vi "EM9636M系列_主VI.vi"() -> ()   [LabVIEW 2016]
uses:
  <vilib>/Modbus/subvis/Modbus API/Modbus API.lvclass/Modbus API.ctl
  <vilib>/Modbus/subvis/Transmission Data Unit (ADU)/Transmission Data Unit/Transmission Data Unit.lvclass/Transmission Data Unit.ctl
  <vilib>/Modbus/master/Data Access/Unit ID/Set Unit ID Property.vi
  <vilib>/Modbus/subvis/Transmission Data Unit (ADU)/Transmission Data Unit/Data Access/Unit ID/Write Unit ID.vi
  <vilib>/Modbus/subvis/Modbus API/Read Transmission Data Unit.vi
  <vilib>/Modbus/subvis/Modbus API/Write Transmission Data Unit.vi
  <vilib>/Modbus/master/Modbus Master.lvclass
  <vilib>/Utility/NIReport.llb/Append Text Table to Report (wrap).vi
  <vilib>/Modbus/master/Create Master Instance (Serial).vi
  <vilib>/Modbus/subvis/Transmission Data Unit (ADU)/Transmission Data Unit/Transmission Data Unit.lvclass
  <vilib>/Utility/NIReport.llb/NI_report.lvclass
  <vilib>/ptbypt/NI_PtbyPt.lvlib
  <vilib>/Utility/miscctls.llb/LVRectTypeDef.ctl
panel:
  out "车型":string
  in  "簇 3":T1
  out "R3":dbl format="%#.2g"
  out "R2":dbl format="%#.2g"
  out "R1":dbl format="%#.2g"
  out "D6":dbl format="%#.2g"
  out "D5":dbl format="%#.2g"
  out "D4":dbl format="%#.2g"
  out "D3":dbl format="%#.2g"
  out "D2":dbl format="%#.2g"
  out "D1":dbl format="%#.2g"
  in  "簇":T1
  out "数据":T2(array[cluster])
  out "comcnt":u16
  out "对话框":bool
  out "到期了":bool
  out "变频6":bool
  out "变频5":bool
  out "变频4":bool
  out "变频3":bool
  out "变频2":bool
  out "变频1":bool
  in  "加载电机右下正反转":bool
  out "加载右下转矩监控":i16 format="%#.0f"
  in  "加载电机右下启动":bool caption="停止"
  out "加载电机右下母线电流":dbl
  out "加载电机右下母线电压":dbl
  out "加载转速右下监控":dbl
  in  "加载电机右下转速给定":i32
  in  "加载电机右下停机":bool caption="停止"
  out "加载电机右下运行？":bool
  in  "加载电机右下转矩给定":i16
  out "加载电机左下运行？":bool
  in  "加载电机左下转速给定":i32
  out "加载左下转速监控":dbl
  out "加载电机左下母线电压":dbl
  out "加载电机左下母线电流":dbl
  out "加载左下转矩监控":i16
  in  "加载电机左下停机":bool caption="停止"
  in  "加载电机左下启动":bool caption="停止"
  in  "加载电机左下正反转":bool
  in  "加载电机左下转矩给定":i16
  in  "加载电机右上正反转":bool
  out "加载转矩右上监控":i16 format="%#.0f"
  in  "加载电机右上启动":bool caption="停止"
  out "加载电机右上母线电流":dbl
  out "加载电机右上母线电压":dbl
  out "加载右上转速监控":dbl
  in  "加载电机右上转速给定":i32
  in  "加载电机右上停机":bool caption="停止"
  out "加载电机右上运行？":bool
  in  "加载电机右上转矩给定":i16
  out "加载电机左上运行？":bool
  in  "加载电机左上转速给定":i32
  out "加载左上转速监控":dbl
  out "加载电机左上母线电压":dbl
  out "加载电机左上母线电流":dbl
  out "加载左上转矩监控":i16
  in  "加载电机左上停机":bool caption="停止"
  in  "加载电机左上启动":bool caption="停止"
  in  "加载电机左上正反转":bool
  in  "加载电机左上转矩给定":i16
  in  "驱动电机上正反转":bool
  out "驱动转矩上监控":i16 format="%#.0f"
  in  "驱动电机上转矩给定":i16
  in  "驱动电机上启动":bool caption="停止"
  out "驱动电机上母线电流":dbl
  out "驱动电机上母线电压":dbl
  out "驱动上转速监控":dbl
  in  "驱动电机上转速给定":i16
  in  "驱动电机上停机":bool caption="停止"
  out "驱动电机上运行？":bool
  in  "驱动电机下正反转":bool
  out "驱动转矩下监控":i16 format="%#.0f"
  in  "驱动电机下转矩给定":i16
  in  "驱动电机下启动":bool caption="停止"
  out "驱动电机下母线电流":dbl
  out "驱动电机下母线电压":dbl
  out "驱动转速下监控":dbl
  in  "驱动电机转速下给定":i16
  in  "驱动电机下停机":bool caption="停止"
  out "驱动电机下运行？":bool
  out "轮询耗时":u32
  out "数值":i32
  out "对话框传递":bool
  out "超温报警":bool
  out "遥控器通讯":bool
  out "变频串口":bool
  in  "加载电机复位":bool caption="停止"
  out "变频器":bool
  out "前右":bool[](array[boolean])
  out "前左":bool[](array[boolean])
  out "中右":bool[](array[boolean])
  out "中左":bool[](array[boolean])
  out "后右":bool[](array[boolean])
  out "后左":bool[](array[boolean])
  in  "倒计时间S":dbl=600.0
  out "错误输出 7":errorcluster caption="错误输出"
  out "确认输入布尔":bool
  out "等待进车布尔":bool
  out "Config":T9={"DevType"=2, "DevIndex"=0, "CanIndex"=0, "VCI_INIT_CONFIG"={"AccCode"=0, "AccMask"=0, "InitFlag"=0, "Fliter"=0, "Timing0"=0, "Timing1"=0, "Mode"=0}} {"DevType" items=["USB-CAN"=3, "USB-CAN2"=4]; "CanIndex" items=["通道1", "通道2"]; "VCI_INIT_CONFIG"."Fliter" items=["接收所有类型"=3, "只接收标准帧"=4, "只接收扩展帧"=7]; "VCI_INIT_CONFIG"."Mode" items=["正常工作", "自测模式（环回）", "仅侦听模式"]; "VCI_INIT_CONFIG"."InitFlag" items=["使用Flash参数", "使用界面设置参数"]}
  in  "D1扭矩给定":i16=500
  in  "D2扭矩给定":i16=1000
  in  "D3扭矩给定":i16=1500
  in  "D4扭矩给定":i16=2000
  in  "D5扭矩给定":i16=3500
  in  "D6扭矩给定":i16=4000
  in  "R1扭矩给定":i16=500
  in  "R2扭矩给定":i16=1000
  in  "R3扭矩给定":i16=1500
  out "发送左侧字符":bool
  in  "Close":bool
  in  "Open 2":bool
  in  "AD开始采集 2":bool
  in  "AD开始采集":bool
  out "输出数组右":dbl[][](array[numeric])
  out "输出数组左":dbl[][](array[numeric])
  out "采集卡右":bool
  out "采集卡左":bool
  out "Open":bool
  out "close2":bool
  out "close":bool
  out "当前实验时间":string
  out "元素 2":bool
  out "元素":bool
  out "元素 4":bool
  out "元素 3":bool
  in  "速度温度":string[][](array[string]) caption="文本数据"
  out "实验基本信息":string[][](array[string])
  out "字符布尔":bool
  in  "Reset 9":bool caption="重置"
  in  "Reset 8":bool caption="重置"
  in  "Reset 7":bool caption="重置"
  in  "Reset 6":bool caption="重置"
  in  "Reset 5":bool caption="重置"
  in  "Reset 4":bool caption="重置"
  in  "Reset 3":bool caption="重置"
  in  "Reset 2":bool caption="重置"
  in  "Reset":bool caption="重置"
  out "R3平均速度":dbl
  out "R2平均速度":dbl
  out "R1平均速度":dbl
  out "D6平均速度":dbl
  out "D5平均速度":dbl
  out "D4平均速度":dbl
  out "D3平均速度":dbl
  out "D2平均速度":dbl
  out "平均速度数组":dbl[](array[numeric])
  out "D1平均速度":dbl
  out "停止布尔 2":bool
  out "停止布尔":bool
  out "启动布尔":bool
  out "485启动给遥控器布尔":bool
  in  "左5字符":u8=85 format="%x"
  in  "左4字符":u8=85 format="%x"
  in  "左3字符":u8=85 format="%x"
  in  "左2字符":u8=85 format="%x"
  in  "左1字符":u8=85 format="%x"
  out "布尔数组 2":bool[](array[boolean])
  out "布尔数组":bool[](array[boolean])
  in  "kBaudRate":u8(ring)=10 caption="波特率" items=["5k bps"=1, "10k bps"=2, "20k bps"=3, "40k bps"=4, "50k bps"=5, "80k bps"=6, "100k bps"=7, "125k bps"=8, "200k bps"=9, "250k bps"=10, "400k bps"=11, "500k bps"=12, "666k bps"=13, "800k bps"=14, "1000k bps"=15, "33.33k bps"=16, "66.66k bps"=17, "83.33k bps"=18]
  in  "Channel":T4 caption="CAN通道" items=["通道1", "通道2"]
  in  "DevType":T3=2 caption="设备类型" items=["USB-CAN"=2, "USB-CAN2"=3]
  out "中间数组":string[](array[string])
  in  "数值 2":dbl
  out "系统时间 2":string="系统时间"
  in  "ID_VCU_MCU_1 8":u32=522 format="0x%x"
  in  "ID_VCU_MCU_2 5":u32=522 format="0x%x"
  in  "ID_VCU_MCU_33 4":u32=522 format="0x%x"
  in  "ID_VCU_MCU_1 7":u32=522 format="0x%x"
  in  "0byte 13":u8=64 format="%x"
  in  "1byte 13":u8=6 format="%x"
  in  "2byte 13":u8=80 format="%x"
  in  "3byte 13":u8=111 format="%x"
  in  "4byte 13":u8=119 format="%x"
  in  "5byte 13":u8=101 format="%x"
  in  "6byte 13":u8=114 format="%x"
  in  "7byte 13":u8=32 format="%x"
  in  "0byte 14":u8=70 format="%x"
  in  "1byte 14":u8=2 format="%x"
  in  "2byte 14":u8=32 format="%x"
  in  "3byte 14":u8=32 format="%x"
  in  "4byte 14":u8 format="%x"
  in  "5byte 14":u8 format="%x"
  in  "6byte 14":u8 format="%x"
  in  "7byte 14":u8 format="%x"
  in  "0byte 15":u8=96 format="%x"
  in  "1byte 15":u8=6 format="%x"
  in  "2byte 15":u8=84 format="%x"
  in  "3byte 15":u8=85 format="%x"
  in  "4byte 15":u8=114 format="%x"
  in  "5byte 15":u8=113 format="%x"
  in  "6byte 15":u8=117 format="%x"
  in  "7byte 15":u8=101 format="%x"
  in  "0byte 16":u8=102 format="%x"
  in  "1byte 16":u8=2 format="%x"
  in  "2byte 16":u8=32 format="%x"
  in  "3byte 16":u8=32 format="%x"
  in  "4byte 16":u8 format="%x"
  in  "5byte 16":u8 format="%x"
  in  "6byte 16":u8 format="%x"
  in  "7byte 16":u8 format="%x"
  in  "ID_VCU_MCU_1 6":u32=522 format="0x%x"
  in  "ID_VCU_MCU_2 4":u32=522 format="0x%x"
  in  "ID_VCU_MCU_33 3":u32=522 format="0x%x"
  in  "ID_VCU_MCU_1 5":u32=522 format="0x%x"
  in  "0byte 5":u8=16 format="%x"
  in  "1byte 5":u8=6 format="%x"
  in  "2byte 5":u8=85 format="%x"
  in  "3byte 5":u8=85 format="%x"
  in  "4byte 5":u8=85 format="%x"
  in  "5byte 5":u8=85 format="%x"
  in  "6byte 5":u8=85 format="%x"
  in  "7byte 5":u8=85 format="%x"
  in  "0byte 6":u8=86 format="%x"
  in  "1byte 6":u8=2 format="%x"
  in  "2byte 6":u8=75 format="%x"
  in  "3byte 6":u8=119 format="%x"
  in  "4byte 6":u8 format="%x"
  in  "5byte 6":u8 format="%x"
  in  "6byte 6":u8 format="%x"
  in  "7byte 6":u8 format="%x"
  in  "0byte 7":u8=48 format="%x"
  in  "1byte 7":u8=6 format="%x"
  in  "2byte 7":u8=85 format="%x"
  in  "3byte 7":u8=85 format="%x"
  in  "4byte 7":u8=85 format="%x"
  in  "5byte 7":u8=85 format="%x"
  in  "6byte 7":u8=85 format="%x"
  in  "7byte 7":u8=85 format="%x"
  in  "0byte 8":u8=118 format="%x"
  in  "1byte 8":u8=2 format="%x"
  in  "2byte 8":u8=78 format="%x"
  in  "3byte 8":u8=109 format="%x"
  in  "4byte 8":u8 format="%x"
  in  "5byte 8":u8 format="%x"
  in  "6byte 8":u8 format="%x"
  in  "7byte 8":u8 format="%x"
  in  "ID_VCU_MCU_1 2":u32=522 format="0x%x"
  in  "ID_VCU_MCU_33":u32=522 format="0x%x"
  in  "ID_VCU_MCU_2 2":u32=522 format="0x%x"
  in  "ID_VCU_MCU_1":u32=522 format="0x%x"
  in  "ID_VCU_MCU_1 4":u32=522 format="0x%x"
  in  "ID_VCU_MCU_2 3":u32=522 format="0x%x"
  in  "ID_VCU_MCU_33 2":u32=522 format="0x%x"
  in  "ID_VCU_MCU_1 3":u32=522 format="0x%x"
  in  "0byte 9":u8 format="%x"
  in  "1byte 9":u8=6 format="%x"
  in  "2byte 9":u8=71 format="%x"
  in  "3byte 9":u8=101 format="%x"
  in  "4byte 9":u8=97 format="%x"
  in  "5byte 9":u8=114 format="%x"
  in  "6byte 9":u8=32 format="%x"
  in  "7byte 9":u8=32 format="%x"
  in  "0byte 10":u8=6 format="%x"
  in  "1byte 10":u8=2 format="%x"
  in  "2byte 10":u8=32 format="%x"
  in  "3byte 10":u8=32 format="%x"
  in  "4byte 10":u8 format="%x"
  in  "5byte 10":u8 format="%x"
  in  "6byte 10":u8 format="%x"
  in  "7byte 10":u8 format="%x"
  in  "0byte 11":u8=32 format="%x"
  in  "1byte 11":u8=6 format="%x"
  in  "2byte 11":u8=83 format="%x"
  in  "3byte 11":u8=112 format="%x"
  in  "4byte 11":u8=101 format="%x"
  in  "5byte 11":u8=101 format="%x"
  in  "6byte 11":u8=100 format="%x"
  in  "7byte 11":u8=32 format="%x"
  in  "0byte 12":u8=38 format="%x"
  in  "1byte 12":u8=2 format="%x"
  in  "2byte 12":u8=32 format="%x"
  in  "3byte 12":u8=32 format="%x"
  in  "4byte 12":u8 format="%x"
  in  "5byte 12":u8 format="%x"
  in  "6byte 12":u8 format="%x"
  in  "7byte 12":u8 format="%x"
  in  "0byte 4":u8=54 format="%x"
  in  "1byte 4":u8=2 format="%x"
  in  "2byte 4":u8=80 format="%x"
  in  "3byte 4":u8=109 format="%x"
  in  "4byte 4":u8 format="%x"
  in  "5byte 4":u8 format="%x"
  in  "6byte 4":u8 format="%x"
  in  "7byte 4":u8 format="%x"
  in  "0byte 3":u8=48 format="%x"
  in  "1byte 3":u8=6 format="%x"
  in  "2byte 3":u8=85 format="%x"
  in  "3byte 3":u8=85 format="%x"
  in  "4byte 3":u8=85 format="%x"
  in  "5byte 3":u8=85 format="%x"
  in  "6byte 3":u8=85 format="%x"
  in  "7byte 3":u8=82 format="%x"
  in  "0byte 2":u8=22 format="%x"
  in  "1byte 2":u8=2 format="%x"
  in  "2byte 2":u8=32 format="%x"
  in  "3byte 2":u8=32 format="%x"
  in  "4byte 2":u8 format="%x"
  in  "5byte 2":u8 format="%x"
  in  "6byte 2":u8 format="%x"
  in  "7byte 2":u8 format="%x"
  out "选项卡控件 4":enum32{"VCU控制", "CAN基本操作"}(tab)
  in  "Clear":bool
  in  "Mode":T8 caption="工作模式" items=["正常工作", "仅侦听模式", "自测模式（环回）"]
  in  "Fliter":T7=1 items=["接收所有类型"=1, "只接收标准帧"=2, "只接收扩展帧"=3]
  in  "AccMask":u32=4294967295 caption="接收屏蔽码" format="%08x"
  in  "AccCode":u32 caption="接收过滤码" format="%08x"
  out "SendCnt":u32 caption="发送统计"
  out "RecvCnt":u32 caption="接收统计"
  in  "RcvEnable":bool=TRUE
  in  "list":i32(listbox)
  in  "Send":bool
  in  "ID":u32 format="0x%x"
  in  "Type":u8(ring) items=["数据帧", "远程帧"]
  in  "Format":u8(ring) items=["标准帧", "扩展帧"]
  in  "Data":string="01 00"
  in  "0byte":u8=16 format="%x"
  in  "1byte":u8=6 format="%x"
  in  "2byte":u8=85 format="%x"
  in  "3byte":u8=85 format="%x"
  in  "4byte":u8=85 format="%x"
  in  "5byte":u8=85 format="%x"
  in  "6byte":u8=85 format="%x"
  in  "7byte":u8=85 format="%x"
  in  "InitFlag":T6=1 caption="初始化参数" items=["使用Flash参数", "使用界面设置参数"]
  in  "选项卡控件 3":enum32{"数据监视", "查看数据"}(tab)
  in  "确认换挡":bool
  in  "重新选档档位":T10(ring)
  out "前右":bool
  out "中右":bool
  out "后右":bool
  out "前左":bool
  out "中左":bool
  out "后左":bool
  out "R3S":dbl format="%#.2g"
  out "R2S":dbl format="%#.2g"
  out "R1S":dbl format="%#.2g"
  out "D6S":dbl format="%#.2g"
  out "D5S":dbl format="%#.2g"
  out "D4S":dbl format="%#.2g"
  out "D3S":dbl format="%#.2g"
  out "D2S":dbl format="%#.2g"
  out "D1S":dbl format="%#.2g"
  in  "刷新参数":bool
  out "LED屏幕信息":string
  in  "高级参数":bool
  in  "重新实验":bool
  in  "生成报表":bool
  in  "确认输入":bool
  in  "遥控器按钮确认":bool
  out "总实验时间":string
  out "前右":dbl format="%#.2g"
  out "前左":dbl format="%#.2g"
  out "中右":dbl
  out "中左":dbl format="%#.2g"
  out "后右":dbl format="%#.2g"
  out "后左":dbl format="%#.2g"
  out "后右":dbl format="%#.2g"
  out "后左":dbl format="%#.2g"
  out "中右":dbl format="%#.2g"
  out "中左":dbl format="%#.2g"
  out "前右":dbl format="%#.2g"
  out "前左":dbl format="%#.2g"
  out "环境温度标定":dbl format="%#.2g"
  out "波形图表":dynamicdata(graph)
  in  "操作者":string
  out "加载扭矩N.M(单个）":dbl
  out "当前试验档位":string
  in  "试验车型":u16(ring) items=["SG21-3", "SG14", "SG16-3", "SG18-3"]
  out "车速":dbl(knob) scale=-30.0..30.0
  in  "试验车编号":string
  in  "发动机编号":string
  out "加载功率":dbl(knob) scale=0.0..30.0
  in  "试验开始":bool caption="停止"
  in  "停止":bool
  out "液压油箱温度标定":dbl format="%#.2g"
  out "变矩器出口温度标定":dbl format="%#.2g"
  out "右前轮轴承温度标定":dbl format="%#.2g"
  out "左前轮轴承温度标定":dbl format="%#.2g"
  out "振动泵压力":dbl format="%#.2g"
  out "转向泵压力":dbl format="%#.2g"
  in  "密码输入":string
  out "SG14百分比":dbl
  out "SG16-3百分比":dbl
  out "SG18-3百分比":dbl
  out "D1 act":dbl format="%#.2g"
  out "D2 act":dbl format="%#.2g"
  out "R3 act":dbl format="%#.2g"
  out "R2 act":dbl format="%#.2g"
  out "R1 act":dbl format="%#.2g"
  out "D6 act":dbl format="%#.2g"
  out "D5 act":dbl format="%#.2g"
  out "D4 act":dbl format="%#.2g"
  out "D3 act":dbl format="%#.2g"
  out "数值 3":i32
  out "前右电机右轴承振动":dbl
  out "前右电机左轴承振动":dbl
  out "前右滚筒右轴承振动":dbl
  out "前右滚筒左轴承振动":dbl
  out "后左滚筒右振动":dbl
  out "后左滚筒左振动":dbl
  out "中右电机右振动":dbl
  out "中右电机左振动":dbl
  out "中右滚筒右振动":dbl
  out "中右滚筒左振动":dbl
  out "中左电机右轴承振动":dbl
  out "中左电机左轴承振动":dbl
  out "中左滚筒右轴承振动":dbl
  out "中左滚筒左轴承振动":dbl
  out "前左电机右轴承振动":dbl
  out "前左电机左轴承振动":dbl
  out "前左滚筒右轴承振动":dbl
  out "前左滚筒左轴承振动":dbl
  out "后右电机右振动":dbl
  out "后右电机左振动":dbl
  out "后右滚筒右振动":dbl
  out "后右滚筒左振动":dbl
  out "后左电机右振动":dbl
  out "后左电机左振动":dbl
  out "后右电机绕组":dbl
  out "后右电机右轴承":dbl
  out "后右滚筒左轴承":dbl
  out "后左滚筒右轴承":dbl
  out "后右滚筒左轴承":dbl
  out "后左电机绕组":dbl
  out "后左电机右轴承":dbl
  out "后左电机左轴承":dbl
  out "后左滚筒右轴承":dbl
  out "后左滚筒左轴承":dbl
  out "中右电机绕组":dbl
  out "中右电机右轴承":dbl
  out "中右电机左轴承":dbl
  out "中右滚筒右轴承":dbl
  out "中右滚筒左轴承":dbl
  out "中左电机绕组":dbl
  out "中左电机右轴承":dbl
  out "中左电机左轴承":dbl
  out "中左滚筒右轴承":dbl
  out "中左滚筒左轴承":dbl
  out "前右电机绕组":dbl
  out "前右电机右轴承":dbl
  out "前右滚筒左轴承":dbl
  out "前左滚筒右轴承":dbl
  out "前右滚筒左轴承":dbl
  out "前左电机绕组":dbl
  out "前左电机右轴承":dbl
  out "前左电机左轴承":dbl
  out "前左滚筒右轴承":dbl
  out "前左滚筒左轴承":dbl
  out "错误输出 6":errorcluster caption="错误输出"
  out "AD均值数据 2":dbl[](array[numeric])
  in  "M系列PWM停止 2":bool
  in  "编码器清零 2":bool
  in  "DA输出 2":bool
  in  "DA输出范围 2":i32(ring) items=["±10V", "±5V", "0~10V（默认）", "0~5V", "0~20mA"]
  in  "CH1 2":i16(slide) scale=0.0..10000.0
  in  "CH3 2":i16(slide) scale=0.0..10000.0
  in  "CH4 2":i16(slide) scale=0.0..10000.0
  in  "CH2 2":i16(slide) scale=0.0..10000.0
  in  "设定输出脉冲个数 2":u32
  in  "M系列PWM输出 2":bool
  in  "AD停止采集 2":bool
  out "布尔 2":bool
  in  "通道频率Hz 2":dbl=10000.0 min=1000.0 max=100000.0 step=10.0
  in  "组频率Hz 2":dbl=500.0
  in  "单双端 2":i32(ring) items=["单端", "双端"]
  in  "AD终止通道 2":i32=32
  in  "AD起始通道 2":i32=1
  in  "增益 2":i32(ring) items=["无增益", "2倍增益", "5倍增益", "10倍增益"]
  in  "伪同步 2":i32(ring) items=["非伪同步", "伪同步"]
  in  "时钟源 2":i32(ring) items=["内时钟", "外时钟"]
  out "每次总数据量 2":i32
  out "通道数量 2":i32
  in  "AD范围 2":enum16{"-10~+10V", "-5V~+5V", "0~10V", "0~5V"}(ring)=enum."0~10V"
  out "每通道数据量 2":i32
  out "编码器AB值 2":i32[](array[numeric])
  out "编码器过零值 2":i16[](array[numeric])
  out "错误输出 5":errorcluster caption="错误输出3"
  out "错误输出 4":errorcluster caption="错误输出2"
  out "设备句柄 2":i32=1
  in  "选项卡控件 2":enum32{"AD数值显示", "数字量I/O", "(标准)PWM", "计数器（测频）"}(tab)
  in  "设置开关量方向 3":bool
  out "数组 5":dbl[](array[numeric])=[1.0, 2.0, 3.0, 4.0, 5.0, 6.0, 7.0, 8.0]
  out "数组 6":dbl[](array[numeric])=[1.0, 2.0, 3.0, 4.0, 5.0, 6.0, 7.0, 8.0]
  in  "光隔离输出 2":bool[](array[boolean])=[FALSE, FALSE, FALSE, FALSE, FALSE, FALSE, FALSE, FALSE]
  out "光隔离输入 2":bool[](array[boolean])
  in  "设置开关量方向 2":cluster{"IO1~IO8":i8, "IO9~IO16":i8}={"IO1~IO8"=1, "IO9~IO16"=1} {"IO9~IO16" items=["输入", "输出"]; "IO1~IO8" items=["输入", "输出"]}
  out "数组 7":i8[](array[numeric])
  in  "可编程数字量I/O 2":T11
  out "可编程数字量I/O(映射控件)--得到所有通道开关量值 2":T11
  in  "PWM输出 2":bool
  in  "PWM停止 2":bool
  in  "频率1 2":dbl=1000.0
  in  "占空比(0~1) 6":dbl=0.5
  out "实际频率 6":dbl
  out "实际占空比 6":dbl
  in  "频率2 2":dbl=5000.0
  in  "占空比(0~1) 5":dbl=0.5
  out "实际频率 5":dbl
  out "实际占空比 5":dbl
  in  "频率3 2":dbl=100000.0
  in  "占空比(0~1) 4":dbl=0.5
  out "实际频率 4":dbl
  out "实际占空比 4":dbl
  in  "开启计数 2":bool
  in  "计数器清零 2":bool
  in  "工作方式 2":u16(ring)=1 items=["计数", "测频"]
  out "计数/测频（Hz）值 2":dbl[](array[numeric])
  in  "编码器清零":bool
  out "编码器AB值":i32[](array[numeric])
  out "编码器过零值":i16[](array[numeric])
  in  "设定输出脉冲个数":u32
  in  "M系列PWM输出":bool
  in  "M系列PWM停止":bool
  in  "CH4":i16(slide) scale=0.0..10000.0
  in  "CH3":i16(slide) scale=0.0..10000.0
  in  "CH2":i16(slide) scale=0.0..10000.0
  in  "CH1":i16(slide) scale=0.0..10000.0
  in  "DA输出":bool
  in  "DA输出范围":i32(ring) items=["±10V", "±5V", "0~10V（默认）", "0~5V", "0~20mA"]
  out "每通道数据量":i32
  out "AD均值数据":dbl[](array[numeric])
  out "布尔":bool
  in  "AD停止采集":bool
  out "错误输出 3":errorcluster caption="错误输出3"
  out "错误输出 2":errorcluster caption="错误输出2"
  in  "选项卡控件":enum32{"AD数值显示", "数字量I/O", "(标准)PWM", "计数器（测频）"}(tab)
  out "变频故障1":bool
  out "变频故障2":bool
  out "变频故障 3":bool
  out "变频故障 4":bool
  out "变频故障5":bool
  out "变频故障 6":bool
  in  "设置开关量方向":bool
  out "数组 3":dbl[](array[numeric])=[1.0, 2.0, 3.0, 4.0, 5.0, 6.0, 7.0, 8.0]
  out "数组 2":dbl[](array[numeric])=[1.0, 2.0, 3.0, 4.0, 5.0, 6.0, 7.0, 8.0]
  in  "光隔离输出":bool[](array[boolean])=[FALSE, FALSE, FALSE, FALSE, FALSE, FALSE, FALSE, FALSE]
  out "光隔离输入":bool[](array[boolean])
  in  "设置开关量方向":cluster{"IO1~IO8":i8, "IO9~IO16":i8}={"IO1~IO8"=1, "IO9~IO16"=1} {"IO9~IO16" items=["输入", "输出"]; "IO1~IO8" items=["输入", "输出"]}
  out "数组 4":i8[](array[numeric])
  in  "可编程数字量I/O":T11
  out "可编程数字量I/O(映射控件)--得到所有通道开关量值":T11
  in  "PWM输出":bool
  in  "PWM停止":bool
  in  "频率1":dbl=1000.0
  in  "占空比(0~1)":dbl=0.5
  out "实际频率":dbl
  out "实际占空比":dbl
  in  "频率2":dbl=5000.0
  in  "占空比(0~1) 2":dbl=0.5
  out "实际频率 2":dbl
  out "实际占空比 2":dbl
  in  "频率3":dbl=100000.0
  in  "占空比(0~1) 3":dbl=0.5
  out "实际频率 3":dbl
  out "实际占空比 3":dbl
  in  "开启计数":bool
  in  "计数器清零":bool
  in  "工作方式":u16(ring)=1 items=["计数", "测频"]
  out "计数/测频（Hz）值":dbl[](array[numeric])
  in  "AD范围":enum16{"-10~+10V", "-5V~+5V", "0~10V", "0~5V"}(ring)=enum."0~10V"
  out "通道数量":i32
  out "设备句柄":i32=1
  out "错误输出":errorcluster
  out "每次总数据量":i32
  in  "时钟源":i32(ring) items=["内时钟", "外时钟"]
  in  "伪同步":i32(ring) items=["非伪同步", "伪同步"]
  in  "增益":i32(ring) items=["无增益", "2倍增益", "5倍增益", "10倍增益"]
  in  "AD起始通道":i32=1
  in  "AD终止通道":i32=32
  in  "单双端":i32(ring) items=["单端", "双端"]
  in  "组频率Hz":dbl=500.0
  in  "通道频率Hz":dbl=10000.0 min=1000.0 max=100000.0 step=10.0
  in  "数据端口":i32=8001
  in  "命令端口":i32=8000
  in  "IP地址":string="192.168.1.125"
  # "加载电机右上"
  # "驱动电机上"
  # "加载电机左上"
  # "r/min"
  # "r/min"
  # "r/min"
  # "转速"
  # "给定"
  # "转速"
  # "给定"
  # "转速"
  # "给定"
  # "给定"
  # "Nm"
  # "Nm"
  # "Nm"
  # "转矩"
  # "转矩"
  # "给定"
  # "转矩"
  # "给定"
  # "山推平地机实验台"
  # "电压"
  # "电流"
  # "电压"
  # "电流"
  # "电压"
  # "V"
  # "电流"
  # "A"
  # "A"
  # "V"
  # "A"
  # "V"
  # "遥控器"
  # "变频器"
  # "采集卡左"
  # "采集卡右"
  # "超温报警"
  # "正转"
  # "反转"
  # "正转"
  # "正转"
  # "反转"
  # "反转"
  # "加载电机右下"
  # "驱动电机下"
  # "加载电机左下"
  # "r/min"
  # "r/min"
  # "r/min"
  # "转速"
  # "给定"
  # "转速"
  # "给定"
  # "转速"
  # "给定"
  # "给定"
  # "Nm"
  # "Nm"
  # "Nm"
  # "转矩"
  # "转矩"
  # "给定"
  # "转矩"
  # "给定"
  # "电压"
  # "电流"
  # "电压"
  # "电流"
  # "电压"
  # "V"
  # "电流"
  # "A"
  # "V"
  # "A"
  # "V"
  # "A"
  # "正转"
  # "反转"
  # "正转"
  # "正转"
  # "反转"
  # "反转"
  # "D1"
  # "D6扭矩给定"
  # "~"
  # "R1"
  # "R3扭矩给定"
  # "~"
  # "EM9636M系列--LabView例程"
  # "CH1"
  # "CH2"
  # "如果设为0，则表示连续输出"
  # "CH1"
  # "CH2"
  # "位置传感器故障"
  # "过流"
  # "控制器过温"
  # "电机过温"
  # "欠压报警"
  # "过压报警"
  # "通讯故障"
  # "控制器高温"
  # "短路保护"
  # "严重欠压"
  # "超过峰值功率"
  # "超过最高限速"
  # "VCU故障"
  # "跛行状态"
  # "堵转保护"
  # "致命故障"
  # "车辆参数"
  # "设备参数"
  # "环境温度"
  # "前左"
  # "℃"
  # "℃"
  # "r/min"
  # "r/min"
  # "r/min"
  # "液压油箱温度"
  # "℃"
  # "前右"
  # "℃"
  # "r/min"
  # "r/min"
  # "r/min"
  # "变速箱温度"
  # "℃"
  # "中左"
  # "℃"
  # "右前轮轴承温度"
  # "中右"
  # "℃"
  # "℃"
  # "左前轮轴承温度"
  # "~"
  # "D1   R3/%"
  # "℃"
  # "后左"
  # "℃"
  # "~"
  # "D1   R3/S"
  # "Mp"
  # "工作泵压力"
  # "后右"
  # "℃"
  # "转向泵压力"
  # "Mp"
  # "前左滚筒左轴承"
  # "后左滚筒左轴承"
  # "℃"
  # "℃"
  # "后左电机左振动"
  # "前右滚筒左振动"
  # "前左滚筒右轴承"
  # "后左滚筒右轴承"
  # "℃"
  # "℃"
  # "后左电机右振动"
  # "前右滚筒右振动"
  # "前左电机左轴承"
  # "后左电机左轴承"
  # "℃"
  # "后右滚筒左振动"
  # "℃"
  # "前右电机左振动"
  # "前左电机右轴承"
  # "后左电机右轴承"
  # "℃"
  # "℃"
  # "后右滚筒右振动"
  # "前右电机右振动"
  # "前左电机绕组"
  # "后左电机绕组"
  # "后右电机左振动"
  # "℃"
  # "℃"
  # "前右滚筒左轴承"
  # "后右滚筒左轴承"
  # "后右电机右振动"
  # "℃"
  # "℃"
  # "前右滚筒右轴承"
  # "后右滚筒右轴承"
  # "前左滚筒左振动"
  # "℃"
  # "℃"
  # "前右电机左轴承"
  # "后右电机左轴承"
  # "前右滚筒右振动"
  # "℃"
  # "℃"
  # "前右电机右轴承"
  # "后右电机右轴承"
  # "前左电机左振动"
  # "℃"
  # "℃"
  # "前右电机绕组"
  # "后右电机绕组"
  # "℃"
  # "℃"
  # "前左电机右振动"
  # "中左滚筒左轴承"
  # "℃"
  # "中左滚筒左振动"
  # "中左滚筒右轴承"
  # "℃"
  # "中左滚筒右振动"
  # "中左电机左轴承"
  # "中左电机左振动"
  # "℃"
  # "中左电机右轴承"
  # "℃"
  # "中左电机右振动"
  # "中左电机绕组"
  # "℃"
  # "中右滚筒左振动"
  # "中右滚筒左轴承"
  # "中右滚筒右振动"
  # "℃"
  # "中右滚筒右轴承"
  # "中右电机左振动"
  # "℃"
  # "中右电机左轴承"
  # "中右电机右振动"
  # "℃"
  # "中右电机右轴承"
  # "后左滚筒左振动"
  # "℃"
  # "中右电机绕组"
  # "℃"
  # "后左滚筒右振动"
  # "通道3"
  # "通道1"
  # "通道2"
  # "频率，250Hz~500KHz\n占空比，0~1"
  # "通道3"
  # "通道1"
  # "通道2"
  # "频率，250Hz~500KHz\n占空比，0~1"
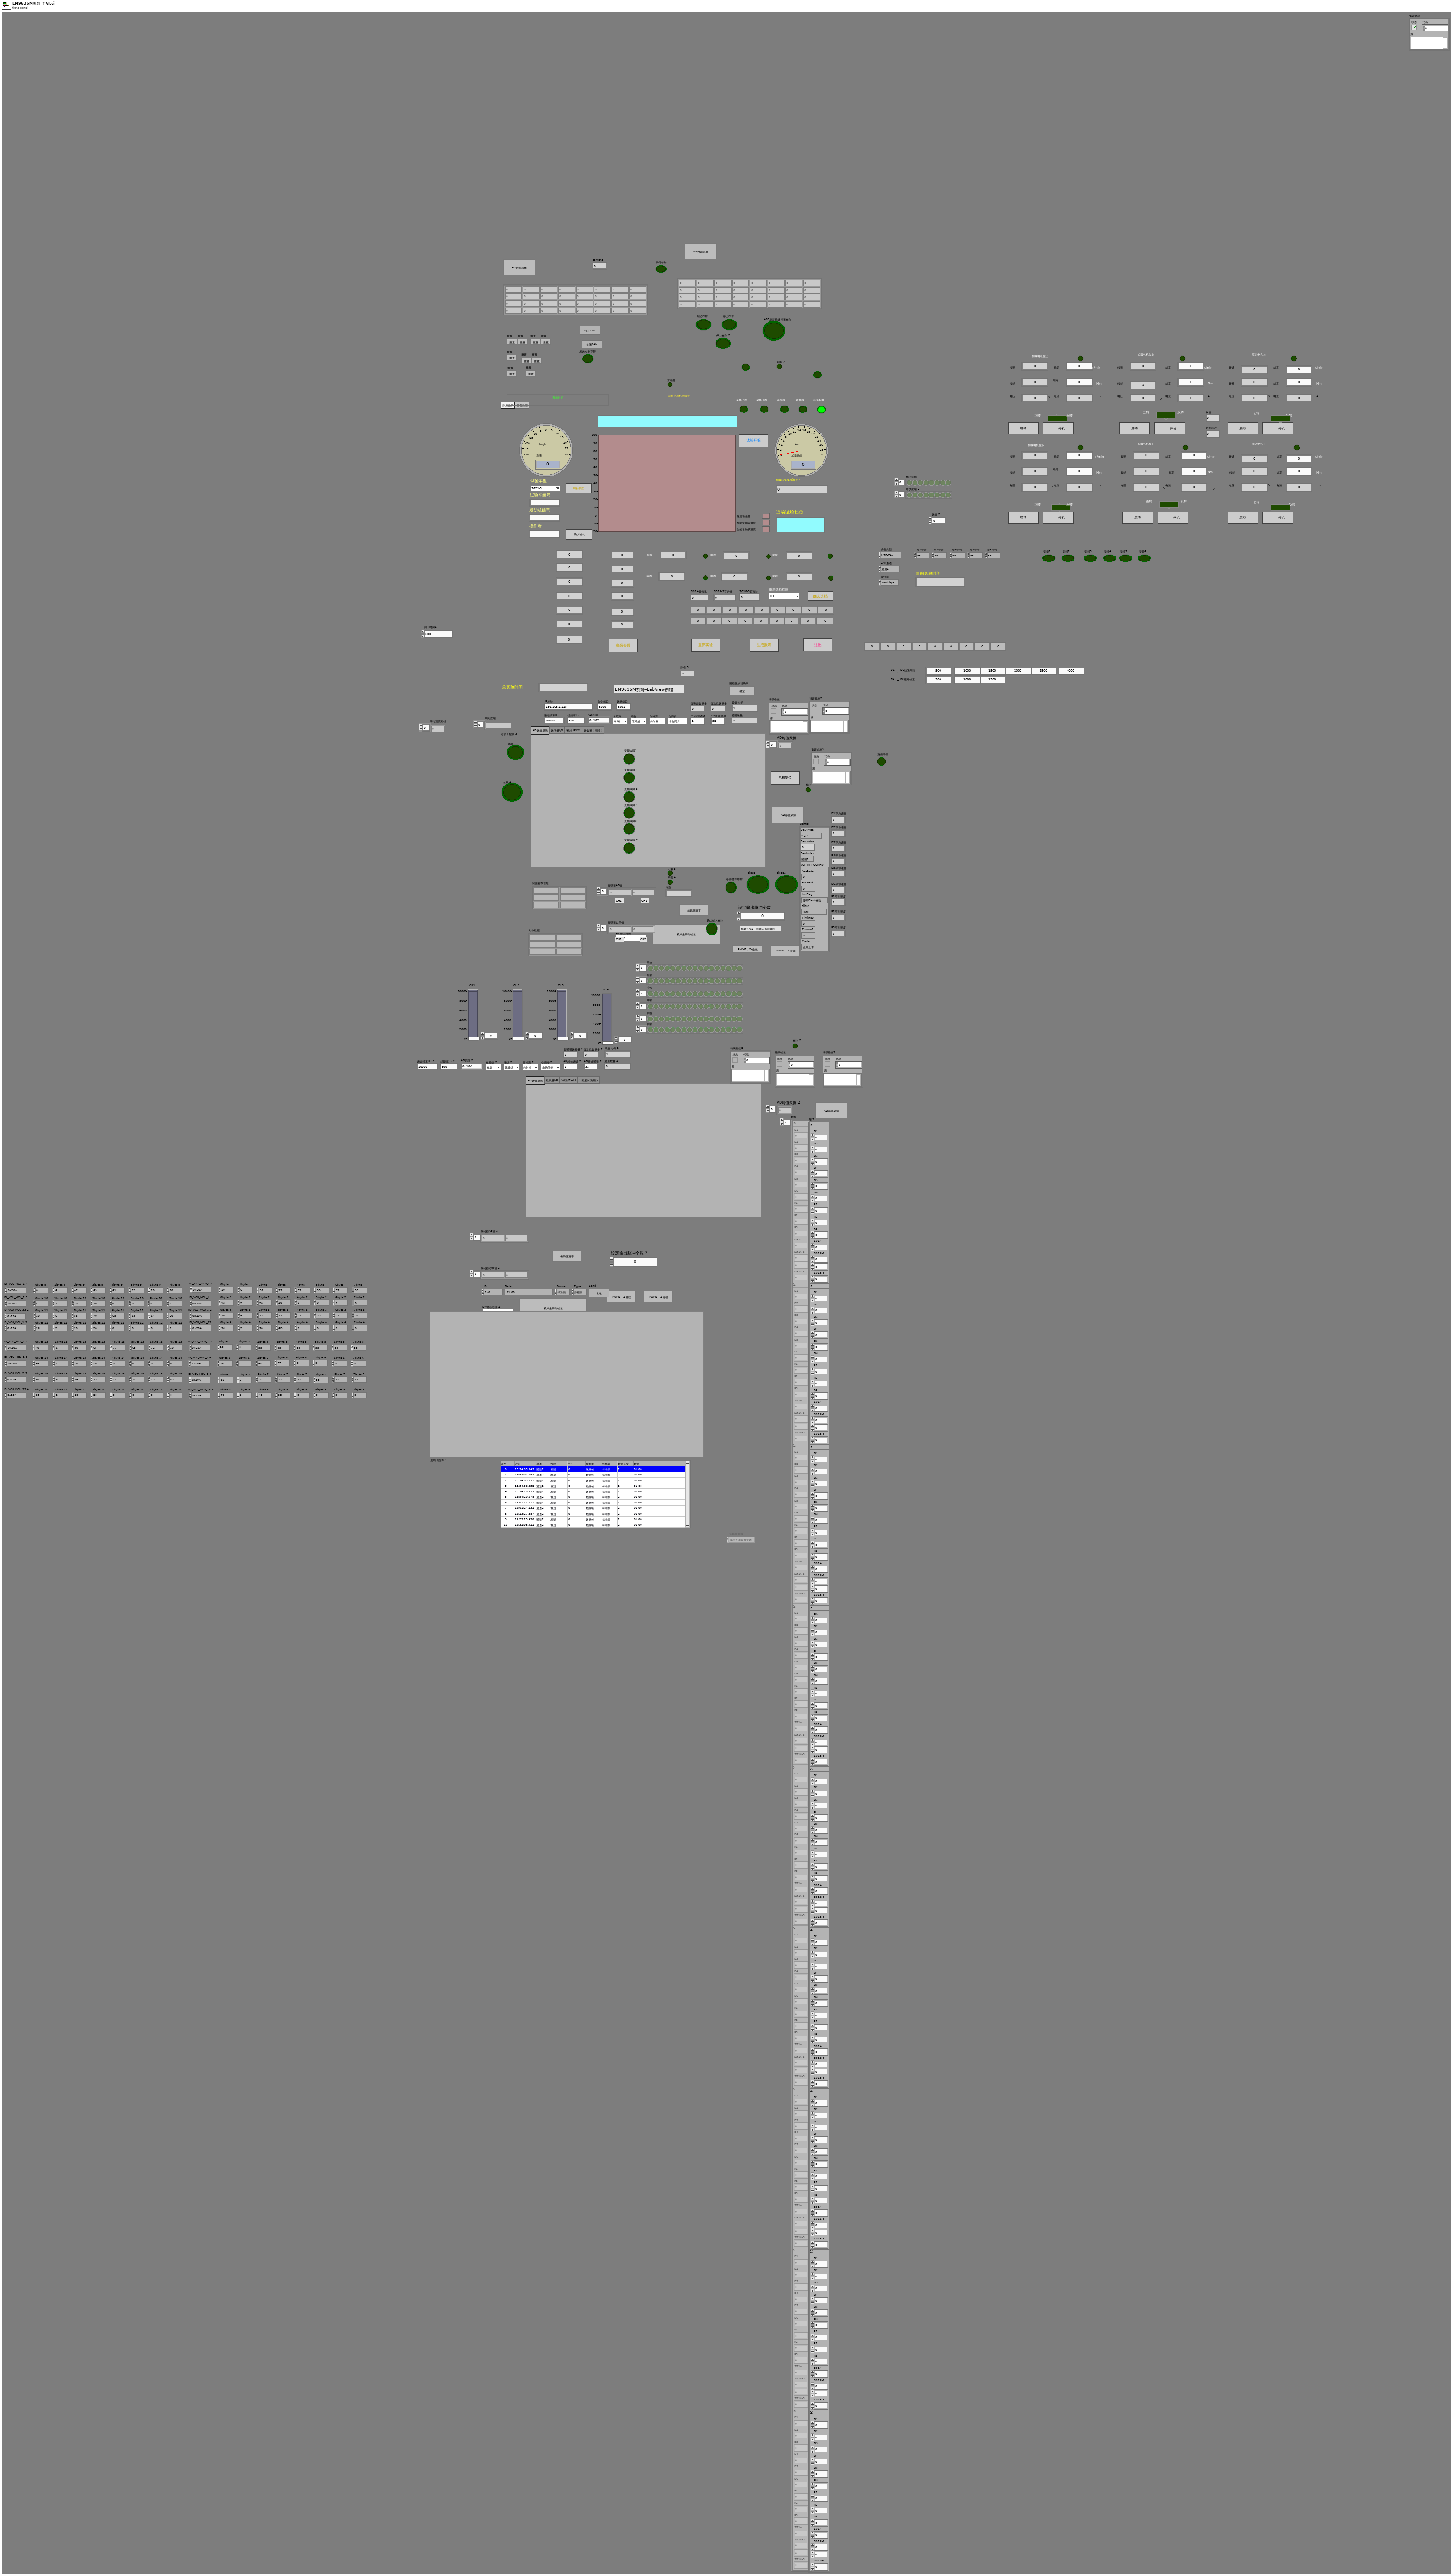
[diagram p1: front panel]
types:
  T1 = cluster{"[0]":cluster{"D1":dbl, "D2":dbl, "D3":dbl, "D4":dbl, "D5":dbl, "D6":dbl, "R1":dbl, "R2":dbl, "R3":dbl, "SG14":dbl, "SG16-3":dbl, dbl, "SG18-3 ":dbl}, "[1]":cluster{"D1":dbl, "D2":dbl, "D3":dbl, "D4":dbl, "D5":dbl, "D6":dbl, "R1":dbl, "R2":dbl, "R3":dbl, "SG14":dbl, "SG16-3":dbl, dbl, "SG18-3 ":dbl}, "[2]":cluster{"D1":dbl, "D2":dbl, "D3":dbl, "D4":dbl, "D5":dbl, "D6":dbl, "R1":dbl, "R2":dbl, "R3":dbl, "SG14":dbl, "SG16-3":dbl, dbl, "SG18-3 ":dbl}, "[3]":cluster{"D1":dbl, "D2":dbl, "D3":dbl, "D4":dbl, "D5":dbl, "D6":dbl, "R1":dbl, "R2":dbl, "R3":dbl, "SG14":dbl, "SG16-3":dbl, dbl, "SG18-3 ":dbl}, "[4]":cluster{"D1":dbl, "D2":dbl, "D3":dbl, "D4":dbl, "D5":dbl, "D6":dbl, "R1":dbl, "R2":dbl, "R3":dbl, "SG14":dbl, "SG16-3":dbl, dbl, "SG18-3 ":dbl}, "[5]":cluster{"D1":dbl, "D2":dbl, "D3":dbl, "D4":dbl, "D5":dbl, "D6":dbl, "R1":dbl, "R2":dbl, "R3":dbl, "SG14":dbl, "SG16-3":dbl, dbl, "SG18-3 ":dbl}, "[6]":cluster{"D1":dbl, "D2":dbl, "D3":dbl, "D4":dbl, "D5":dbl, "D6":dbl, "R1":dbl, "R2":dbl, "R3":dbl, "SG14":dbl, "SG16-3":dbl, dbl, "SG18-3 ":dbl}, "[7]":cluster{"D1":dbl, "D2":dbl, "D3":dbl, "D4":dbl, "D5":dbl, "D6":dbl, "R1":dbl, "R2":dbl, "R3":dbl, "SG14":dbl, "SG16-3":dbl, dbl, "SG18-3 ":dbl}, "[8]":cluster{"D1":dbl, "D2":dbl, "D3":dbl, "D4":dbl, "D5":dbl, "D6":dbl, "R1":dbl, "R2":dbl, "R3":dbl, "SG14":dbl, "SG16-3":dbl, dbl, "SG18-3 ":dbl}}
  T2 = cluster{"[0]":cluster{"D1":dbl, "D2":dbl, "D3":dbl, "D4":dbl, "D5":dbl, "D6":dbl, "R1":dbl, "R2":dbl, "R3":dbl, "SG14":dbl, "SG16-3":dbl, dbl, "SG18-3 ":dbl}, "[1]":cluster{"D1":dbl, "D2":dbl, "D3":dbl, "D4":dbl, "D5":dbl, "D6":dbl, "R1":dbl, "R2":dbl, "R3":dbl, "SG14":dbl, "SG16-3":dbl, dbl, "SG18-3 ":dbl}, "[2]":cluster{"D1":dbl, "D2":dbl, "D3":dbl, "D4":dbl, "D5":dbl, "D6":dbl, "R1":dbl, "R2":dbl, "R3":dbl, "SG14":dbl, "SG16-3":dbl, dbl, "SG18-3 ":dbl}, "[3]":cluster{"D1":dbl, "D2":dbl, "D3":dbl, "D4":dbl, "D5":dbl, "D6":dbl, "R1":dbl, "R2":dbl, "R3":dbl, "SG14":dbl, "SG16-3":dbl, dbl, "SG18-3 ":dbl}, "[4]":cluster{"D1":dbl, "D2":dbl, "D3":dbl, "D4":dbl, "D5":dbl, "D6":dbl, "R1":dbl, "R2":dbl, "R3":dbl, "SG14":dbl, "SG16-3":dbl, dbl, "SG18-3 ":dbl}, "[5]":cluster{"D1":dbl, "D2":dbl, "D3":dbl, "D4":dbl, "D5":dbl, "D6":dbl, "R1":dbl, "R2":dbl, "R3":dbl, "SG14":dbl, "SG16-3":dbl, dbl, "SG18-3 ":dbl}, "[6]":cluster{"D1":dbl, "D2":dbl, "D3":dbl, "D4":dbl, "D5":dbl, "D6":dbl, "R1":dbl, "R2":dbl, "R3":dbl, "SG14":dbl, "SG16-3":dbl, dbl, "SG18-3 ":dbl}, "[7]":cluster{"D1":dbl, "D2":dbl, "D3":dbl, "D4":dbl, "D5":dbl, "D6":dbl, "R1":dbl, "R2":dbl, "R3":dbl, "SG14":dbl, "SG16-3":dbl, dbl, "SG18-3 ":dbl}, "[8]":cluster{"D1":dbl, "D2":dbl, "D3":dbl, "D4":dbl, "D5":dbl, "D6":dbl, "R1":dbl, "R2":dbl, "R3":dbl, "SG14":dbl, "SG16-3":dbl, dbl, "SG18-3 ":dbl}}[]
  T3 = typedef "ControlCAN.lvlib/DevType.ctl" = u32
  T4 = typedef "ControlCAN.lvlib/CAN Channel.ctl" = u32
  T5 = typedef "ControlCAN.lvlib/VCI_INIT_CONFIG.ctl" = cluster{"AccCode":u32, "AccMask":u32, "InitFlag":T6, "Fliter":T7, "Timing0":u8, "Timing1":u8, "Mode":T8}
  T6 = typedef "ControlCAN.lvlib/InitFlag.ctl" = u32
  T7 = typedef "ControlCAN.lvlib/Fliter.ctl" = u8
  T8 = typedef "ControlCAN.lvlib/Mode.ctl" = u8
  T9 = cluster{"DevType":T3, "DevIndex":u32, "CanIndex":T4, "VCI_INIT_CONFIG":T5}
  T10 = enum16{"D1", "D2", "D3", "D4", "D5", "D6", "R1", "R2", "R3"}
  T11 = cluster{"CH1":bool, "CH2":bool, "CH3":bool, "CH4":bool, "CH5":bool, "CH6":bool, "CH7":bool, "CH8":bool, "CH9":bool, "CH10":bool, "CH11":bool, "CH12":bool, "CH13":bool, "CH14":bool, "CH15":bool, "CH16":bool}
  T12 = typedef "ControlCAN.lvlib/VCI_CAN_OBJ.ctl" = cluster{"ID":u32, "TimeStamp":u32, "TimeFlag":u8, "SendType":u8, "RemoteFlag":u8, "ExternFlag":u8, "DataLen":u8, "Data":u8[], "Reserved":u8[]}
  T13 = cluster{"Type":enum16{"接收", "发送"}, "Channel":T4, "Time":timestamp, "VCI_CAN_OBJ":T12}[]
  T14 = typedef "LVRectTypeDef.ctl" = cluster{"Left":i16, "Top":i16, "Right":i16, "Bottom":i16}
  T15 = cluster{"position (excel)":cluster{"row":i32, "column":i32}, "name (excel)":string, "bookmark (word)":string}
  T16 = enum16{"Standard Report", "HTML", "Word", "Excel"}
  T17 = enum32{"Invalid", "Standard", "Closed", "Hidden", "Minimized", "Maximized"}
  T18 = cluster{"D1":dbl, "D2":dbl, "D3":dbl, "D4":dbl, "D5":dbl, "D6":dbl, "R1":dbl, "R2":dbl, "R3":dbl, "SG14":dbl, "SG16-3":dbl, dbl, "SG18-3 ":dbl}
  T19 = enum32{"invalid app kind", "Development System", "Run Time System", "Student Edition", "Embedded LabVIEW", "Evaluation", "Custom"}
  T20 = cluster{"Type":enum16{"接收", "发送"}, "Channel":T4, "Time":timestamp, "VCI_CAN_OBJ":T12}
  T21 = typedef "ControlCAN.lvlib/Return Val.ctl" = i32
  T22 = cluster{"[0]":bool, "[1]":bool, "[2]":bool, "[3]":bool, "[4]":bool, "[5]":bool, "[6]":bool, "[7]":bool, "[8]":bool, "[9]":bool, "[10]":bool, "[11]":bool, "[12]":bool, "[13]":bool, "[14]":bool, "[15]":bool}
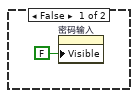
[diagram p4: hidden frame]
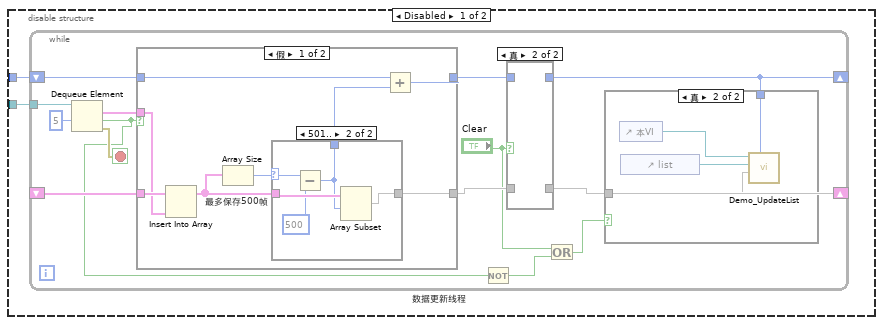
[diagram p8: hidden frame]
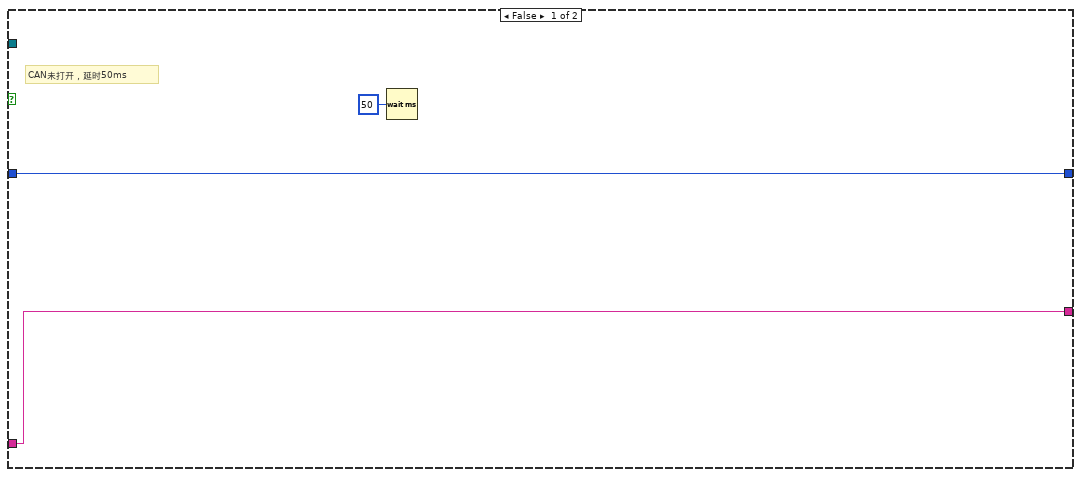
[diagram p13: hidden frame]
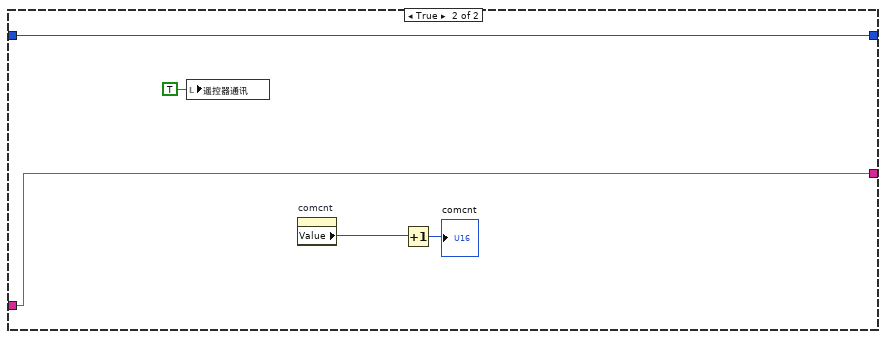
[diagram p16: hidden frame]
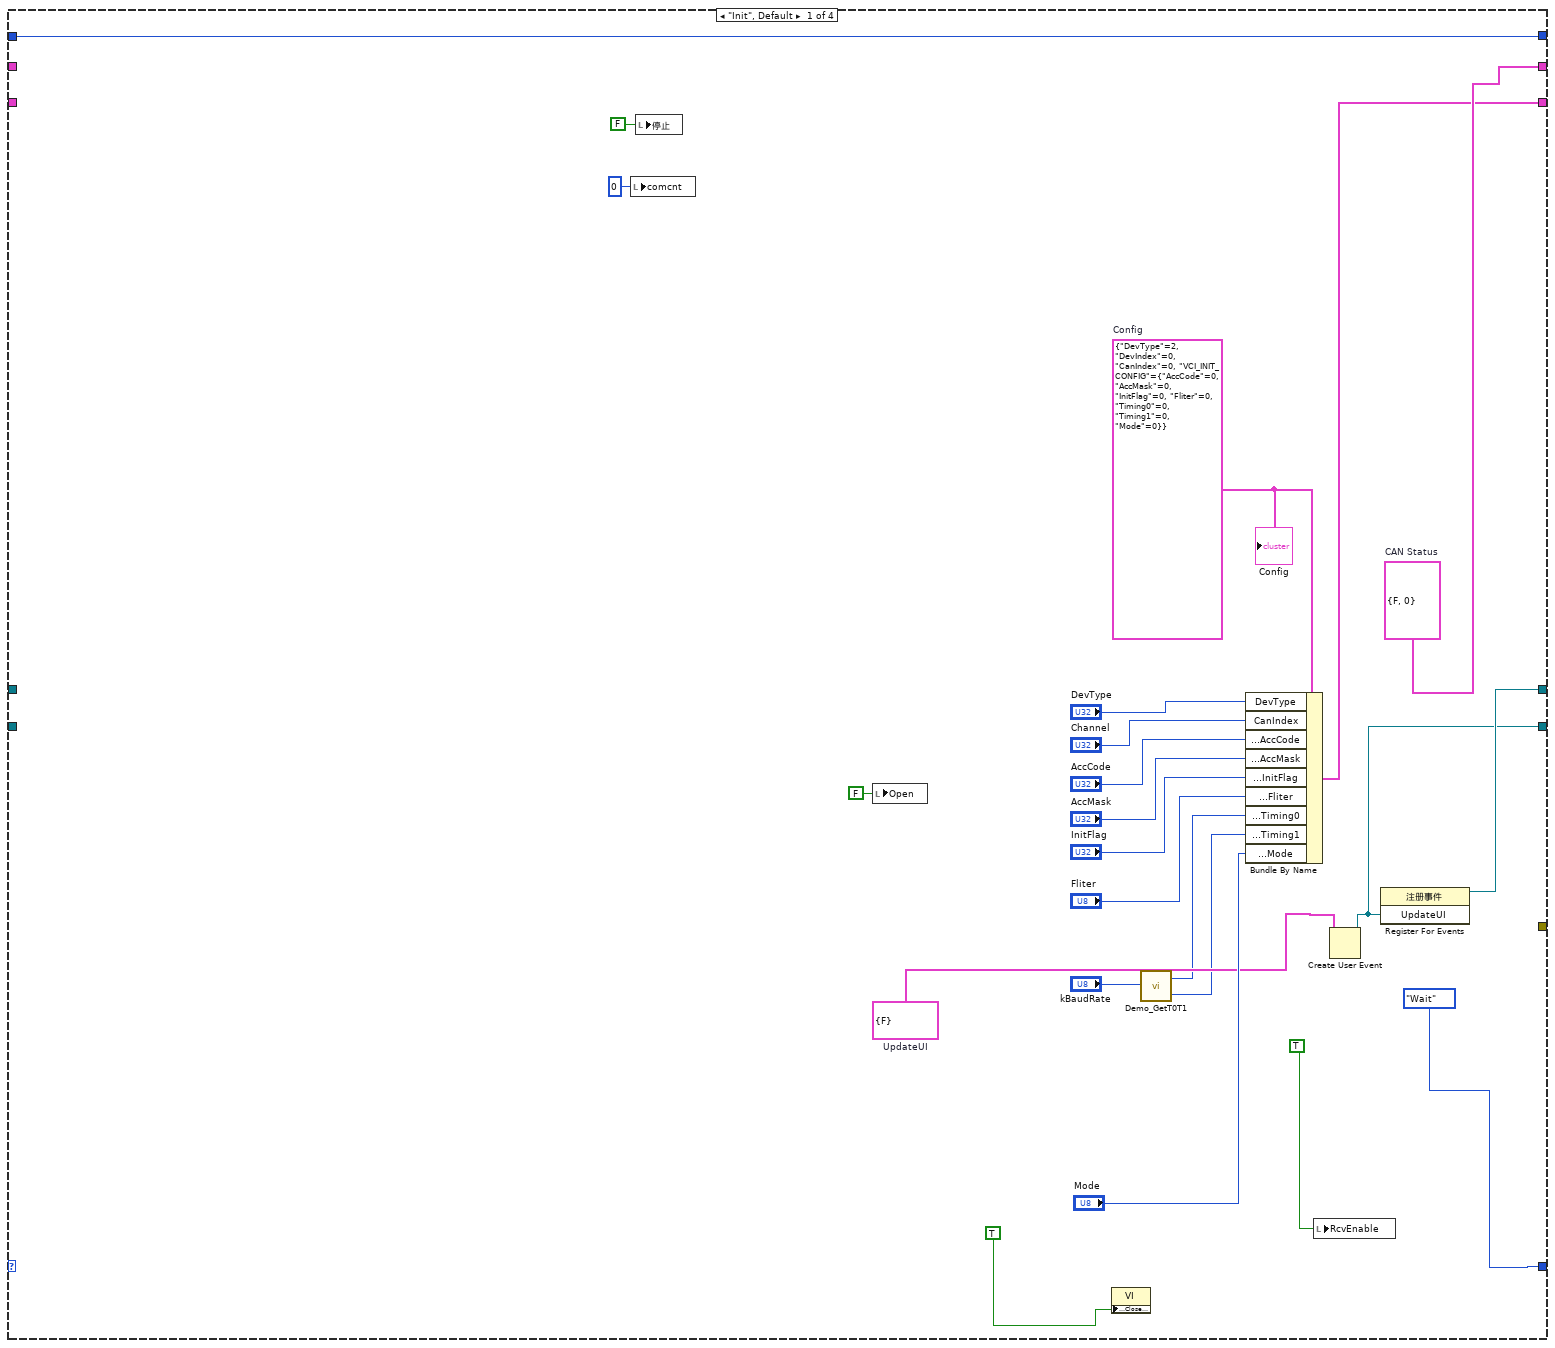
[diagram p17: hidden frame]
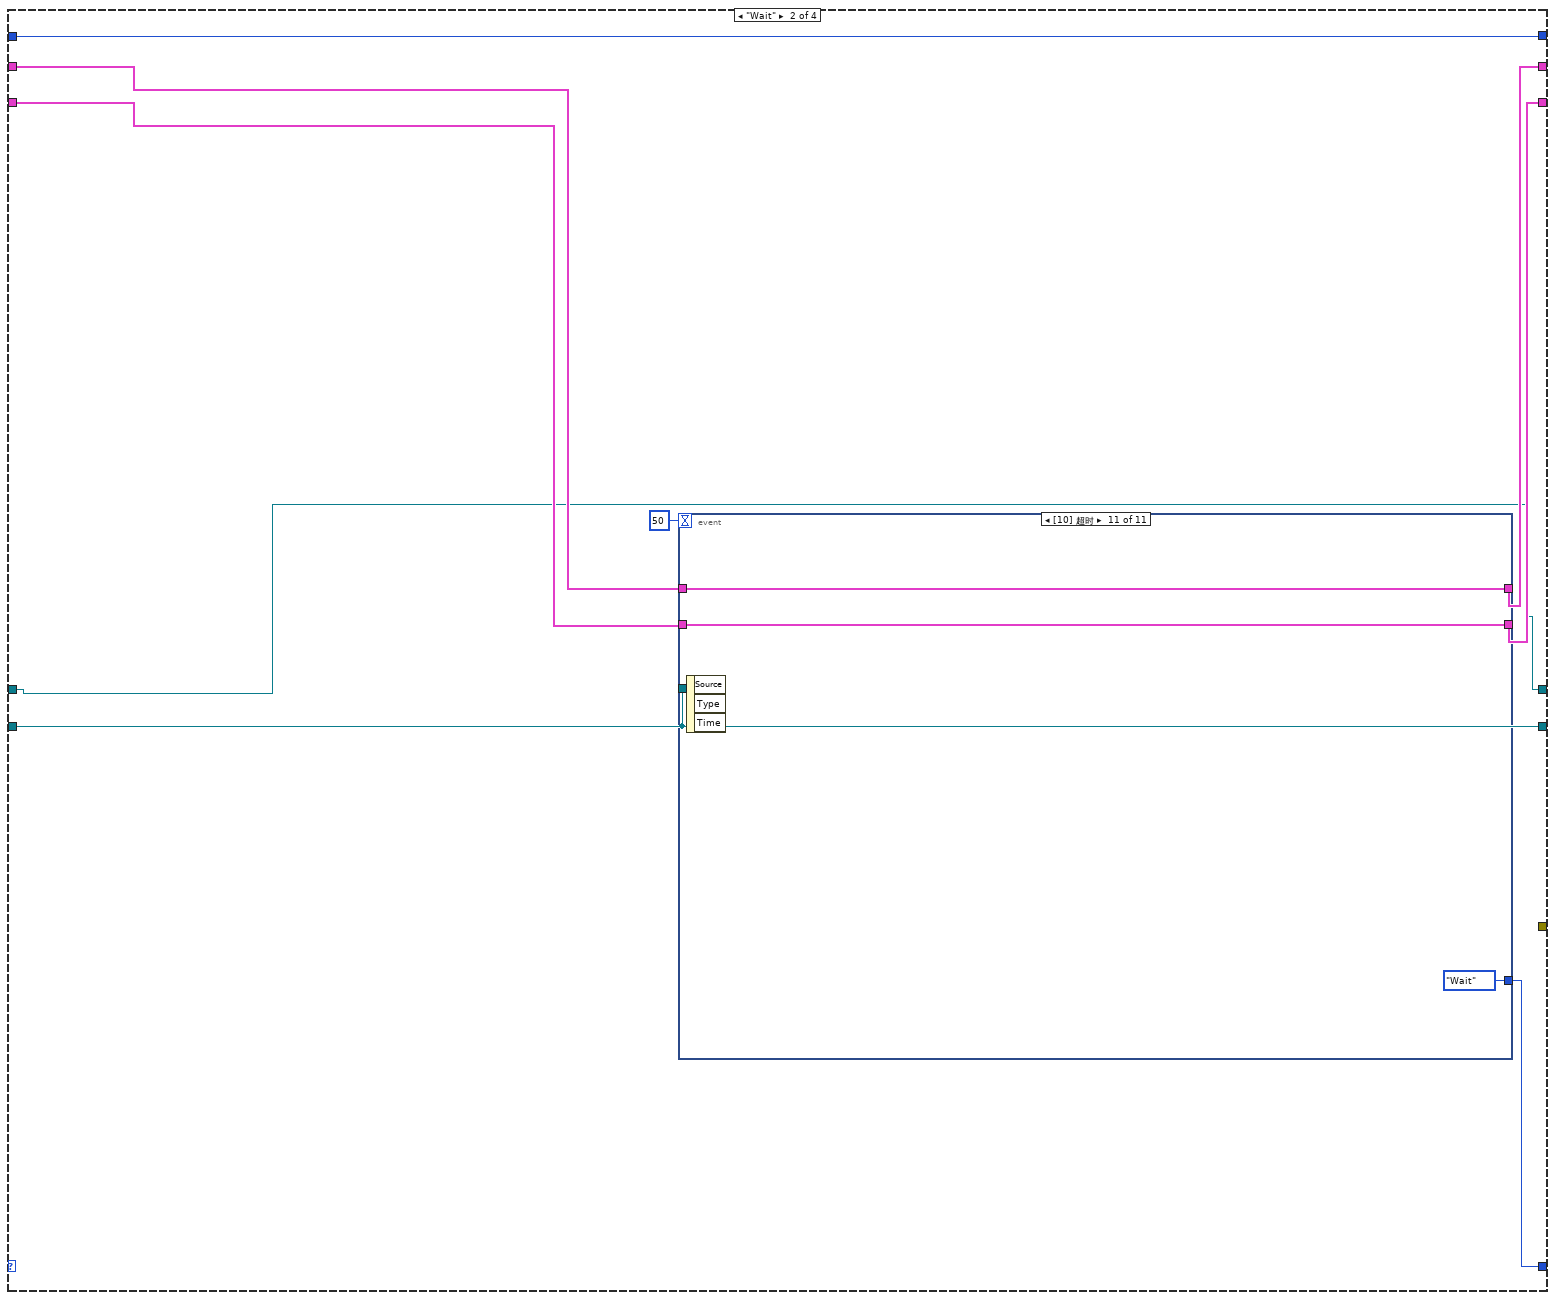
[diagram p18: hidden frame]
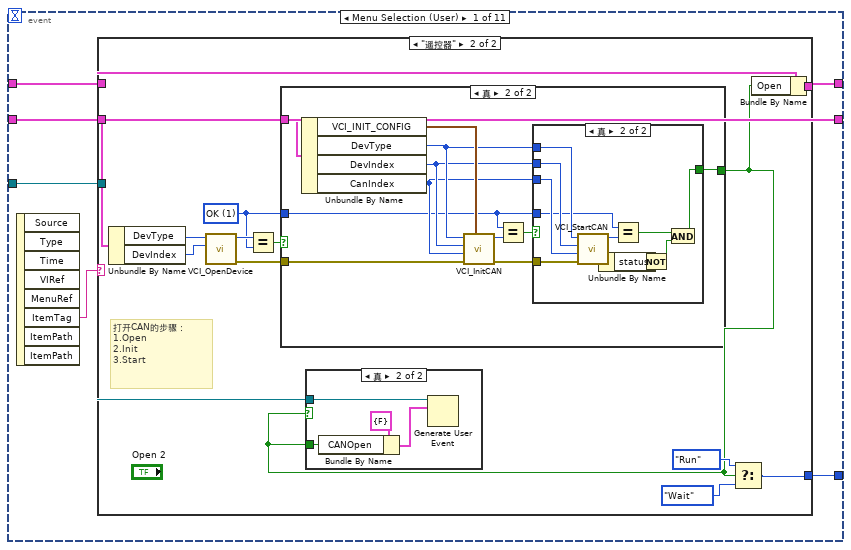
[diagram p19: hidden frame]
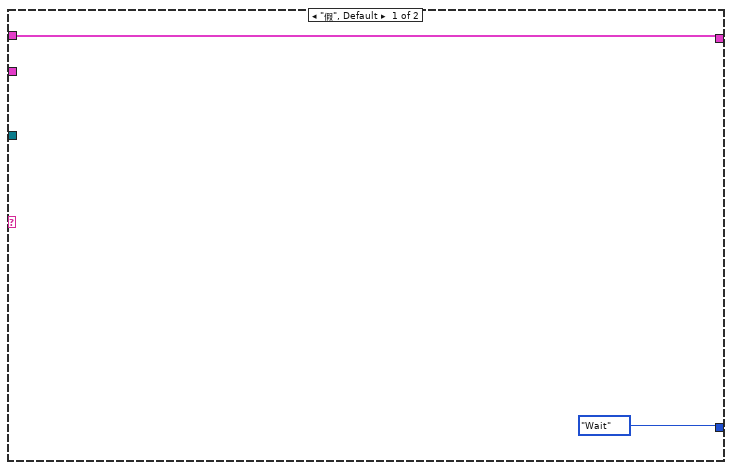
[diagram p20: hidden frame]
diagram:
  # "test1 commit"
  # "今天改了CAN"
  # "实验开始前平均速度要清零"
  n1 = disable-structure shown="启用" {
    disable-tunnel: [w29 _] -> w26
    frame Disabled {
      n2 = Obtain Queue(name (unnamed)="数据显示队列" ("名称（未命名）"), element data type=T13 []) -> (queue out=w29:refnum<queue>)  [unwired: 3 in, 2 out]
    }
    frame Enabled {
    }
  }
  n3 = disable-structure shown="禁用" {
    frame Disabled {
      n4 = property on="加载电机左下启动" class="Bool (严格)"("Val(Sgnl)"=FALSE ("值(信号)")) -> ()  [unwired: 2 in, 2 out]
      n5 = property on="驱动电机下启动" class="Bool (严格)"("Val(Sgnl)"=FALSE ("值(信号)")) -> ()  [unwired: 2 in, 2 out]
      n6 = property on="加载电机左上启动" class="Bool (严格)"("Val(Sgnl)"=FALSE ("值(信号)")) -> ()  [unwired: 2 in, 2 out]
      n7 = property on="加载电机右上启动" class="Bool (严格)"("Val(Sgnl)"=FALSE ("值(信号)")) -> ()  [unwired: 2 in, 2 out]
      n8 = property on="加载电机右下启动" class="Bool (严格)"("Val(Sgnl)"=FALSE ("值(信号)")) -> ()  [unwired: 2 in, 2 out]
      n9 = property on="驱动电机上启动" class="Bool (严格)"("Val(Sgnl)"=FALSE ("值(信号)")) -> ()  [unwired: 2 in, 2 out]
    }
    frame Enabled {
    }
  }
  n10 = flat-sequence {
    tunnel: [w45] -> w23
    tunnel: [w42] -> w22
    tunnel: [w49] -> w25
    tunnel: [w48] -> w24
    tunnel: w23 -> [w47]
    tunnel: w22 -> [w46]
    frame #0 {
      w37 = u16 0 items=["无", "奇", "偶"] ("parity (Even)")
      w44 = TRUE
      n11 = call-poly <vilib>:"Create Master Instance.vi"("serial type"=enum16{"RTU", "ASCII"}."RTU", "parity (Even)"=w37, "unit ID"=u8 1, "baud rate (9600)"=u32 9600, "VISA resource name"=refnum<visa-resource-name> "COM1") -> ("error out"=w42:errorcluster, "serial master instance"=w45:refnum<class "Modbus Master.lvclass">)  [unwired: 5 in]
      n12 = local write "停止"(FALSE ("停止")) -> ()
      n13 = Not(x=w42) -> (.not. x?=→"变频串口":bool)
      "变频1" <- w44
      "变频2" <- w44
      "变频3" <- w44
      "变频4" <- w44
      "变频5" <- w44
      "变频6" <- w44
    }
    frame #1 {
      n14 = while {
        shift-right: [w57] -> _
        shift-left: _ -> [w58]
        tunnel: [w55] -> w49
        shift-right: [w54] -> w48
        shift-left: w47 -> [w60]
        tunnel: w46 -> [w53]
        i -> [w52]
        stop <- w59 stop-if-true
        n15 = Tick Count (ms)() -> (millisecond timer value=w57:u32)
        n16 = Greater?(x=w52, y=2) -> (0:w50:bool)
        n17 = Subtract(x=w57, y=w58) -> (x-y=→"轮询耗时":u32)
        n18 = for {
          N: 6 -> [_]
          tunnel: w60 -> [w66]
          tunnel: [w65] -> w54
          shift-right: [w63] -> w55
          shift-left: w53 -> [w64]
          i -> [w68]
          n19 = Increment(x=w68) -> (x+1=w67:i32)
          n20 = case shown="4" w67 {
            tunnel: w66 -> [w145 w221 w326 w434 w547 w683]
            tunnel: [w111 w219 w324 w429 w548 w681] -> w65
            tunnel: w64 -> [w110 w220 w325 w433 w546 w682]
            tunnel: [w106 w214 w318 w428 w541 w676] -> w63
            frame 1, Default {
              w102 = 200 ("read operation timeout (ms)")
              n21 = local read "变频1"() -> (w140:bool)
              n22 = call <vilib>:"Set Unit ID.vi"("error in (no error)"=w110, "unit ID"=u8 1, "Modbus master in"=w145) -> ("error out"=w109:errorcluster, "Modbus master out"=w143:refnum<class "Modbus Master.lvclass">)  [unwired: 7 in]
              n23 = case shown="真" w140 {
                tunnel: w143 -> [w168 w173]
                tunnel: [w167 w172] -> w142
                tunnel: [w168 w171] -> w141
                tunnel: w109 -> [w167 _]
                frame False {
                }
                frame True {
                  n24 = for {
                    N: 2 -> [_]
                    tunnel: [w175] -> w172
                    shift-right: [w174] -> w171
                    shift-left: w173 -> [w178]
                    # "变频器初始化"
                    n25 = call-dynamic "Write Single Holding Register.vi"("holding register value"=u16 1142, "address"=u16 0, "Modbus master in"=w178) -> ("error out"=w175:errorcluster, "Modbus master out"=w174:refnum<class "Modbus Master.lvclass">)  [unwired: 7 in]
                  }
                  n26 = local write "变频1"(FALSE) -> ()
                }
              }
              n27 = flat-sequence {
                tunnel: w142 -> [w180]
                tunnel: [w180] -> w138
                tunnel: w141 -> [w179]
                tunnel: [w179] -> w139
                frame #0 {
                  n28 = Wait (ms)(milliseconds to wait=u32 10 ("等待时间（毫秒）")) -> ()  [unwired: 1 out]
                }
              }
              n29 = case shown="假" "加载电机左上启动" {
                tunnel: w139 -> [w156 w162]
                tunnel: [w155 w159] -> w87
                tunnel: [w151 w158] -> w89
                tunnel: w138 -> [w152 w157]
                frame False {
                  n30 = call-dynamic "Write Single Holding Register.vi"("error in (no error)"=w152, "holding register value"=u16 1143, "address"=u16 0, "Modbus master in"=w156) -> ("error out"=w151:errorcluster, "Modbus master out"=w155:refnum<class "Modbus Master.lvclass">)  [unwired: 6 in]
                }
                frame True {
                  n31 = call-dynamic "Write Single Holding Register.vi"("error in (no error)"=w157, "holding register value"=u16 1151, "address"=u16 0, "Modbus master in"=w162) -> ("error out"=w158:errorcluster, "Modbus master out"=w159:refnum<class "Modbus Master.lvclass">)  [unwired: 6 in]
                }
              }
              n32 = case shown="假" "加载电机左上正反转" {
                tunnel: [w163 w166] -> w135
                frame False {
                  n33 = local read "加载电机左上转矩给定"() -> (w163:i16)
                }
                frame True {
                  n34 = Multiply(x="加载电机左上转矩给定", y=i8 -1) -> (x*y=w166:i16)
                }
              }
              n35 = flat-sequence {
                tunnel: w89 -> [w147]
                tunnel: [w147] -> w88
                tunnel: w87 -> [w146]
                tunnel: [w146] -> _
                tunnel: [w146] -> w86
                frame #0 {
                  n36 = Wait (ms)(milliseconds to wait=u32 10 ("等待时间（毫秒）")) -> ()  [unwired: 1 out]
                }
              }
              n37 = call-dynamic "Write Single Holding Register.vi"("error in (no error)"=w88, "holding register value"=w135, "address"=u16 1, "Modbus master in"=w86) -> ("error out"=w104:errorcluster, "Modbus master out"=w105:refnum<class "Modbus Master.lvclass">)  [unwired: 6 in]
              n38 = local read "加载左上转矩监控"() -> (w69:i16)
              n39 = call-dynamic "Read Holding Registers.vi"("error in (no error)"=w104, "number of holding registers"=u16 2, "starting address"=u16 109, "Modbus master in"=w105) -> ("error out"=w108:errorcluster, "register values"=w123:u16[], "Modbus master out"=w116:refnum<class "Modbus Master.lvclass">)  [unwired: 5 in]
              n40 = Index Array(array=w123) -> (element #1=→"加载左上转矩监控":u16, element #2=w121:u16)  [unwired: 2 in]
              n41 = Divide(x=w121, y=u16 10) -> (x/y=→"加载电机左上母线电压":dbl)
              n42 = call-dynamic "Read Holding Registers.vi"("error in (no error)"=w108, "number of holding registers"=u16 1, "starting address"=u16 106, "Modbus master in"=w116) -> ("error out"=w103:errorcluster, "register values"=w115:u16[], "Modbus master out"=w90:refnum<class "Modbus Master.lvclass">)  [unwired: 5 in]
              n43 = Index Array(array=w115) -> (element #1=w114:u16)  [unwired: 2 in, 1 out]
              n44 = Multiply(x=w114, y=0.3) -> (x*y=→"加载电机左上母线电流":dbl)
              n45 = Divide(x=w69, y=u16 10000) -> (x/y=w72:dbl)
              n46 = Multiply(x=w72, y=800.0) -> (x*y=→"加载扭矩N.M(单个）":dbl)
              n47 = call-dynamic "Read Holding Registers.vi"("error in (no error)"=w103, "number of holding registers"=u16 2, "starting address"=u16 20200 ("address"), "Modbus master in"=w90) -> ("error out"=w85:errorcluster, "register values"=w132:u16[], "Modbus master out"=w98:refnum<class "Modbus Master.lvclass">)  [unwired: 5 in]
              n48 = Index Array(array=w132) -> (element #1=w129:u16, element #2=w131:u16)  [unwired: 2 in]
              n49 = Multiply(x=w131, y=u32 65536) -> (x*y=w128:u32)
              n50 = Add(x=w129, y=w128) -> (x+y=w127:u32)
              n51 = To Long Integer(number=w127) -> (32bit integer=w126:i32)
              n52 = Divide(x=w126, y=100) -> (x/y=→"加载左上转速监控" →"后左":dbl)
              n53 = call-dynamic "Read Holding Registers.vi"("error in (no error)"=w85, "number of holding registers"=u16 2, "starting address"=u16 420, "Modbus master in"=w98) -> ("error out"=w82:errorcluster, "register values"=w95:u16[], "Modbus master out"=w84:refnum<class "Modbus Master.lvclass">)  [unwired: 5 in]
              n54 = Index Array(array=w95) -> (element #1=w94:u16, element #2=w93:u16)  [unwired: 2 in]
              n55 = call-dynamic "Read Holding Registers.vi"("error in (no error)"=w82, "number of holding registers"=u16 1, "starting address"=u16 615, "Modbus master in"=w84) -> ("error out"=w81:errorcluster, "register values"=w79:u16[], "Modbus master out"=w83:refnum<class "Modbus Master.lvclass">)  [unwired: 5 in]
              n56 = Add(x=w94, y=w93) -> (x+y=w92:u16)
              n57 = Greater Than 0?(x=w92) -> (x > 0?=w91:bool)
              n58 = case shown="真" w91 {
                frame False {
                  n59 = local write "变频故障1"(FALSE ("变频故障1")) -> ()
                }
                frame True {
                  "变频故障1" <- TRUE ("变频故障1")
                }
              }
              n60 = call <vilib>:"Set Timeouts.vi"("error in (no error)"=w81, "write operation timeout (ms)"=w102, "read operation timeout (ms)"=w102, "Modbus master in"=w83) -> ("error out"=w106:errorcluster, "Modbus master out"=w111:refnum<class "Modbus Master.lvclass">)  [unwired: 6 in]
              n61 = Index Array(array=w79) -> (element=w78:u16)  [unwired: 1 in]
              n62 = Number To Boolean Array(number=w78) -> (Boolean array=w76:bool[])
              "后左" <- w76
              n63 = Index Array(array=w76, index=5 ("索引")) -> (element=→"后左":bool)
              n64 = Wait (ms)(milliseconds to wait=u32 50 ("等待时间（毫秒）")) -> ()  [unwired: 1 out]
            }
            frame 2 {
              w210 = 200 ("read operation timeout (ms)")
              n65 = local read "变频2"() -> (w249:bool)
              n66 = call <vilib>:"Set Unit ID.vi"("error in (no error)"=w220, "unit ID"=u8 2, "Modbus master in"=w221) -> ("error out"=w224:errorcluster, "Modbus master out"=w252:refnum<class "Modbus Master.lvclass">)  [unwired: 7 in]
              n67 = case shown="真" w249 {
                tunnel: w252 -> [w276 w282]
                tunnel: [w275 w279] -> w251
                tunnel: [w276 w278] -> w250
                tunnel: w224 -> [w275 _]
                frame False {
                }
                frame True {
                  # "变频器初始化"
                  n68 = call-dynamic "Write Single Holding Register.vi"("holding register value"=u16 1142, "address"=u16 0, "Modbus master in"=w282) -> ("error out"=w279:errorcluster, "Modbus master out"=w278:refnum<class "Modbus Master.lvclass">)  [unwired: 7 in]
                  n69 = local write "变频2"(FALSE) -> ()
                }
              }
              n70 = flat-sequence {
                tunnel: w251 -> [w284]
                tunnel: [w284] -> w247
                tunnel: w250 -> [w283]
                tunnel: [w283] -> w248
                frame #0 {
                  n71 = Wait (ms)(milliseconds to wait=u32 10 ("等待时间（毫秒）")) -> ()  [unwired: 1 out]
                }
              }
              n72 = case shown="假" "加载电机左下启动" {
                tunnel: w248 -> [w264 w270]
                tunnel: [w263 w267] -> w197
                tunnel: [w259 w266] -> w195
                tunnel: w247 -> [w260 w265]
                frame False {
                  n73 = call-dynamic "Write Single Holding Register.vi"("error in (no error)"=w260, "holding register value"=u16 1143, "address"=u16 0, "Modbus master in"=w264) -> ("error out"=w259:errorcluster, "Modbus master out"=w263:refnum<class "Modbus Master.lvclass">)  [unwired: 6 in]
                }
                frame True {
                  n74 = call-dynamic "Write Single Holding Register.vi"("error in (no error)"=w265, "holding register value"=u16 1151, "address"=u16 0, "Modbus master in"=w270) -> ("error out"=w266:errorcluster, "Modbus master out"=w267:refnum<class "Modbus Master.lvclass">)  [unwired: 6 in]
                }
              }
              n75 = flat-sequence {
                tunnel: w195 -> [w255]
                tunnel: [w255] -> w194
                tunnel: w197 -> [w254]
                tunnel: [w254] -> w196
                frame #0 {
                  n76 = Wait (ms)(milliseconds to wait=u32 10 ("等待时间（毫秒）")) -> ()  [unwired: 1 out]
                }
              }
              n77 = case shown="真" "加载电机左下正反转" {
                tunnel: [w271 w274] -> w245
                frame False {
                  n78 = local read "加载电机左下转矩给定"() -> (w271:i16)
                }
                frame True {
                  n79 = Multiply(x="加载电机左下转矩给定", y=i8 -1) -> (x*y=w274:i16)
                }
              }
              n80 = call-dynamic "Write Single Holding Register.vi"("error in (no error)"=w194, "holding register value"=w245, "address"=u16 1, "Modbus master in"=w196) -> ("error out"=w212:errorcluster, "Modbus master out"=w213:refnum<class "Modbus Master.lvclass">)  [unwired: 6 in]
              n81 = call-dynamic "Read Holding Registers.vi"("error in (no error)"=w212, "number of holding registers"=u16 2, "starting address"=u16 109, "Modbus master in"=w213) -> ("error out"=w223:errorcluster, "register values"=w233:u16[], "Modbus master out"=w228:refnum<class "Modbus Master.lvclass">)  [unwired: 5 in]
              n82 = Index Array(array=w233) -> (element #1=→"加载左下转矩监控":u16, element #2=w232:u16)  [unwired: 2 in]
              n83 = Divide(x=w232, y=u16 10) -> (x/y=→"加载电机左下母线电压":dbl)
              n84 = call-dynamic "Read Holding Registers.vi"("error in (no error)"=w223, "number of holding registers"=u16 1, "starting address"=u16 106, "Modbus master in"=w228) -> ("error out"=w211:errorcluster, "register values"=w227:u16[], "Modbus master out"=w198:refnum<class "Modbus Master.lvclass">)  [unwired: 5 in]
              n85 = Index Array(array=w227) -> (element #1=w226:u16)  [unwired: 2 in, 1 out]
              n86 = Multiply(x=w226, y=0.3) -> (x*y=→"加载电机左下母线电流":dbl)
              n87 = call-dynamic "Read Holding Registers.vi"("error in (no error)"=w211, "number of holding registers"=u16 2, "starting address"=u16 20200 ("address"), "Modbus master in"=w198) -> ("error out"=w193:errorcluster, "register values"=w242:u16[], "Modbus master out"=w199:refnum<class "Modbus Master.lvclass">)  [unwired: 5 in]
              n88 = Index Array(array=w242) -> (element #1=w239:u16, element #2=w241:u16)  [unwired: 2 in]
              n89 = Multiply(x=w241, y=u32 65536) -> (x*y=w238:u32)
              n90 = Add(x=w239, y=w238) -> (x+y=w237:u32)
              n91 = To Long Integer(number=w237) -> (32bit integer=w236:i32)
              n92 = Divide(x=w236, y=100) -> (x/y=→"加载左下转速监控" →"后右":dbl)
              n93 = call-dynamic "Read Holding Registers.vi"("error in (no error)"=w193, "number of holding registers"=u16 2, "starting address"=u16 420, "Modbus master in"=w199) -> ("error out"=w185:errorcluster, "register values"=w203:u16[], "Modbus master out"=w192:refnum<class "Modbus Master.lvclass">)  [unwired: 5 in]
              n94 = Index Array(array=w203) -> (element #1=w202:u16, element #2=w201:u16)  [unwired: 2 in]
              n95 = Add(x=w202, y=w201) -> (x+y=w206:u16)
              n96 = Greater Than 0?(x=w206) -> (x > 0?=w200:bool)
              n97 = case shown="真" w200 {
                frame False {
                  n98 = local write "变频故障2"(FALSE ("变频故障2")) -> ()
                }
                frame True {
                  "变频故障2" <- TRUE ("变频故障2")
                }
              }
              n99 = call-dynamic "Read Holding Registers.vi"("error in (no error)"=w185, "number of holding registers"=u16 1, "starting address"=u16 615, "Modbus master in"=w192) -> ("error out"=w188:errorcluster, "register values"=w187:u16[], "Modbus master out"=w191:refnum<class "Modbus Master.lvclass">)  [unwired: 5 in]
              n100 = Index Array(array=w187) -> (element=w186:u16)  [unwired: 1 in]
              n101 = call <vilib>:"Set Timeouts.vi"("error in (no error)"=w188, "write operation timeout (ms)"=w210, "read operation timeout (ms)"=w210, "Modbus master in"=w191) -> ("error out"=w214:errorcluster, "Modbus master out"=w219:refnum<class "Modbus Master.lvclass">)  [unwired: 6 in]
              n102 = Number To Boolean Array(number=w186) -> (Boolean array=w184:bool[])
              "后右" <- w184
              n103 = Index Array(array=w184, index=5 ("索引")) -> (element=→"后右":bool)
              n104 = Wait (ms)(milliseconds to wait=u32 50 ("等待时间（毫秒）")) -> ()  [unwired: 1 out]
            }
            frame 3 {
              w314 = 200 ("read operation timeout (ms)")
              n105 = local read "变频3"() -> (w323:bool)
              n106 = call <vilib>:"Set Unit ID.vi"("error in (no error)"=w325, "unit ID"=u8 3, "Modbus master in"=w326) -> ("error out"=w329:errorcluster, "Modbus master out"=w356:refnum<class "Modbus Master.lvclass">)  [unwired: 7 in]
              n107 = case shown="真" w323 {
                tunnel: w356 -> [w380 w385]
                tunnel: [w379 w384] -> w355
                tunnel: [w380 w383] -> w354
                tunnel: w329 -> [w379 _]
                frame False {
                }
                frame True {
                  n108 = for {
                    N: 2 -> [_]
                    tunnel: [w387] -> w384
                    shift-right: [w386] -> w383
                    shift-left: w385 -> [w390]
                    # "变频器初始化"
                    n109 = call-dynamic "Write Single Holding Register.vi"("holding register value"=u16 1142, "address"=u16 0, "Modbus master in"=w390) -> ("error out"=w387:errorcluster, "Modbus master out"=w386:refnum<class "Modbus Master.lvclass">)  [unwired: 7 in]
                  }
                  n110 = local write "变频3"(FALSE) -> ()
                }
              }
              n111 = flat-sequence {
                tunnel: w355 -> [w392]
                tunnel: [w392] -> w352
                tunnel: w354 -> [w391]
                tunnel: [w391] -> w353
                frame #0 {
                  n112 = Wait (ms)(milliseconds to wait=u32 10 ("等待时间（毫秒）")) -> ()  [unwired: 1 out]
                }
              }
              n113 = case shown="假" "加载电机右上启动" {
                tunnel: w353 -> [w368 w374]
                tunnel: [w367 w371] -> w302
                tunnel: [w363 w370] -> w300
                tunnel: w352 -> [w364 w369]
                frame False {
                  n114 = call-dynamic "Write Single Holding Register.vi"("error in (no error)"=w364, "holding register value"=u16 1143, "address"=u16 0, "Modbus master in"=w368) -> ("error out"=w363:errorcluster, "Modbus master out"=w367:refnum<class "Modbus Master.lvclass">)  [unwired: 6 in]
                }
                frame True {
                  n115 = call-dynamic "Write Single Holding Register.vi"("error in (no error)"=w369, "holding register value"=u16 1151, "address"=u16 0, "Modbus master in"=w374) -> ("error out"=w370:errorcluster, "Modbus master out"=w371:refnum<class "Modbus Master.lvclass">)  [unwired: 6 in]
                }
              }
              n116 = flat-sequence {
                tunnel: w300 -> [w359]
                tunnel: [w359] -> w299
                tunnel: w302 -> [w358]
                tunnel: [w358] -> w301
                frame #0 {
                  n117 = Wait (ms)(milliseconds to wait=u32 10 ("等待时间（毫秒）")) -> ()  [unwired: 1 out]
                }
              }
              n118 = case shown="真" "加载电机右上正反转" {
                tunnel: [w375 w378] -> w350
                frame False {
                  n119 = local read "加载电机右上转矩给定"() -> (w375:i16)
                }
                frame True {
                  n120 = Multiply(x="加载电机右上转矩给定", y=i8 -1) -> (x*y=w378:i16)
                }
              }
              n121 = call-dynamic "Write Single Holding Register.vi"("error in (no error)"=w299, "holding register value"=w350, "address"=u16 1, "Modbus master in"=w301) -> ("error out"=w316:errorcluster, "Modbus master out"=w317:refnum<class "Modbus Master.lvclass">)  [unwired: 6 in]
              n122 = call-dynamic "Read Holding Registers.vi"("error in (no error)"=w316, "number of holding registers"=u16 2, "starting address"=u16 109, "Modbus master in"=w317) -> ("error out"=w328:errorcluster, "register values"=w338:u16[], "Modbus master out"=w333:refnum<class "Modbus Master.lvclass">)  [unwired: 5 in]
              n123 = Index Array(array=w338) -> (element #1=→"加载转矩右上监控":u16, element #2=w337:u16)  [unwired: 2 in]
              n124 = Divide(x=w337, y=u16 10) -> (x/y=→"加载电机右上母线电压":dbl)
              n125 = call-dynamic "Read Holding Registers.vi"("error in (no error)"=w328, "number of holding registers"=u16 1, "starting address"=u16 106, "Modbus master in"=w333) -> ("error out"=w315:errorcluster, "register values"=w332:u16[], "Modbus master out"=w298:refnum<class "Modbus Master.lvclass">)  [unwired: 5 in]
              n126 = Index Array(array=w332) -> (element #1=w331:u16)  [unwired: 2 in, 1 out]
              n127 = Multiply(x=w331, y=0.3) -> (x*y=→"加载电机右上母线电流":dbl)
              n128 = call-dynamic "Read Holding Registers.vi"("error in (no error)"=w315, "number of holding registers"=u16 2, "starting address"=u16 20200 ("address"), "Modbus master in"=w298) -> ("error out"=w297:errorcluster, "register values"=w347:u16[], "Modbus master out"=w303:refnum<class "Modbus Master.lvclass">)  [unwired: 5 in]
              n129 = Index Array(array=w347) -> (element #1=w344:u16, element #2=w346:u16)  [unwired: 2 in]
              n130 = Multiply(x=w346, y=u32 65536) -> (x*y=w343:u32)
              n131 = Add(x=w344, y=w343) -> (x+y=w342:u32)
              n132 = To Long Integer(number=w342) -> (32bit integer=w341:i32)
              n133 = Divide(x=w341, y=100) -> (x/y=→"加载右上转速监控" →"中左":dbl)
              n134 = call-dynamic "Read Holding Registers.vi"("error in (no error)"=w297, "number of holding registers"=u16 2, "starting address"=u16 420, "Modbus master in"=w303) -> ("error out"=w294:errorcluster, "register values"=w307:u16[], "Modbus master out"=w296:refnum<class "Modbus Master.lvclass">)  [unwired: 5 in]
              n135 = Index Array(array=w307) -> (element #1=w306:u16, element #2=w305:u16)  [unwired: 2 in]
              n136 = call-dynamic "Read Holding Registers.vi"("error in (no error)"=w294, "number of holding registers"=u16 1, "starting address"=u16 615, "Modbus master in"=w296) -> ("error out"=w293:errorcluster, "register values"=w290:u16[], "Modbus master out"=w295:refnum<class "Modbus Master.lvclass">)  [unwired: 5 in]
              n137 = Wait (ms)(milliseconds to wait=u32 50 ("等待时间（毫秒）")) -> ()  [unwired: 1 out]
              n138 = Add(x=w306, y=w305) -> (x+y=w310:u16)
              n139 = Greater Than 0?(x=w310) -> (x > 0?=w304:bool)
              n140 = case shown="真" w304 {
                frame False {
                  n141 = local write "变频故障 3"(FALSE ("变频故障 3")) -> ()
                }
                frame True {
                  "变频故障 3" <- TRUE ("变频故障 3")
                }
              }
              n142 = Index Array(array=w290) -> (element=w289:u16)  [unwired: 1 in]
              n143 = Number To Boolean Array(number=w289) -> (Boolean array=w288:bool[])
              "中左" <- w288
              n144 = Index Array(array=w288, index=5 ("索引")) -> (element=→"中左":bool)
              n145 = call <vilib>:"Set Timeouts.vi"("error in (no error)"=w293, "write operation timeout (ms)"=w314, "read operation timeout (ms)"=w314, "Modbus master in"=w295) -> ("error out"=w318:errorcluster, "Modbus master out"=w324:refnum<class "Modbus Master.lvclass">)  [unwired: 6 in]
            }
            frame 4 {
              w424 = 200 ("read operation timeout (ms)")
              n146 = call <vilib>:"Set Unit ID.vi"("error in (no error)"=w433, "unit ID"=u8 4, "Modbus master in"=w434) -> ("error out"=w438:errorcluster, "Modbus master out"=w464:refnum<class "Modbus Master.lvclass">)  [unwired: 7 in]
              n147 = local read "变频4"() -> (w435:bool)
              n148 = case shown="真" w435 {
                tunnel: w464 -> [w488 w494]
                tunnel: [w487 w493] -> w463
                tunnel: [w488 w492] -> w462
                tunnel: w438 -> [w487 w490]
                frame False {
                }
                frame True {
                  n149 = for {
                    N: 2 -> [_]
                    shift-right: [w496] -> w492
                    shift-left: w494 -> [w500]
                    shift-right: [w497] -> w493
                    shift-left: w490 -> [w495]
                    # "变频器初始化"
                    n150 = call-dynamic "Write Single Holding Register.vi"("error in (no error)"=w495, "holding register value"=u16 1142, "address"=u16 0, "Modbus master in"=w500) -> ("error out"=w497:errorcluster, "Modbus master out"=w496:refnum<class "Modbus Master.lvclass">)  [unwired: 6 in]
                  }
                  n151 = local write "变频4"(FALSE) -> ()
                }
              }
              n152 = flat-sequence {
                tunnel: w463 -> [w502]
                tunnel: [w502] -> w460
                tunnel: w462 -> [w501]
                tunnel: [w501] -> w461
                frame #0 {
                  n153 = Wait (ms)(milliseconds to wait=u32 10 ("等待时间（毫秒）")) -> ()  [unwired: 1 out]
                }
              }
              n154 = case shown="假" "加载电机右下启动" {
                tunnel: w461 -> [w476 w482]
                tunnel: [w475 w479] -> w410
                tunnel: [w471 w478] -> w408
                tunnel: w460 -> [w472 w477]
                frame False {
                  n155 = call-dynamic "Write Single Holding Register.vi"("error in (no error)"=w472, "holding register value"=u16 1143, "address"=u16 0, "Modbus master in"=w476) -> ("error out"=w471:errorcluster, "Modbus master out"=w475:refnum<class "Modbus Master.lvclass">)  [unwired: 6 in]
                }
                frame True {
                  n156 = call-dynamic "Write Single Holding Register.vi"("error in (no error)"=w477, "holding register value"=u16 1151, "address"=u16 0, "Modbus master in"=w482) -> ("error out"=w478:errorcluster, "Modbus master out"=w479:refnum<class "Modbus Master.lvclass">)  [unwired: 6 in]
                }
              }
              n157 = flat-sequence {
                tunnel: w408 -> [w467]
                tunnel: [w467] -> w407
                tunnel: w410 -> [w466]
                tunnel: [w466] -> w409
                frame #0 {
                  n158 = Wait (ms)(milliseconds to wait=u32 10 ("等待时间（毫秒）")) -> ()  [unwired: 1 out]
                }
              }
              n159 = case shown="假" "加载电机右下正反转" {
                tunnel: [w483 w486] -> w394
                frame False {
                  n160 = local read "加载电机右下转矩给定"() -> (w483:i16)
                }
                frame True {
                  n161 = Multiply(x="加载电机右下转矩给定", y=i8 -1) -> (x*y=w486:i16)
                }
              }
              n162 = call-dynamic "Write Single Holding Register.vi"("error in (no error)"=w407, "holding register value"=w394, "address"=u16 1, "Modbus master in"=w409) -> ("error out"=w427:errorcluster, "Modbus master out"=w426:refnum<class "Modbus Master.lvclass">)  [unwired: 6 in]
              n163 = call-dynamic "Read Holding Registers.vi"("error in (no error)"=w427, "number of holding registers"=u16 2, "starting address"=u16 109, "Modbus master in"=w426) -> ("error out"=w437:errorcluster, "register values"=w447:u16[], "Modbus master out"=w442:refnum<class "Modbus Master.lvclass">)  [unwired: 5 in]
              n164 = Index Array(array=w447) -> (element #1=→"加载右下转矩监控":u16, element #2=w446:u16)  [unwired: 2 in]
              n165 = Divide(x=w446, y=u16 10) -> (x/y=→"加载电机右下母线电压":dbl)
              n166 = call-dynamic "Read Holding Registers.vi"("error in (no error)"=w437, "number of holding registers"=u16 1, "starting address"=u16 106, "Modbus master in"=w442) -> ("error out"=w425:errorcluster, "register values"=w441:u16[], "Modbus master out"=w411:refnum<class "Modbus Master.lvclass">)  [unwired: 5 in]
              n167 = Index Array(array=w441) -> (element #1=w440:u16)  [unwired: 2 in, 1 out]
              n168 = Multiply(x=w440, y=0.3) -> (x*y=→"加载电机右下母线电流":dbl)
              n169 = call-dynamic "Read Holding Registers.vi"("error in (no error)"=w425, "number of holding registers"=u16 2, "starting address"=u16 20200 ("address"), "Modbus master in"=w411) -> ("error out"=w406:errorcluster, "register values"=w456:u16[], "Modbus master out"=w412:refnum<class "Modbus Master.lvclass">)  [unwired: 5 in]
              n170 = Index Array(array=w456) -> (element #1=w453:u16, element #2=w455:u16)  [unwired: 2 in]
              n171 = Multiply(x=w455, y=u32 65536) -> (x*y=w452:u32)
              n172 = Add(x=w453, y=w452) -> (x+y=w451:u32)
              n173 = To Long Integer(number=w451) -> (32bit integer=w450:i32)
              n174 = Divide(x=w450, y=100) -> (x/y=→"加载转速右下监控" →"中右":dbl)
              n175 = call-dynamic "Read Holding Registers.vi"("error in (no error)"=w406, "number of holding registers"=u16 2, "starting address"=u16 420, "Modbus master in"=w412) -> ("error out"=w403:errorcluster, "register values"=w416:u16[], "Modbus master out"=w405:refnum<class "Modbus Master.lvclass">)  [unwired: 5 in]
              n176 = Wait (ms)(milliseconds to wait=u32 50 ("等待时间（毫秒）")) -> ()  [unwired: 1 out]
              n177 = call-dynamic "Read Holding Registers.vi"("error in (no error)"=w403, "number of holding registers"=u16 1, "starting address"=u16 615, "Modbus master in"=w405) -> ("error out"=w402:errorcluster, "register values"=w399:u16[], "Modbus master out"=w404:refnum<class "Modbus Master.lvclass">)  [unwired: 5 in]
              n178 = Index Array(array=w416) -> (element #1=w415:u16, element #2=w414:u16)  [unwired: 2 in]
              n179 = Add(x=w415, y=w414) -> (x+y=w419:u16)
              n180 = Greater Than 0?(x=w419) -> (x > 0?=w413:bool)
              n181 = case shown="真" w413 {
                frame False {
                  n182 = local write "变频故障 4"(FALSE ("变频故障 4")) -> ()
                }
                frame True {
                  "变频故障 4" <- TRUE ("变频故障 4")
                }
              }
              n183 = call <vilib>:"Set Timeouts.vi"("error in (no error)"=w402, "write operation timeout (ms)"=w424, "read operation timeout (ms)"=w424, "Modbus master in"=w404) -> ("error out"=w428:errorcluster, "Modbus master out"=w429:refnum<class "Modbus Master.lvclass">)  [unwired: 6 in]
              n184 = Index Array(array=w399) -> (element=w398:u16)  [unwired: 1 in]
              n185 = Number To Boolean Array(number=w398) -> (Boolean array=w397:bool[])
              "中右" <- w397
              n186 = Index Array(array=w397, index=5 ("索引")) -> (element=→"中右":bool)
            }
            frame 5 {
              w537 = 200 ("read operation timeout (ms)")
              n187 = local read "变频5"() -> (w549:bool)
              n188 = call <vilib>:"Set Unit ID.vi"("error in (no error)"=w546, "unit ID"=u8 5, "Modbus master in"=w547) -> ("error out"=w552:errorcluster, "Modbus master out"=w579:refnum<class "Modbus Master.lvclass">)  [unwired: 7 in]
              n189 = case shown="真" w549 {
                tunnel: w579 -> [w625 w631]
                tunnel: [w624 w630] -> w578
                tunnel: [w625 w629] -> w577
                tunnel: w552 -> [w624 w627]
                frame False {
                }
                frame True {
                  n190 = for {
                    N: 2 -> [_]
                    shift-right: [w633] -> w629
                    shift-left: w631 -> [w637]
                    shift-right: [w634] -> w630
                    shift-left: w627 -> [w632]
                    # "变频器初始化"
                    n191 = call-dynamic "Write Single Holding Register.vi"("error in (no error)"=w632, "holding register value"=u16 1142, "address"=u16 0, "Modbus master in"=w637) -> ("error out"=w634:errorcluster, "Modbus master out"=w633:refnum<class "Modbus Master.lvclass">)  [unwired: 6 in]
                  }
                  n192 = local write "变频5"(FALSE) -> ()
                }
              }
              n193 = flat-sequence {
                tunnel: w578 -> [w639]
                tunnel: [w639] -> w575
                tunnel: w577 -> [w638]
                tunnel: [w638] -> w576
                frame #0 {
                  n194 = Wait (ms)(milliseconds to wait=u32 10 ("等待时间（毫秒）")) -> ()  [unwired: 1 out]
                }
              }
              n195 = case shown="真" "驱动电机上启动" {
                tunnel: w576 -> [w613 w619]
                tunnel: [w612 w616] -> w524
                tunnel: [w608 w615] -> w522
                tunnel: w575 -> [w609 w614]
                frame False {
                  n196 = call-dynamic "Write Single Holding Register.vi"("error in (no error)"=w609, "holding register value"=u16 1143, "address"=u16 0, "Modbus master in"=w613) -> ("error out"=w608:errorcluster, "Modbus master out"=w612:refnum<class "Modbus Master.lvclass">)  [unwired: 6 in]
                }
                frame True {
                  n197 = call-dynamic "Write Single Holding Register.vi"("error in (no error)"=w614, "holding register value"=u16 1151, "address"=u16 0, "Modbus master in"=w619) -> ("error out"=w615:errorcluster, "Modbus master out"=w616:refnum<class "Modbus Master.lvclass">)  [unwired: 6 in]
                }
              }
              n198 = flat-sequence {
                tunnel: w522 -> [w604]
                tunnel: [w604] -> w521
                tunnel: w524 -> [w603]
                tunnel: [w603] -> w523
                frame #0 {
                  n199 = Wait (ms)(milliseconds to wait=u32 10 ("等待时间（毫秒）")) -> ()  [unwired: 1 out]
                }
              }
              n200 = case shown="假" "驱动电机上正反转" {
                tunnel: [w620 w623] -> w573
                frame False {
                  n201 = local read "驱动电机上转速给定"() -> (w620:i16)
                }
                frame True {
                  n202 = Multiply(x="驱动电机上转速给定", y=i16 -1) -> (x*y=w623:i16)
                }
              }
              n203 = call-dynamic "Write Single Holding Register.vi"("error in (no error)"=w521, "holding register value"=w573, "address"=u16 1, "Modbus master in"=w523) -> ("error out"=w539:errorcluster, "Modbus master out"=w540:refnum<class "Modbus Master.lvclass">)  [unwired: 6 in]
              n204 = call-dynamic "Read Holding Registers.vi"("error in (no error)"=w539, "number of holding registers"=u16 2, "starting address"=u16 109, "Modbus master in"=w540) -> ("error out"=w551:errorcluster, "register values"=w561:u16[], "Modbus master out"=w556:refnum<class "Modbus Master.lvclass">)  [unwired: 5 in]
              n205 = Index Array(array=w561) -> (element #1=→"驱动转矩上监控":u16, element #2=w560:u16)  [unwired: 2 in]
              n206 = Divide(x=w560, y=u16 10) -> (x/y=→"驱动电机上母线电压":dbl)
              n207 = local read "当前试验档位"() -> (w515:string)
              n208 = local read "当前试验档位"() -> (w516:string)
              n209 = local read "当前试验档位"() -> (w517:string)
              n210 = local read "当前试验档位"() -> (w518:string)
              n211 = call-dynamic "Read Holding Registers.vi"("error in (no error)"=w551, "number of holding registers"=u16 1, "starting address"=u16 106, "Modbus master in"=w556) -> ("error out"=w538:errorcluster, "register values"=w555:u16[], "Modbus master out"=w520:refnum<class "Modbus Master.lvclass">)  [unwired: 5 in]
              n212 = Index Array(array=w555) -> (element #1=w554:u16)  [unwired: 2 in, 1 out]
              n213 = Multiply(x=w554, y=0.3) -> (x*y=→"驱动电机上母线电流":dbl)
              n214 = case shown="\"D6\"" w515 {
                tunnel: [w581 w582 w583 w587] -> _
                frame "D5" {
                  n215 = local read "D4平均速度"() -> (w581:dbl)
                }
                frame "D6" {
                  n216 = local read "D4平均速度"() -> (w582:dbl)
                  n217 = local write "驱动电机上转速给定"(w582) -> ()
                }
                frame "N" {
                  n218 = local read "加载左上转速监控"() -> (w583:dbl)
                }
                frame "D1", "D2", "D3", "D4", Default {
                  n219 = local read "加载左上转速监控"() -> (w586:dbl)
                  n220 = Multiply(x=w586, y=1.0) -> (x*y=w584:dbl)
                  n221 = To Word Integer(number=w584) -> (16bit integer=w587:i16)
                }
              }
              n222 = case shown="\"D5\", \"D6 \"" w516 {
                tunnel: [w588 w592] -> _
                frame "D5", "D6 " {
                  n223 = local read "D4平均速度"() -> (w588:dbl)
                }
                frame "D1", "D2", "D3", "D4", Default {
                  n224 = local read "加载左上转速监控"() -> (w591:dbl)
                  n225 = Multiply(x=w591, y=1.0) -> (x*y=w589:dbl)
                  n226 = To Word Integer(number=w589) -> (16bit integer=w592:i16)
                }
              }
              n227 = case shown="\"D5\", \"D6 \"" w517 {
                tunnel: [w593 w597] -> _
                frame "D5", "D6 " {
                  n228 = local read "D4平均速度"() -> (w593:dbl)
                }
                frame "D1", "D2", "D3", "D4", Default {
                  n229 = local read "加载左上转速监控"() -> (w596:dbl)
                  n230 = Multiply(x=w596, y=1.0) -> (x*y=w594:dbl)
                  n231 = To Word Integer(number=w594) -> (16bit integer=w597:i16)
                }
              }
              n232 = case shown="\"D5\", \"D6 \"" w518 {
                tunnel: [w598 w602] -> w534
                frame "D5", "D6 " {
                  n233 = local read "D4平均速度"() -> (w598:dbl)
                }
                frame "D1", "D2", "D3", "D4", Default {
                  n234 = local read "加载左上转速监控"() -> (w601:dbl)
                  n235 = Multiply(x=w601, y=1.0) -> (x*y=w599:dbl)
                  n236 = To Word Integer(number=w599) -> (16bit integer=w602:i16)
                }
              }
              n237 = Wait (ms)(milliseconds to wait=u32 50 ("等待时间（毫秒）")) -> ()  [unwired: 1 out]
              n238 = call-dynamic "Read Holding Registers.vi"("error in (no error)"=w538, "number of holding registers"=u16 2, "starting address"=u16 20200 ("address"), "Modbus master in"=w520) -> ("error out"=w519:errorcluster, "register values"=w570:u16[], "Modbus master out"=w525:refnum<class "Modbus Master.lvclass">)  [unwired: 5 in]
              n239 = Index Array(array=w570) -> (element #1=w567:u16, element #2=w569:u16)  [unwired: 2 in]
              n240 = Multiply(x=w569, y=u32 65536) -> (x*y=w566:u32)
              n241 = Add(x=w567, y=w566) -> (x+y=w565:u32)
              n242 = To Long Integer(number=w565) -> (32bit integer=w564:i32)
              n243 = Divide(x=w564, y=100) -> (x/y=→"驱动上转速监控" →"前左":dbl)
              n244 = local write "驱动电机上转速给定"(w534) -> ()
              n245 = call-dynamic "Read Holding Registers.vi"("error in (no error)"=w519, "number of holding registers"=u16 2, "starting address"=u16 420, "Modbus master in"=w525) -> ("error out"=w514:errorcluster, "register values"=w529:u16[], "Modbus master out"=w513:refnum<class "Modbus Master.lvclass">)  [unwired: 5 in]
              n246 = Index Array(array=w529) -> (element #1=w528:u16, element #2=w527:u16)  [unwired: 2 in]
              n247 = call-dynamic "Read Holding Registers.vi"("error in (no error)"=w514, "number of holding registers"=u16 1, "starting address"=u16 615, "Modbus master in"=w513) -> ("error out"=w511:errorcluster, "register values"=w508:u16[], "Modbus master out"=w512:refnum<class "Modbus Master.lvclass">)  [unwired: 5 in]
              n248 = Add(x=w528, y=w527) -> (x+y=w532:u16)
              n249 = Greater Than 0?(x=w532) -> (x > 0?=w526:bool)
              n250 = case shown="真" w526 {
                frame False {
                  n251 = local write "变频故障5"(FALSE ("变频故障5")) -> ()
                }
                frame True {
                  "变频故障5" <- TRUE ("变频故障5")
                }
              }
              n252 = call <vilib>:"Set Timeouts.vi"("error in (no error)"=w511, "write operation timeout (ms)"=w537, "read operation timeout (ms)"=w537, "Modbus master in"=w512) -> ("error out"=w541:errorcluster, "Modbus master out"=w548:refnum<class "Modbus Master.lvclass">)  [unwired: 6 in]
              n253 = Index Array(array=w508) -> (element=w507:u16)  [unwired: 1 in]
              n254 = Number To Boolean Array(number=w507) -> (Boolean array=w506:bool[])
              "前左" <- w506
              n255 = Index Array(array=w506, index=5 ("索引")) -> (element=→"前左":bool)
            }
            frame 6 {
              w672 = 200 ("read operation timeout (ms)")
              n256 = local read "变频6"() -> (w715:bool)
              n257 = call <vilib>:"Set Unit ID.vi"("error in (no error)"=w682, "unit ID"=u8 6, "Modbus master in"=w683) -> ("error out"=w712:errorcluster, "Modbus master out"=w685:refnum<class "Modbus Master.lvclass">)  [unwired: 7 in]
              n258 = case shown="真" w715 {
                tunnel: w685 -> [w744 w750]
                tunnel: [w743 w749] -> w686
                tunnel: [w744 w748] -> w687
                tunnel: w712 -> [w743 w746]
                frame False {
                }
                frame True {
                  n259 = for {
                    N: 2 -> [_]
                    shift-right: [w752] -> w748
                    shift-left: w750 -> [w756]
                    shift-right: [w753] -> w749
                    shift-left: w746 -> [w751]
                    # "变频器初始化"
                    n260 = call-dynamic "Write Single Holding Register.vi"("error in (no error)"=w751, "holding register value"=u16 1142, "address"=u16 0, "Modbus master in"=w756) -> ("error out"=w753:errorcluster, "Modbus master out"=w752:refnum<class "Modbus Master.lvclass">)  [unwired: 6 in]
                  }
                  n261 = local write "变频6"(FALSE) -> ()
                }
              }
              n262 = flat-sequence {
                tunnel: w686 -> [w758]
                tunnel: [w758] -> w689
                tunnel: w687 -> [w757]
                tunnel: [w757] -> w688
                frame #0 {
                  n263 = Wait (ms)(milliseconds to wait=u32 10 ("等待时间（毫秒）")) -> ()  [unwired: 1 out]
                }
              }
              n264 = case shown="假" "驱动电机下启动" {
                tunnel: w688 -> [w732 w738]
                tunnel: [w731 w735] -> w659
                tunnel: [w727 w734] -> w657
                tunnel: w689 -> [w728 w733]
                frame False {
                  n265 = call-dynamic "Write Single Holding Register.vi"("error in (no error)"=w728, "holding register value"=u16 1143, "address"=u16 0, "Modbus master in"=w732) -> ("error out"=w727:errorcluster, "Modbus master out"=w731:refnum<class "Modbus Master.lvclass">)  [unwired: 6 in]
                }
                frame True {
                  n266 = call-dynamic "Write Single Holding Register.vi"("error in (no error)"=w733, "holding register value"=u16 1151, "address"=u16 0, "Modbus master in"=w738) -> ("error out"=w734:errorcluster, "Modbus master out"=w735:refnum<class "Modbus Master.lvclass">)  [unwired: 6 in]
                }
              }
              n267 = flat-sequence {
                tunnel: w657 -> [w723]
                tunnel: [w723] -> w656
                tunnel: w659 -> [w722]
                tunnel: [w722] -> w658
                frame #0 {
                  n268 = Wait (ms)(milliseconds to wait=u32 10 ("等待时间（毫秒）")) -> ()  [unwired: 1 out]
                }
              }
              n269 = case shown="真" "驱动电机下正反转" {
                tunnel: [w739 w742] -> w691
                frame False {
                  n270 = local read "驱动电机转速下给定"() -> (w739:i16)
                }
                frame True {
                  n271 = Multiply(x="驱动电机转速下给定", y=i8 -1) -> (x*y=w742:i16)
                }
              }
              n272 = call-dynamic "Write Single Holding Register.vi"("error in (no error)"=w656, "holding register value"=w691, "address"=u16 1, "Modbus master in"=w658) -> ("error out"=w674:errorcluster, "Modbus master out"=w675:refnum<class "Modbus Master.lvclass">)  [unwired: 6 in]
              n273 = call-dynamic "Read Holding Registers.vi"("error in (no error)"=w674, "number of holding registers"=u16 2, "starting address"=u16 109, "Modbus master in"=w675) -> ("error out"=w713:errorcluster, "register values"=w703:u16[], "Modbus master out"=w708:refnum<class "Modbus Master.lvclass">)  [unwired: 5 in]
              n274 = Index Array(array=w703) -> (element #1=→"驱动转矩下监控":u16, element #2=w704:u16)  [unwired: 2 in]
              n275 = Divide(x=w704, y=u16 10) -> (x/y=→"驱动电机下母线电压":dbl)
              n276 = local read "当前试验档位"() -> (w654:string)
              n277 = call-dynamic "Read Holding Registers.vi"("error in (no error)"=w713, "number of holding registers"=u16 1, "starting address"=u16 106, "Modbus master in"=w708) -> ("error out"=w673:errorcluster, "register values"=w709:u16[], "Modbus master out"=w660:refnum<class "Modbus Master.lvclass">)  [unwired: 5 in]
              n278 = Index Array(array=w709) -> (element #1=w710:u16)  [unwired: 2 in, 1 out]
              n279 = case shown="\"D5\", \"D6\"" w654 {
                tunnel: [w716 w717 w718] -> w653
                frame "D5", "D6" {
                  n280 = local read "D4平均速度"() -> (w716:dbl)
                }
                frame "N" {
                  n281 = local read "加载左上转速监控"() -> (w717:dbl)
                }
                frame "D1", "D2", "D3", "D4", Default {
                  n282 = local read "加载左上转速监控"() -> (w721:dbl)
                  n283 = Multiply(x=w721, y=1.0) -> (x*y=w719:dbl)
                  n284 = To Word Integer(number=w719) -> (16bit integer=w718:i16)
                }
              }
              n285 = Multiply(x=w710, y=0.3) -> (x*y=→"驱动电机下母线电流":dbl)
              n286 = local write "驱动电机转速下给定"(w653) -> ()
              n287 = call-dynamic "Read Holding Registers.vi"("error in (no error)"=w673, "number of holding registers"=u16 2, "starting address"=u16 20200 ("address"), "Modbus master in"=w660) -> ("error out"=w655:errorcluster, "register values"=w694:u16[], "Modbus master out"=w661:refnum<class "Modbus Master.lvclass">)  [unwired: 5 in]
              n288 = Index Array(array=w694) -> (element #1=w697:u16, element #2=w695:u16)  [unwired: 2 in]
              n289 = Multiply(x=w695, y=u32 65536) -> (x*y=w698:u32)
              n290 = Add(x=w697, y=w698) -> (x+y=w699:u32)
              n291 = To Long Integer(number=w699) -> (32bit integer=w700:i32)
              n292 = Divide(x=w700, y=100) -> (x/y=→"驱动转速下监控" →"前右":dbl)
              n293 = call-dynamic "Read Holding Registers.vi"("error in (no error)"=w655, "number of holding registers"=u16 2, "starting address"=u16 420, "Modbus master in"=w661) -> ("error out"=w651:errorcluster, "register values"=w665:u16[], "Modbus master out"=w652:refnum<class "Modbus Master.lvclass">)  [unwired: 5 in]
              n294 = call-dynamic "Read Holding Registers.vi"("error in (no error)"=w651, "number of holding registers"=u16 1, "starting address"=u16 615, "Modbus master in"=w652) -> ("error out"=w641:errorcluster, "register values"=w647:u16[], "Modbus master out"=w650:refnum<class "Modbus Master.lvclass">)  [unwired: 5 in]
              n295 = call <vilib>:"Set Timeouts.vi"("error in (no error)"=w641, "write operation timeout (ms)"=w672, "read operation timeout (ms)"=w672, "Modbus master in"=w650) -> ("error out"=w676:errorcluster, "Modbus master out"=w681:refnum<class "Modbus Master.lvclass">)  [unwired: 6 in]
              n296 = Wait (ms)(milliseconds to wait=u32 50 ("等待时间（毫秒）")) -> ()  [unwired: 1 out]
              n297 = Index Array(array=w665) -> (element #1=w664:u16, element #2=w663:u16)  [unwired: 2 in]
              n298 = Add(x=w664, y=w663) -> (x+y=w668:u16)
              n299 = Greater Than 0?(x=w668) -> (x > 0?=w662:bool)
              n300 = case shown="真" w662 {
                frame False {
                  n301 = local write "变频故障 6"(FALSE ("变频故障 6")) -> ()
                }
                frame True {
                  "变频故障 6" <- TRUE ("变频故障 6")
                }
              }
              n302 = Not(x=w641) -> (.not. x?=→"变频器":bool)
              n303 = Index Array(array=w647) -> (element=w646:u16)  [unwired: 1 in]
              n304 = Number To Boolean Array(number=w646) -> (Boolean array=w645:bool[])
              "前右" <- w645
              n305 = Index Array(array=w645, index=5 ("索引")) -> (element=→"前右":bool)
            }
          }
        }
        n306 = case shown="真" w50 {
          frame False {
          }
          frame True {
            "485启动给遥控器布尔" <- TRUE ("485启动给遥控器布尔")
          }
        }
        n307 = local read "停止"() -> (w59:bool)
        "数值" <- w52
      }
    }
  }
  n308 = Obtain Queue(name (unnamed)="LED" ("名称（未命名）"), element data type=0) -> (queue out=w20:refnum<queue>)  [unwired: 3 in, 2 out]
  n309 = TCP Open Connection(address="192.168.1.200" ("地址"), remote port or service name=u16 10001 ("远程端口或服务名称")) -> (connection ID=w18:refnum<k5>)  [unwired: 3 in, 1 out]
  n310 = Obtain Queue(name (unnamed)="LED" ("名称（未命名）"), element data type=0) -> (queue out=w10:refnum<queue>)  [unwired: 3 in, 2 out]
  n311 = while {
    shift-right: [w785] -> w11
    shift-left: w20 -> [w781]
    tunnel: w18 -> [w786]
    shift-right: [w783] -> _
    shift-left: dbl[] [] -> [w782]
    i -> [w760]
    stop <- w787 stop-if-true
    n312 = local read "comcnt"() -> (w763:u16)
    n313 = local read "变矩器出口温度标定"() -> (w770:dbl)
    n314 = local read "右前轮轴承温度标定"() -> (w769:dbl)
    n315 = local read "左前轮轴承温度标定"() -> (w768:dbl)
    n316 = Dequeue Element(queue=w781) -> (queue out=w767:refnum<queue>, element=w765:i32)  [unwired: 2 in, 2 out]
    n317 = Greater?(x=w763, y=u16 100) -> (0:w761:bool)
    n318 = case shown="真" w761 {
      tunnel: w767 -> [w789 w792]
      tunnel: [w789 w791] -> w766
      tunnel: w765 -> [w788 _]
      tunnel: [w788 45] -> w764
      frame False {
      }
      frame True {
        n319 = Flush Queue(queue=w792) -> (queue out=w791:refnum<queue>)  [unwired: 1 in, 2 out]
      }
    }
    n320 = Merge Signals(w770, w769, w768) -> (→"波形图表":dynamicdata)
    n321 = local read "变频故障1"() -> (w772:bool)
    n322 = local read "变频故障2"() -> (w773:bool)
    n323 = local read "变频故障 3"() -> (w774:bool)
    n324 = local read "变频故障 4"() -> (w775:bool)
    n325 = local read "变频故障5"() -> (w776:bool)
    n326 = local read "变频故障 6"() -> (w777:bool)
    n327 = Compound Arithmetic op=OR ("复合运算")(w772, w773, w774, w775, w776, w777) -> (w771:bool)
    n328 = case shown="假" w771 {
      tunnel: w764 -> [w794 _]
      tunnel: [w794 44] -> w779
      tunnel: w766 -> [w793 w797]
      tunnel: [w793 w796] -> w778
      frame False {
      }
      frame True {
        n329 = Flush Queue(queue=w797) -> (queue out=w796:refnum<queue>)  [unwired: 1 in, 2 out]
      }
    }
    n330 = case shown="43" w779 {
      tunnel: w778 -> [w805 w822 w837 w852 w876 w889 w905 w919 w944 w954 w972 w986 w1010 w1021 w1039 w1052 w1078 w1087 w1105 w1118 w1144 w1155 w1173 w1185 w1211 w1221 w1240 w1255 w1268 w1294 w1303 w1322 w1335 w1355 w1371 w1389 w1401 w1422 w1438 w1456 w1467 w1476 w1482 w1490 w1496]
      tunnel: w786 -> [w807 w823 w839 w853 w878 w890 w906 w920 w945 w956 w973 w987 w1012 w1024 w1040 w1054 w1079 w1090 w1107 w1121 w1146 w1158 w1174 w1188 w1213 w1224 w1241 w1257 w1271 w1295 w1306 w1323 w1337 w1362 w1374 w1390 w1404 w1429 w1440 w1457 w1468 w1477 w1485 w1492 w1499]
      tunnel: [w804 w821 w836 w850 w877 w888 w904 w917 w943 w953 w971 w985 w1009 w1020 w1038 w1053 w1077 w1086 w1104 w1117 w1143 w1154 w1172 w1184 w1210 w1220 w1239 w1254 w1267 w1293 w1302 w1321 w1334 w1354 w1370 w1388 w1400 w1423 w1437 w1455 w1467 w1476 w1481 w1489 w1496] -> w785
      tunnel: [dbl[] [] dbl[] [] dbl[] [] dbl[] [] w872 dbl[] [] dbl[] [] dbl[] [] w937 dbl[] [] dbl[] [] dbl[] [] w1004 dbl[] [] dbl[] [] dbl[] [] w1071 dbl[] [] dbl[] [] dbl[] [] w1138 dbl[] [] dbl[] [] dbl[] [] w1205 dbl[] [] dbl[] [] dbl[] [] dbl[] [] w1287 dbl[] [] dbl[] [] dbl[] [] w1357 dbl[] [] dbl[] [] dbl[] [] w1424 dbl[] [] dbl[] [] dbl[] [] dbl[] [] dbl[] [] w1491 dbl[] []] -> w783
      tunnel: w782 -> [_ _ _ _ w873 _ _ _ w938 _ _ _ w1005 _ _ _ w1072 _ _ _ w1139 _ _ _ w1206 _ _ _ _ w1288 _ _ _ w1358 _ _ _ w1425 _ _ _ _ _ w1491 _]
      frame 2 {
        n331 = local read "等待进车布尔"() -> (w798:bool)
        n332 = local read "遥控器按钮确认"() -> (w800:bool)
        n333 = case shown="真" w798 {
          tunnel: w807 -> [_ w812]
          frame False {
          }
          frame True {
            w808 = "等待进车"
            n334 = local write "等待进车布尔"(FALSE ("等待进车布尔")) -> ()
            n335 = call "led显示更新字符串山推.vi"("显示字符"=w808, "立显/保存"=TRUE) -> ("发送数据"=w811:string)  [unwired: 9 in]
            n336 = local write "LED屏幕信息"(w808) -> ()
            n337 = call "led发送数据并接收返回山推.vi"("发送数据"=w811, "TCP网络连接输入"=w812) -> ()  [unwired: 8 in, 2 out]
          }
        }
        n338 = call <vilib>:"Boolean Crossing PtByPt.vi"("direction"=enum16{"either", "false-true", "true-false"}."false-true", "input"=w800) -> ("crossing"=w801:bool)  [unwired: 1 in]
        n339 = case shown="假" w801 {
          tunnel: [2 3] -> w806
          frame False {
          }
          frame True {
          }
        }
        n340 = Enqueue Element(queue=w805, element=w806) -> (queue out=w804:refnum<queue>)  [unwired: 2 in, 2 out]
        "字符布尔" <- TRUE ("字符布尔")
      }
      frame 3 {
        n341 = local read "遥控器按钮确认"() -> (w816:bool)
        n342 = local read "字符布尔"() -> (w815:bool)
        n343 = case shown="真" w815 {
          tunnel: w823 -> [_ w828]
          frame False {
          }
          frame True {
            w824 = "请落下举升，油缸浮动，车辆系固，连接传感器"
            n344 = local write "字符布尔"(FALSE ("字符布尔")) -> ()
            n345 = call "led显示更新字符串山推.vi"("显示字符"=w824, "立显/保存"=TRUE) -> ("发送数据"=w827:string)  [unwired: 9 in]
            n346 = call "led发送数据并接收返回山推.vi"("发送数据"=w827, "TCP网络连接输入"=w828) -> ()  [unwired: 8 in, 2 out]
            n347 = local write "LED屏幕信息"(w824) -> ()
          }
        }
        n348 = call <vilib>:"Boolean Crossing PtByPt.vi"("direction"=enum16{"either", "false-true", "true-false"}."false-true", "input"=w816) -> ("crossing"=w817:bool)  [unwired: 1 in]
        n349 = case shown="真" w817 {
          tunnel: [3 4] -> w820
          frame False {
          }
          frame True {
          }
        }
        n350 = Enqueue Element(queue=w822, element=w820) -> (queue out=w821:refnum<queue>)  [unwired: 2 in, 2 out]
      }
      frame 4 {
        # "here need it to be true"
        n351 = local read "遥控器按钮确认"() -> (w832:bool)
        n352 = local read "字符布尔"() -> (w831:bool)
        n353 = call <vilib>:"Boolean Crossing PtByPt.vi"("direction"=enum16{"either", "false-true", "true-false"}."false-true", "input"=w832) -> ("crossing"=w833:bool)  [unwired: 1 in]
        n354 = case shown="假" w831 {
          tunnel: w839 -> [w844 _]
          frame False {
            w840 = "车挂一档，转速在2000转"
            n355 = local write "字符布尔"(TRUE ("字符布尔")) -> ()
            n356 = call "led显示更新字符串山推.vi"("显示字符"=w840, "立显/保存"=TRUE) -> ("发送数据"=w843:string)  [unwired: 9 in]
            n357 = local write "LED屏幕信息"(w840) -> ()
            n358 = call "led发送数据并接收返回山推.vi"("发送数据"=w843, "TCP网络连接输入"=w844) -> ()  [unwired: 8 in, 2 out]
          }
          frame True {
          }
        }
        n359 = case shown="真" w833 {
          tunnel: [4 5] -> w838
          frame False {
          }
          frame True {
          }
        }
        n360 = Enqueue Element(queue=w837, element=w838) -> (queue out=w836:refnum<queue>)  [unwired: 2 in, 2 out]
      }
      frame 5 {
        n361 = local read "当前试验档位"() -> (w849:string)
        n362 = local read "字符布尔"() -> (w847:bool)
        n363 = case shown="\"假\", 默认" w849 {
          tunnel: [5 6] -> w851
          frame "假", Default {
          }
          frame "D1" {
          }
        }
        n364 = case shown="真" w847 {
          tunnel: w853 -> [_ w856]
          frame False {
          }
          frame True {
            w854 = "遥控器请选择D1档"
            n365 = local write "字符布尔"(FALSE ("字符布尔")) -> ()
            n366 = call "led显示更新字符串山推.vi"("显示字符"=w854, "立显/保存"=TRUE) -> ("发送数据"=w858:string)  [unwired: 9 in]
            n367 = call "led发送数据并接收返回山推.vi"("发送数据"=w858, "TCP网络连接输入"=w856) -> ()  [unwired: 8 in, 2 out]
            n368 = local write "LED屏幕信息"(w854) -> ()
          }
        }
        n369 = Enqueue Element(queue=w852, element=w851) -> (queue out=w850:refnum<queue>)  [unwired: 2 in, 2 out]
      }
      frame 6 {
        n370 = local read "D1S"() -> (w863:dbl)
        n371 = local write "字符布尔"(TRUE ("字符布尔")) -> ()
        n372 = call "已用时间"("Time Target (s)"=w863, "Reset"="Reset") -> ("Time has Elapsed"=w869:bool, "Elapsed Time Text"=w867:string)  [unwired: 10 in, 6 out]
        n373 = local read "加载左上转速监控"() -> (w874:dbl)
        n374 = call "输出文本.vi"("当前档位"="D1" ("字符串"), "字符串"=w867) -> ("输出文本"=w862:string)  [unwired: 9 in]
        n375 = local write "Reset"(FALSE ("Reset")) -> ()
        n376 = call "led显示更新字符串山推.vi"("显示字符"=w862, "立显/保存"=FALSE) -> ("发送数据"=w880:string)  [unwired: 9 in]
        n377 = local write "LED屏幕信息"(w862) -> ()
        n378 = case shown="真" w869 {
          tunnel: [6 7] -> w875
          frame False {
          }
          frame True {
            n379 = local write "Reset"(TRUE ("Reset")) -> ()
          }
        }
        n380 = call "led发送数据并接收返回山推.vi"("发送数据"=w880, "TCP网络连接输入"=w878) -> ()  [unwired: 8 in, 2 out]
        n381 = Build Array (concatenate)(w873, w874) -> (w872:dbl[])
        n382 = Array Size(array=w872) -> (size(s)=w861:i32)
        n383 = Add Array Elements(numeric array=w872) -> (sum=w871:dbl)
        n384 = Divide(x=w871, y=w861) -> (x/y=→"D1平均速度":dbl)
        n385 = Enqueue Element(queue=w876, element=w875) -> (queue out=w877:refnum<queue>)  [unwired: 2 in, 2 out]
      }
      frame 7 {
        n386 = local read "字符布尔"() -> (w884:bool)
        n387 = local read "当前试验档位"() -> (w885:string)
        n388 = case shown="真" w884 {
          tunnel: w890 -> [_ w893]
          frame False {
          }
          frame True {
            w891 = "遥控器请挂空挡" ("显示字符")
            n389 = local write "字符布尔"(FALSE ("字符布尔 2")) -> ()
            n390 = call "led显示更新字符串山推.vi"("显示字符"=w891, "立显/保存"=TRUE) -> ("发送数据"=w895:string)  [unwired: 9 in]
            n391 = local write "LED屏幕信息"(w891) -> ()
            n392 = call "led发送数据并接收返回山推.vi"("发送数据"=w895, "TCP网络连接输入"=w893) -> ()  [unwired: 8 in, 2 out]
          }
        }
        n393 = case shown="\"假\", 默认" w885 {
          tunnel: [7 8] -> w887
          frame "假", Default {
          }
          frame "N" {
          }
        }
        n394 = Enqueue Element(queue=w889, element=w887) -> (queue out=w888:refnum<queue>)  [unwired: 2 in, 2 out]
      }
      frame 8 {
        n395 = local read "字符布尔"() -> (w898:bool)
        n396 = local read "遥控器按钮确认"() -> (w901:bool)
        n397 = case shown="假" w898 {
          tunnel: w906 -> [w909 _]
          frame False {
            w907 = "请车挂二档，转速在2000转"
            n398 = local write "字符布尔"(TRUE ("字符布尔")) -> ()
            n399 = call "led显示更新字符串山推.vi"("显示字符"=w907, "立显/保存"=TRUE) -> ("发送数据"=w911:string)  [unwired: 9 in]
            n400 = local write "LED屏幕信息"(w907) -> ()
            n401 = call "led发送数据并接收返回山推.vi"("发送数据"=w911, "TCP网络连接输入"=w909) -> ()  [unwired: 8 in, 2 out]
          }
          frame True {
          }
        }
        n402 = call <vilib>:"Boolean Crossing PtByPt.vi"("direction"=enum16{"either", "false-true", "true-false"}."false-true", "input"=w901) -> ("crossing"=w900:bool)  [unwired: 1 in]
        n403 = case shown="假" w900 {
          tunnel: [8 9] -> w899
          frame False {
          }
          frame True {
          }
        }
        n404 = Enqueue Element(queue=w905, element=w899) -> (queue out=w904:refnum<queue>)  [unwired: 2 in, 2 out]
      }
      frame 9 {
        n405 = local read "字符布尔"() -> (w914:bool)
        n406 = local read "当前试验档位"() -> (w916:string)
        n407 = case shown="真" w914 {
          tunnel: w920 -> [_ w923]
          frame False {
          }
          frame True {
            w921 = "请将遥控器挂D2档"
            n408 = local write "LED屏幕信息"(w921) -> ()
            n409 = call "led显示更新字符串山推.vi"("显示字符"=w921, "立显/保存"=TRUE) -> ("发送数据"=w925:string)  [unwired: 9 in]
            n410 = local write "字符布尔"(FALSE ("字符布尔")) -> ()
            n411 = call "led发送数据并接收返回山推.vi"("发送数据"=w925, "TCP网络连接输入"=w923) -> ()  [unwired: 8 in, 2 out]
          }
        }
        n412 = case shown="\"假\", 默认" w916 {
          tunnel: [9 10] -> w918
          frame "假", Default {
          }
          frame "D2" {
          }
        }
        n413 = Enqueue Element(queue=w919, element=w918) -> (queue out=w917:refnum<queue>)  [unwired: 2 in, 2 out]
      }
      frame 10 {
        n414 = local read "D2S"() -> (w930:dbl)
        n415 = call "已用时间2"("Time Target (s)"=w930, "Reset"="Reset 2") -> ("Time has Elapsed"=w934:bool, "Elapsed Time Text"=w935:string)  [unwired: 10 in, 6 out]
        n416 = local read "加载左上转速监控"() -> (w941:dbl)
        n417 = call "输出文本.vi"("当前档位"="D2" ("字符串"), "字符串"=w935) -> ("输出文本"=w929:string)  [unwired: 9 in]
        n418 = local write "Reset 2"(FALSE ("Reset 2")) -> ()
        n419 = local write "字符布尔"(TRUE ("字符布尔")) -> ()
        n420 = case shown="真" w934 {
          tunnel: [10 11] -> w942
          frame False {
          }
          frame True {
            n421 = local write "Reset 2"(TRUE ("Reset 2")) -> ()
          }
        }
        n422 = Build Array (concatenate)(w938, w941) -> (w937:dbl[])
        n423 = Array Size(array=w937) -> (size(s)=w928:i32)
        n424 = Add Array Elements(numeric array=w937) -> (sum=w940:dbl)
        n425 = call "led显示更新字符串山推.vi"("显示字符"=w929, "立显/保存"=FALSE) -> ("发送数据"=w947:string)  [unwired: 9 in]
        n426 = local write "LED屏幕信息"(w929) -> ()
        n427 = call "led发送数据并接收返回山推.vi"("发送数据"=w947, "TCP网络连接输入"=w945) -> ()  [unwired: 8 in, 2 out]
        n428 = Divide(x=w940, y=w928) -> (x/y=→"D2平均速度":dbl)
        n429 = Enqueue Element(queue=w944, element=w942) -> (queue out=w943:refnum<queue>)  [unwired: 2 in, 2 out]
      }
      frame 11 {
        n430 = local read "当前试验档位"() -> (w955:string)
        n431 = local read "字符布尔"() -> (w951:bool)
        n432 = case shown="真" w951 {
          tunnel: w956 -> [_ w960]
          frame False {
          }
          frame True {
            w958 = "遥控器挂空挡"
            n433 = local write "字符布尔"(FALSE ("字符布尔")) -> ()
            n434 = local write "LED屏幕信息"(w958) -> ()
            n435 = call "led显示更新字符串山推.vi"("显示字符"=w958, "立显/保存"=TRUE) -> ("发送数据"=w962:string)  [unwired: 9 in]
            n436 = call "led发送数据并接收返回山推.vi"("发送数据"=w962, "TCP网络连接输入"=w960) -> ()  [unwired: 8 in, 2 out]
          }
        }
        n437 = case shown="\"N\"" w955 {
          tunnel: [11 12] -> w952
          frame "假", Default {
          }
          frame "N" {
          }
        }
        n438 = Enqueue Element(queue=w954, element=w952) -> (queue out=w953:refnum<queue>)  [unwired: 2 in, 2 out]
      }
      frame 12 {
        n439 = local read "遥控器按钮确认"() -> (w967:bool)
        n440 = local read "字符布尔"() -> (w965:bool)
        n441 = case shown="假" w965 {
          tunnel: w973 -> [w976 _]
          frame False {
            w974 = "请车挂三档，转速在2000转"
            n442 = local write "字符布尔"(TRUE ("字符布尔")) -> ()
            n443 = call "led显示更新字符串山推.vi"("显示字符"=w974, "立显/保存"=TRUE) -> ("发送数据"=w978:string)  [unwired: 9 in]
            n444 = local write "LED屏幕信息"(w974) -> ()
            n445 = call "led发送数据并接收返回山推.vi"("发送数据"=w978, "TCP网络连接输入"=w976) -> ()  [unwired: 8 in, 2 out]
          }
          frame True {
          }
        }
        n446 = call <vilib>:"Boolean Crossing PtByPt.vi"("direction"=enum16{"either", "false-true", "true-false"}."false-true", "input"=w967) -> ("crossing"=w966:bool)  [unwired: 1 in]
        n447 = case shown="假" w966 {
          tunnel: [12 13] -> w970
          frame False {
          }
          frame True {
          }
        }
        n448 = Enqueue Element(queue=w972, element=w970) -> (queue out=w971:refnum<queue>)  [unwired: 2 in, 2 out]
      }
      frame 13 {
        n449 = local read "当前试验档位"() -> (w983:string)
        n450 = local read "字符布尔"() -> (w981:bool)
        n451 = case shown="\"D3\"" w983 {
          tunnel: [13 14] -> w984
          frame "假", Default {
          }
          frame "D3" {
          }
        }
        n452 = case shown="真" w981 {
          tunnel: w987 -> [_ w990]
          frame False {
          }
          frame True {
            w988 = "遥控器挂三档"
            n453 = local write "字符布尔"(FALSE ("字符布尔")) -> ()
            n454 = local write "LED屏幕信息"(w988) -> ()
            n455 = call "led显示更新字符串山推.vi"("显示字符"=w988, "立显/保存"=TRUE) -> ("发送数据"=w992:string)  [unwired: 9 in]
            n456 = call "led发送数据并接收返回山推.vi"("发送数据"=w992, "TCP网络连接输入"=w990) -> ()  [unwired: 8 in, 2 out]
          }
        }
        n457 = Enqueue Element(queue=w986, element=w984) -> (queue out=w985:refnum<queue>)  [unwired: 2 in, 2 out]
      }
      frame 14 {
        n458 = local read "D3S"() -> (w997:dbl)
        n459 = local write "字符布尔"(TRUE ("字符布尔")) -> ()
        n460 = call "已用时间3"("Time Target (s)"=w997, "Reset"="Reset 3") -> ("Time has Elapsed"=w1001:bool, "Elapsed Time Text"=w1002:string)  [unwired: 10 in, 6 out]
        n461 = local write "Reset 3"(FALSE ("Reset 3")) -> ()
        n462 = local read "加载左上转速监控"() -> (w1008:dbl)
        n463 = call "输出文本.vi"("当前档位"="D3" ("字符串"), "字符串"=w1002) -> ("输出文本"=w996:string)  [unwired: 9 in]
        n464 = case shown="真" w1001 {
          tunnel: [14 15] -> w1011
          frame False {
          }
          frame True {
            n465 = local write "Reset 3"(TRUE ("Reset 3")) -> ()
          }
        }
        n466 = Build Array (concatenate)(w1005, w1008) -> (w1004:dbl[])
        n467 = Array Size(array=w1004) -> (size(s)=w995:i32)
        n468 = Add Array Elements(numeric array=w1004) -> (sum=w1007:dbl)
        n469 = call "led显示更新字符串山推.vi"("显示字符"=w996, "立显/保存"=FALSE) -> ("发送数据"=w1014:string)  [unwired: 9 in]
        n470 = local write "LED屏幕信息"(w996) -> ()
        n471 = call "led发送数据并接收返回山推.vi"("发送数据"=w1014, "TCP网络连接输入"=w1012) -> ()  [unwired: 8 in, 2 out]
        n472 = Divide(x=w1007, y=w995) -> (x/y=→"D3平均速度":dbl)
        n473 = Enqueue Element(queue=w1010, element=w1011) -> (queue out=w1009:refnum<queue>)  [unwired: 2 in, 2 out]
      }
      frame 15 {
        n474 = local read "当前试验档位"() -> (w1023:string)
        n475 = local read "字符布尔"() -> (w1018:bool)
        n476 = case shown="\"N\"" w1023 {
          tunnel: [15 16] -> w1022
          frame "假", Default {
          }
          frame "N" {
          }
        }
        n477 = case shown="真" w1018 {
          tunnel: w1024 -> [_ w1027]
          frame False {
          }
          frame True {
            w1025 = "遥控器挂空挡"
            n478 = local write "LED屏幕信息"(w1025) -> ()
            n479 = local write "字符布尔"(FALSE ("字符布尔")) -> ()
            n480 = call "led显示更新字符串山推.vi"("显示字符"=w1025, "立显/保存"=TRUE) -> ("发送数据"=w1029:string)  [unwired: 9 in]
            n481 = call "led发送数据并接收返回山推.vi"("发送数据"=w1029, "TCP网络连接输入"=w1027) -> ()  [unwired: 8 in, 2 out]
          }
        }
        n482 = Enqueue Element(queue=w1021, element=w1022) -> (queue out=w1020:refnum<queue>)  [unwired: 2 in, 2 out]
      }
      frame 16 {
        n483 = local read "遥控器按钮确认"() -> (w1034:bool)
        n484 = local read "字符布尔"() -> (w1032:bool)
        n485 = case shown="假" w1032 {
          tunnel: w1040 -> [w1043 _]
          frame False {
            w1041 = "车挂四档，转速在2000转"
            n486 = local write "字符布尔"(TRUE ("字符布尔")) -> ()
            n487 = local write "LED屏幕信息"(w1041) -> ()
            n488 = call "led显示更新字符串山推.vi"("显示字符"=w1041, "立显/保存"=TRUE) -> ("发送数据"=w1045:string)  [unwired: 9 in]
            n489 = call "led发送数据并接收返回山推.vi"("发送数据"=w1045, "TCP网络连接输入"=w1043) -> ()  [unwired: 8 in, 2 out]
          }
          frame True {
          }
        }
        n490 = call <vilib>:"Boolean Crossing PtByPt.vi"("direction"=enum16{"either", "false-true", "true-false"}."false-true", "input"=w1034) -> ("crossing"=w1033:bool)  [unwired: 1 in]
        n491 = case shown="真" w1033 {
          tunnel: [16 17] -> w1037
          frame False {
          }
          frame True {
          }
        }
        n492 = Enqueue Element(queue=w1039, element=w1037) -> (queue out=w1038:refnum<queue>)  [unwired: 2 in, 2 out]
      }
      frame 17 {
        n493 = local read "当前试验档位"() -> (w1050:string)
        n494 = local read "字符布尔"() -> (w1048:bool)
        n495 = case shown="\"D4\"" w1050 {
          tunnel: [17 ("等待时间（毫秒）") 18 ("等待时间（毫秒）")] -> w1051
          frame "假", Default {
          }
          frame "D4" {
          }
        }
        n496 = case shown="真" w1048 {
          tunnel: w1054 -> [_ w1057]
          frame False {
          }
          frame True {
            w1055 = "遥控器挂D4档"
            n497 = local write "LED屏幕信息"(w1055) -> ()
            n498 = local write "字符布尔"(FALSE ("字符布尔")) -> ()
            n499 = call "led显示更新字符串山推.vi"("显示字符"=w1055, "立显/保存"=TRUE) -> ("发送数据"=w1059:string)  [unwired: 9 in]
            n500 = call "led发送数据并接收返回山推.vi"("发送数据"=w1059, "TCP网络连接输入"=w1057) -> ()  [unwired: 8 in, 2 out]
          }
        }
        n501 = Enqueue Element(queue=w1052, element=w1051) -> (queue out=w1053:refnum<queue>)  [unwired: 2 in, 2 out]
      }
      frame 18 {
        n502 = local read "D4S"() -> (w1064:dbl)
        n503 = local write "字符布尔"(TRUE ("字符布尔")) -> ()
        n504 = call "已用时间4"("Time Target (s)"=w1064, "Reset"="Reset 4") -> ("Time has Elapsed"=w1068:bool, "Elapsed Time Text"=w1069:string)  [unwired: 10 in, 6 out]
        n505 = call "输出文本.vi"("当前档位"="D4" ("字符串"), "字符串"=w1069) -> ("输出文本"=w1063:string)  [unwired: 9 in]
        n506 = local write "Reset 4"(FALSE ("Reset 4")) -> ()
        n507 = local read "加载左上转速监控"() -> (w1075:dbl)
        n508 = case shown="真" w1068 {
          tunnel: [18 19] -> w1076
          frame False {
          }
          frame True {
            n509 = local write "Reset 4"(TRUE ("Reset 4")) -> ()
          }
        }
        n510 = Build Array (concatenate)(w1072, w1075) -> (w1071:dbl[])
        n511 = Array Size(array=w1071) -> (size(s)=w1062:i32)
        n512 = Add Array Elements(numeric array=w1071) -> (sum=w1074:dbl)
        n513 = call "led显示更新字符串山推.vi"("显示字符"=w1063, "立显/保存"=FALSE) -> ("发送数据"=w1081:string)  [unwired: 9 in]
        n514 = local write "LED屏幕信息"(w1063) -> ()
        n515 = Divide(x=w1074, y=w1062) -> (x/y=→"D4平均速度":dbl)
        n516 = call "led发送数据并接收返回山推.vi"("发送数据"=w1081, "TCP网络连接输入"=w1079) -> ()  [unwired: 8 in, 2 out]
        n517 = Enqueue Element(queue=w1078, element=w1076) -> (queue out=w1077:refnum<queue>)  [unwired: 2 in, 2 out]
      }
      frame 19 {
        n518 = local read "当前试验档位"() -> (w1089:string)
        n519 = local read "字符布尔"() -> (w1085:bool)
        n520 = case shown="\"N\"" w1089 {
          tunnel: [19 20] -> w1088
          frame "假", Default {
          }
          frame "N" {
          }
        }
        n521 = case shown="真" w1085 {
          tunnel: w1090 -> [_ w1094]
          frame False {
          }
          frame True {
            w1092 = "遥控器挂空挡"
            n522 = local write "LED屏幕信息"(w1092) -> ()
            n523 = call "led显示更新字符串山推.vi"("显示字符"=w1092, "立显/保存"=TRUE) -> ("发送数据"=w1096:string)  [unwired: 9 in]
            n524 = local write "字符布尔"(FALSE ("字符布尔")) -> ()
            n525 = call "led发送数据并接收返回山推.vi"("发送数据"=w1096, "TCP网络连接输入"=w1094) -> ()  [unwired: 8 in, 2 out]
          }
        }
        n526 = Enqueue Element(queue=w1087, element=w1088) -> (queue out=w1086:refnum<queue>)  [unwired: 2 in, 2 out]
      }
      frame 20 {
        n527 = local read "遥控器按钮确认"() -> (w1101:bool)
        n528 = local read "字符布尔"() -> (w1099:bool)
        n529 = case shown="假" w1099 {
          tunnel: w1107 -> [w1110 _]
          frame False {
            w1108 = "车挂五档，转速在2000转"
            n530 = local write "字符布尔"(TRUE ("字符布尔")) -> ()
            n531 = local write "LED屏幕信息"(w1108) -> ()
            n532 = call "led显示更新字符串山推.vi"("显示字符"=w1108, "立显/保存"=TRUE) -> ("发送数据"=w1112:string)  [unwired: 9 in]
            n533 = call "led发送数据并接收返回山推.vi"("发送数据"=w1112, "TCP网络连接输入"=w1110) -> ()  [unwired: 8 in, 2 out]
          }
          frame True {
          }
        }
        n534 = call <vilib>:"Boolean Crossing PtByPt.vi"("direction"=enum16{"either", "false-true", "true-false"}."false-true", "input"=w1101) -> ("crossing"=w1100:bool)  [unwired: 1 in]
        n535 = case shown="真" w1100 {
          tunnel: [20 21] -> w1106
          frame False {
          }
          frame True {
          }
        }
        n536 = Enqueue Element(queue=w1105, element=w1106) -> (queue out=w1104:refnum<queue>)  [unwired: 2 in, 2 out]
      }
      frame 21 {
        n537 = local read "当前试验档位"() -> (w1120:string)
        n538 = local read "字符布尔"() -> (w1115:bool)
        n539 = case shown="真" w1115 {
          tunnel: w1121 -> [_ w1124]
          frame False {
          }
          frame True {
            w1122 = "遥控器挂D5档"
            n540 = local write "字符布尔"(FALSE ("字符布尔")) -> ()
            n541 = call "led显示更新字符串山推.vi"("显示字符"=w1122, "立显/保存"=TRUE) -> ("发送数据"=w1126:string)  [unwired: 9 in]
            n542 = local write "LED屏幕信息"(w1122) -> ()
            n543 = call "led发送数据并接收返回山推.vi"("发送数据"=w1126, "TCP网络连接输入"=w1124) -> ()  [unwired: 8 in, 2 out]
          }
        }
        n544 = case shown="\"D5\"" w1120 {
          tunnel: [21 22] -> w1119
          frame "假", Default {
          }
          frame "D5" {
          }
        }
        n545 = Enqueue Element(queue=w1118, element=w1119) -> (queue out=w1117:refnum<queue>)  [unwired: 2 in, 2 out]
      }
      frame 22 {
        n546 = local read "D5S"() -> (w1131:dbl)
        n547 = call "已用时间5"("Time Target (s)"=w1131, "Reset"="Reset 5") -> ("Time has Elapsed"=w1135:bool, "Elapsed Time Text"=w1136:string)  [unwired: 10 in, 6 out]
        n548 = call "输出文本.vi"("当前档位"="D5" ("字符串"), "字符串"=w1136) -> ("输出文本"=w1130:string)  [unwired: 9 in]
        n549 = local read "加载左上转速监控"() -> (w1142:dbl)
        n550 = local write "字符布尔"(TRUE ("字符布尔")) -> ()
        n551 = local write "Reset 5"(FALSE ("Reset 5")) -> ()
        n552 = case shown="真" w1135 {
          tunnel: [22 23] -> w1145
          frame False {
          }
          frame True {
            n553 = local write "Reset 5"(TRUE ("Reset 5")) -> ()
          }
        }
        n554 = Build Array (concatenate)(w1139, w1142) -> (w1138:dbl[])
        n555 = Array Size(array=w1138) -> (size(s)=w1129:i32)
        n556 = call "led显示更新字符串山推.vi"("显示字符"=w1130, "立显/保存"=FALSE) -> ("发送数据"=w1148:string)  [unwired: 9 in]
        n557 = Add Array Elements(numeric array=w1138) -> (sum=w1141:dbl)
        n558 = call "led发送数据并接收返回山推.vi"("发送数据"=w1148, "TCP网络连接输入"=w1146) -> ()  [unwired: 8 in, 2 out]
        n559 = Divide(x=w1141, y=w1129) -> (x/y=→"D5平均速度":dbl)
        n560 = local write "LED屏幕信息"(w1130) -> ()
        n561 = Enqueue Element(queue=w1144, element=w1145) -> (queue out=w1143:refnum<queue>)  [unwired: 2 in, 2 out]
      }
      frame 23 {
        n562 = local read "当前试验档位"() -> (w1156:string)
        n563 = local read "字符布尔"() -> (w1152:bool)
        n564 = case shown="\"N\"" w1156 {
          tunnel: [23 24] -> w1153
          frame "假", Default {
          }
          frame "N" {
          }
        }
        n565 = case shown="真" w1152 {
          tunnel: w1158 -> [_ w1161]
          frame False {
          }
          frame True {
            w1159 = "遥控器挂空挡"
            n566 = local write "LED屏幕信息"(w1159) -> ()
            n567 = call "led显示更新字符串山推.vi"("显示字符"=w1159, "立显/保存"=TRUE) -> ("发送数据"=w1163:string)  [unwired: 9 in]
            n568 = call "led发送数据并接收返回山推.vi"("发送数据"=w1163, "TCP网络连接输入"=w1161) -> ()  [unwired: 8 in, 2 out]
            n569 = local write "字符布尔"(FALSE ("字符布尔")) -> ()
          }
        }
        n570 = Enqueue Element(queue=w1155, element=w1153) -> (queue out=w1154:refnum<queue>)  [unwired: 2 in, 2 out]
      }
      frame 24 {
        n571 = local read "遥控器按钮确认"() -> (w1168:bool)
        n572 = local read "字符布尔"() -> (w1166:bool)
        n573 = case shown="假" w1166 {
          tunnel: w1174 -> [w1177 _]
          frame False {
            w1175 = "车挂六档，转速在2000转"
            n574 = local write "字符布尔"(TRUE ("字符布尔")) -> ()
            n575 = local write "LED屏幕信息"(w1175) -> ()
            n576 = call "led显示更新字符串山推.vi"("显示字符"=w1175, "立显/保存"=TRUE) -> ("发送数据"=w1179:string)  [unwired: 9 in]
            n577 = call "led发送数据并接收返回山推.vi"("发送数据"=w1179, "TCP网络连接输入"=w1177) -> ()  [unwired: 8 in, 2 out]
          }
          frame True {
          }
        }
        n578 = call <vilib>:"Boolean Crossing PtByPt.vi"("direction"=enum16{"either", "false-true", "true-false"}."false-true", "input"=w1168) -> ("crossing"=w1167:bool)  [unwired: 1 in]
        n579 = case shown="假" w1167 {
          tunnel: [24 25] -> w1171
          frame False {
          }
          frame True {
          }
        }
        n580 = Enqueue Element(queue=w1173, element=w1171) -> (queue out=w1172:refnum<queue>)  [unwired: 2 in, 2 out]
      }
      frame 25 {
        n581 = local read "当前试验档位"() -> (w1187:string)
        n582 = local read "字符布尔"() -> (w1182:bool)
        n583 = case shown="\"D6\"" w1187 {
          tunnel: [25 26] -> w1186
          frame "假", Default {
          }
          frame "D6" {
          }
        }
        n584 = case shown="真" w1182 {
          tunnel: w1188 -> [_ w1191]
          frame False {
          }
          frame True {
            w1189 = "遥控器挂D6档"
            n585 = local write "字符布尔"(FALSE ("字符布尔")) -> ()
            n586 = call "led显示更新字符串山推.vi"("显示字符"=w1189, "立显/保存"=TRUE) -> ("发送数据"=w1193:string)  [unwired: 9 in]
            n587 = local write "LED屏幕信息"(w1189) -> ()
            n588 = call "led发送数据并接收返回山推.vi"("发送数据"=w1193, "TCP网络连接输入"=w1191) -> ()  [unwired: 8 in, 2 out]
          }
        }
        n589 = Enqueue Element(queue=w1185, element=w1186) -> (queue out=w1184:refnum<queue>)  [unwired: 2 in, 2 out]
      }
      frame 26 {
        n590 = local read "D6S"() -> (w1198:dbl)
        n591 = call "已用时间6"("Time Target (s)"=w1198, "Reset"="Reset 6") -> ("Time has Elapsed"=w1202:bool, "Elapsed Time Text"=w1203:string)  [unwired: 10 in, 6 out]
        n592 = local read "加载左上转速监控"() -> (w1209:dbl)
        n593 = call "输出文本.vi"("当前档位"="D6" ("字符串"), "字符串"=w1203) -> ("输出文本"=w1197:string)  [unwired: 9 in]
        n594 = local write "字符布尔"(TRUE ("字符布尔")) -> ()
        n595 = local write "Reset 6"(FALSE ("Reset 6")) -> ()
        n596 = case shown="真" w1202 {
          tunnel: [26 27] -> w1212
          frame False {
          }
          frame True {
            n597 = local write "Reset 6"(TRUE ("Reset 6")) -> ()
          }
        }
        n598 = Build Array (concatenate)(w1206, w1209) -> (w1205:dbl[])
        n599 = Array Size(array=w1205) -> (size(s)=w1196:i32)
        n600 = call "led显示更新字符串山推.vi"("显示字符"=w1197, "立显/保存"=FALSE) -> ("发送数据"=w1215:string)  [unwired: 9 in]
        n601 = Add Array Elements(numeric array=w1205) -> (sum=w1208:dbl)
        n602 = call "led发送数据并接收返回山推.vi"("发送数据"=w1215, "TCP网络连接输入"=w1213) -> ()  [unwired: 8 in, 2 out]
        n603 = local write "LED屏幕信息"(w1197) -> ()
        n604 = Divide(x=w1208, y=w1196) -> (x/y=→"D6平均速度":dbl)
        n605 = Enqueue Element(queue=w1211, element=w1212) -> (queue out=w1210:refnum<queue>)  [unwired: 2 in, 2 out]
      }
      frame 27 {
        n606 = local read "当前试验档位"() -> (w1223:string)
        n607 = local read "字符布尔"() -> (w1219:bool)
        n608 = case shown="\"N\"" w1223 {
          tunnel: [27 28] -> w1222
          frame "假", Default {
          }
          frame "N" {
          }
        }
        n609 = case shown="真" w1219 {
          tunnel: w1224 -> [_ w1228]
          frame False {
          }
          frame True {
            w1226 = "遥控器挂空挡"
            n610 = local write "字符布尔"(FALSE ("字符布尔")) -> ()
            n611 = call "led显示更新字符串山推.vi"("显示字符"=w1226, "立显/保存"=TRUE) -> ("发送数据"=w1230:string)  [unwired: 9 in]
            n612 = local write "LED屏幕信息"(w1226) -> ()
            n613 = call "led发送数据并接收返回山推.vi"("发送数据"=w1230, "TCP网络连接输入"=w1228) -> ()  [unwired: 8 in, 2 out]
          }
        }
        n614 = Enqueue Element(queue=w1221, element=w1222) -> (queue out=w1220:refnum<queue>)  [unwired: 2 in, 2 out]
      }
      frame 28 {
        n615 = local read "遥控器按钮确认"() -> (w1234:bool)
        n616 = local read "字符布尔"() -> (w1233:bool)
        n617 = call <vilib>:"Boolean Crossing PtByPt.vi"("direction"=enum16{"either", "false-true", "true-false"}."false-true", "input"=w1234) -> ("crossing"=w1235:bool)  [unwired: 1 in]
        n618 = case shown="假" w1233 {
          tunnel: w1241 -> [w1244 _]
          frame False {
            w1242 = "车辆请挂空挡"
            n619 = local write "字符布尔"(TRUE ("字符布尔")) -> ()
            n620 = local write "LED屏幕信息"(w1242) -> ()
            n621 = call "led显示更新字符串山推.vi"("显示字符"=w1242, "立显/保存"=TRUE) -> ("发送数据"=w1246:string)  [unwired: 9 in]
            n622 = call "led发送数据并接收返回山推.vi"("发送数据"=w1246, "TCP网络连接输入"=w1244) -> ()  [unwired: 8 in, 2 out]
          }
          frame True {
          }
        }
        n623 = case shown="真" w1235 {
          tunnel: [28 29] -> w1238
          frame False {
          }
          frame True {
          }
        }
        n624 = Enqueue Element(queue=w1240, element=w1238) -> (queue out=w1239:refnum<queue>)  [unwired: 2 in, 2 out]
      }
      frame 29 {
        n625 = local read "遥控器按钮确认"() -> (w1251:bool)
        n626 = local read "字符布尔"() -> (w1249:bool)
        n627 = case shown="真" w1249 {
          tunnel: w1257 -> [_ w1260]
          frame False {
          }
          frame True {
            w1258 = "车挂负一档，转速在2000转"
            n628 = local write "字符布尔"(FALSE ("字符布尔")) -> ()
            n629 = call "led显示更新字符串山推.vi"("显示字符"=w1258, "立显/保存"=TRUE) -> ("发送数据"=w1262:string)  [unwired: 9 in]
            n630 = local write "LED屏幕信息"(w1258) -> ()
            n631 = call "led发送数据并接收返回山推.vi"("发送数据"=w1262, "TCP网络连接输入"=w1260) -> ()  [unwired: 8 in, 2 out]
          }
        }
        n632 = call <vilib>:"Boolean Crossing PtByPt.vi"("direction"=enum16{"either", "false-true", "true-false"}."false-true", "input"=w1251) -> ("crossing"=w1250:bool)  [unwired: 1 in]
        n633 = case shown="真" w1250 {
          tunnel: [29 30] -> w1256
          frame False {
          }
          frame True {
          }
        }
        n634 = Enqueue Element(queue=w1255, element=w1256) -> (queue out=w1254:refnum<queue>)  [unwired: 2 in, 2 out]
      }
      frame 30 {
        n635 = local read "字符布尔"() -> (w1265:bool)
        n636 = local read "当前试验档位"() -> (w1270:string)
        n637 = case shown="假" w1265 {
          tunnel: w1271 -> [w1274 _]
          frame False {
            w1272 = "遥控器挂F1档"
            n638 = local write "字符布尔"(TRUE ("字符布尔")) -> ()
            n639 = call "led显示更新字符串山推.vi"("显示字符"=w1272, "立显/保存"=TRUE) -> ("发送数据"=w1276:string)  [unwired: 9 in]
            n640 = local write "LED屏幕信息"(w1272) -> ()
            n641 = call "led发送数据并接收返回山推.vi"("发送数据"=w1276, "TCP网络连接输入"=w1274) -> ()  [unwired: 8 in, 2 out]
          }
          frame True {
          }
        }
        n642 = case shown="\"R1\"" w1270 {
          tunnel: [30 31] -> w1269
          frame "假", Default {
          }
          frame "R1" {
          }
        }
        n643 = Enqueue Element(queue=w1268, element=w1269) -> (queue out=w1267:refnum<queue>)  [unwired: 2 in, 2 out]
      }
      frame 31 {
        n644 = local read "R1S"() -> (w1281:dbl)
        n645 = call "已用时间7"("Time Target (s)"=w1281, "Reset"="Reset 7") -> ("Time has Elapsed"=w1284:bool, "Elapsed Time Text"=w1286:string)  [unwired: 10 in, 6 out]
        n646 = call "输出文本.vi"("当前档位"="F1" ("字符串"), "字符串"=w1286) -> ("输出文本"=w1280:string)  [unwired: 9 in]
        n647 = local read "加载左上转速监控"() -> (w1291:dbl)
        n648 = local write "Reset 7"(FALSE ("Reset 7")) -> ()
        n649 = case shown="真" w1284 {
          tunnel: [31 32] -> w1292
          frame False {
          }
          frame True {
            n650 = local write "Reset 7"(TRUE ("Reset 7")) -> ()
          }
        }
        n651 = Build Array (concatenate)(w1288, w1291) -> (w1287:dbl[])
        n652 = Array Size(array=w1287) -> (size(s)=w1279:i32)
        n653 = local write "LED屏幕信息"(w1280) -> ()
        n654 = call "led显示更新字符串山推.vi"("显示字符"=w1280, "立显/保存"=FALSE) -> ("发送数据"=w1297:string)  [unwired: 9 in]
        n655 = Add Array Elements(numeric array=w1287) -> (sum=w1290:dbl)
        n656 = call "led发送数据并接收返回山推.vi"("发送数据"=w1297, "TCP网络连接输入"=w1295) -> ()  [unwired: 8 in, 2 out]
        n657 = Divide(x=w1290, y=w1279) -> (x/y=→"R1平均速度":dbl)
        n658 = Enqueue Element(queue=w1294, element=w1292) -> (queue out=w1293:refnum<queue>)  [unwired: 2 in, 2 out]
      }
      frame 32 {
        n659 = local read "当前试验档位"() -> (w1305:string)
        n660 = local read "字符布尔"() -> (w1301:bool)
        n661 = case shown="\"N\"" w1305 {
          tunnel: [32 33] -> w1304
          frame "假", Default {
          }
          frame "N" {
          }
        }
        n662 = case shown="真" w1301 {
          tunnel: w1306 -> [_ w1310]
          frame False {
          }
          frame True {
            w1308 = "遥控器挂空挡"
            n663 = local write "字符布尔"(FALSE ("字符布尔")) -> ()
            n664 = call "led显示更新字符串山推.vi"("显示字符"=w1308, "立显/保存"=TRUE) -> ("发送数据"=w1312:string)  [unwired: 9 in]
            n665 = local write "LED屏幕信息"(w1308) -> ()
            n666 = call "led发送数据并接收返回山推.vi"("发送数据"=w1312, "TCP网络连接输入"=w1310) -> ()  [unwired: 8 in, 2 out]
          }
        }
        n667 = Enqueue Element(queue=w1303, element=w1304) -> (queue out=w1302:refnum<queue>)  [unwired: 2 in, 2 out]
      }
      frame 33 {
        n668 = local read "遥控器按钮确认"() -> (w1317:bool)
        n669 = local read "字符布尔"() -> (w1315:bool)
        n670 = case shown="假" w1315 {
          tunnel: w1323 -> [w1326 _]
          frame False {
            w1324 = "车挂负二档，转速在2000转"
            n671 = local write "字符布尔"(TRUE ("字符布尔")) -> ()
            n672 = local write "LED屏幕信息"(w1324) -> ()
            n673 = call "led显示更新字符串山推.vi"("显示字符"=w1324, "立显/保存"=TRUE) -> ("发送数据"=w1328:string)  [unwired: 9 in]
            n674 = call "led发送数据并接收返回山推.vi"("发送数据"=w1328, "TCP网络连接输入"=w1326) -> ()  [unwired: 8 in, 2 out]
          }
          frame True {
          }
        }
        n675 = call <vilib>:"Boolean Crossing PtByPt.vi"("direction"=enum16{"either", "false-true", "true-false"}."false-true", "input"=w1317) -> ("crossing"=w1316:bool)  [unwired: 1 in]
        n676 = case shown="真" w1316 {
          tunnel: [33 34] -> w1320
          frame False {
          }
          frame True {
          }
        }
        n677 = Enqueue Element(queue=w1322, element=w1320) -> (queue out=w1321:refnum<queue>)  [unwired: 2 in, 2 out]
      }
      frame 34 {
        n678 = local read "当前试验档位"() -> (w1336:string)
        n679 = local read "字符布尔"() -> (w1331:bool)
        n680 = case shown="\"假\", 默认" w1336 {
          tunnel: [34 35] -> w1333
          frame "假", Default {
          }
          frame "R2" {
          }
        }
        n681 = case shown="真" w1331 {
          tunnel: w1337 -> [_ w1340]
          frame False {
          }
          frame True {
            w1338 = "遥控器挂F2档"
            n682 = local write "字符布尔"(FALSE ("字符布尔")) -> ()
            n683 = call "led显示更新字符串山推.vi"("显示字符"=w1338, "立显/保存"=TRUE) -> ("发送数据"=w1342:string)  [unwired: 9 in]
            n684 = local write "LED屏幕信息"(w1338) -> ()
            n685 = call "led发送数据并接收返回山推.vi"("发送数据"=w1342, "TCP网络连接输入"=w1340) -> ()  [unwired: 8 in, 2 out]
          }
        }
        n686 = Enqueue Element(queue=w1335, element=w1333) -> (queue out=w1334:refnum<queue>)  [unwired: 2 in, 2 out]
      }
      frame 35 {
        n687 = local read "R2S"() -> (w1347:dbl)
        n688 = call "已用时间8"("Time Target (s)"=w1347, "Reset"="Reset 8") -> ("Time has Elapsed"=w1353:bool, "Elapsed Time Text"=w1352:string)  [unwired: 10 in, 6 out]
        n689 = local read "加载左上转速监控"() -> (w1361:dbl)
        n690 = call "输出文本.vi"("当前档位"="F2" ("字符串"), "字符串"=w1352) -> ("输出文本"=w1346:string)  [unwired: 9 in]
        n691 = local write "Reset 8"(FALSE ("Reset 8")) -> ()
        n692 = local write "字符布尔"(TRUE ("字符布尔")) -> ()
        n693 = case shown="真" w1353 {
          tunnel: [35 36] -> w1356
          frame False {
          }
          frame True {
            n694 = local write "Reset 8"(TRUE ("Reset 8")) -> ()
          }
        }
        n695 = Build Array (concatenate)(w1358, w1361) -> (w1357:dbl[])
        n696 = Array Size(array=w1357) -> (size(s)=w1345:i32)
        n697 = call "led显示更新字符串山推.vi"("显示字符"=w1346, "立显/保存"=FALSE) -> ("发送数据"=w1364:string)  [unwired: 9 in]
        n698 = Add Array Elements(numeric array=w1357) -> (sum=w1360:dbl)
        n699 = call "led发送数据并接收返回山推.vi"("发送数据"=w1364, "TCP网络连接输入"=w1362) -> ()  [unwired: 8 in, 2 out]
        n700 = local write "LED屏幕信息"(w1346) -> ()
        n701 = Divide(x=w1360, y=w1345) -> (x/y=→"R2平均速度":dbl)
        n702 = Enqueue Element(queue=w1355, element=w1356) -> (queue out=w1354:refnum<queue>)  [unwired: 2 in, 2 out]
      }
      frame 36 {
        n703 = local read "当前试验档位"() -> (w1373:string)
        n704 = local read "字符布尔"() -> (w1368:bool)
        n705 = case shown="\"N\"" w1373 {
          tunnel: [36 37] -> w1372
          frame "假", Default {
          }
          frame "N" {
          }
        }
        n706 = case shown="真" w1368 {
          tunnel: w1374 -> [_ w1377]
          frame False {
          }
          frame True {
            w1375 = "遥控器挂空挡"
            n707 = local write "字符布尔"(FALSE ("字符布尔")) -> ()
            n708 = local write "LED屏幕信息"(w1375) -> ()
            n709 = call "led显示更新字符串山推.vi"("显示字符"=w1375, "立显/保存"=TRUE) -> ("发送数据"=w1379:string)  [unwired: 9 in]
            n710 = call "led发送数据并接收返回山推.vi"("发送数据"=w1379, "TCP网络连接输入"=w1377) -> ()  [unwired: 8 in, 2 out]
          }
        }
        n711 = Enqueue Element(queue=w1371, element=w1372) -> (queue out=w1370:refnum<queue>)  [unwired: 2 in, 2 out]
      }
      frame 37 {
        n712 = local read "遥控器按钮确认"() -> (w1384:bool)
        n713 = local read "字符布尔"() -> (w1382:bool)
        n714 = case shown="假" w1382 {
          tunnel: w1390 -> [w1393 _]
          frame False {
            w1391 = "车挂负三档，转速在2000转"
            n715 = local write "字符布尔"(TRUE ("字符布尔")) -> ()
            n716 = call "led显示更新字符串山推.vi"("显示字符"=w1391, "立显/保存"=TRUE) -> ("发送数据"=w1395:string)  [unwired: 9 in]
            n717 = local write "LED屏幕信息"(w1391) -> ()
            n718 = call "led发送数据并接收返回山推.vi"("发送数据"=w1395, "TCP网络连接输入"=w1393) -> ()  [unwired: 8 in, 2 out]
          }
          frame True {
          }
        }
        n719 = call <vilib>:"Boolean Crossing PtByPt.vi"("direction"=enum16{"either", "false-true", "true-false"}."false-true", "input"=w1384) -> ("crossing"=w1383:bool)  [unwired: 1 in]
        n720 = case shown="真" w1383 {
          tunnel: [37 38] -> w1387
          frame False {
          }
          frame True {
          }
        }
        n721 = Enqueue Element(queue=w1389, element=w1387) -> (queue out=w1388:refnum<queue>)  [unwired: 2 in, 2 out]
      }
      frame 38 {
        n722 = local read "当前试验档位"() -> (w1403:string)
        n723 = local read "字符布尔"() -> (w1398:bool)
        n724 = case shown="\"R3\"" w1403 {
          tunnel: [38 39] -> w1402
          frame "假", Default {
          }
          frame "R3" {
          }
        }
        n725 = case shown="真" w1398 {
          tunnel: w1404 -> [_ w1407]
          frame False {
          }
          frame True {
            w1405 = "遥控器挂F3档"
            n726 = local write "字符布尔"(FALSE ("字符布尔")) -> ()
            n727 = call "led显示更新字符串山推.vi"("显示字符"=w1405, "立显/保存"=TRUE) -> ("发送数据"=w1409:string)  [unwired: 9 in]
            n728 = local write "LED屏幕信息"(w1405) -> ()
            n729 = call "led发送数据并接收返回山推.vi"("发送数据"=w1409, "TCP网络连接输入"=w1407) -> ()  [unwired: 8 in, 2 out]
          }
        }
        n730 = Enqueue Element(queue=w1401, element=w1402) -> (queue out=w1400:refnum<queue>)  [unwired: 2 in, 2 out]
      }
      frame 39 {
        n731 = local read "R3S"() -> (w1414:dbl)
        n732 = call "已用时间9"("Time Target (s)"=w1414, "Reset"="Reset 9") -> ("Time has Elapsed"=w1418:bool, "Elapsed Time Text"=w1420:string)  [unwired: 10 in, 6 out]
        n733 = call "输出文本.vi"("当前档位"="F3" ("字符串"), "字符串"=w1420) -> ("输出文本"=w1413:string)  [unwired: 9 in]
        n734 = local read "加载左上转速监控"() -> (w1428:dbl)
        n735 = local write "Reset 9"(FALSE ("Reset 9")) -> ()
        n736 = local write "字符布尔"(TRUE ("字符布尔")) -> ()
        n737 = case shown="真" w1418 {
          tunnel: [39 40] -> w1421
          frame False {
          }
          frame True {
            n738 = local write "Reset 9"(TRUE ("Reset 9")) -> ()
          }
        }
        n739 = Build Array (concatenate)(w1425, w1428) -> (w1424:dbl[])
        n740 = call "led显示更新字符串山推.vi"("显示字符"=w1413, "立显/保存"=FALSE) -> ("发送数据"=w1431:string)  [unwired: 9 in]
        n741 = Array Size(array=w1424) -> (size(s)=w1412:i32)
        n742 = Add Array Elements(numeric array=w1424) -> (sum=w1427:dbl)
        n743 = call "led发送数据并接收返回山推.vi"("发送数据"=w1431, "TCP网络连接输入"=w1429) -> ()  [unwired: 8 in, 2 out]
        n744 = local write "LED屏幕信息"(w1413) -> ()
        n745 = Divide(x=w1427, y=w1412) -> (x/y=→"R3平均速度":dbl)
        n746 = Enqueue Element(queue=w1422, element=w1421) -> (queue out=w1423:refnum<queue>)  [unwired: 2 in, 2 out]
      }
      frame 40 {
        n747 = local read "当前试验档位"() -> (w1439:string)
        n748 = local read "字符布尔"() -> (w1435:bool)
        n749 = case shown="\"N\"" w1439 {
          tunnel: [40 41] -> w1436
          frame "假", Default {
          }
          frame "N" {
          }
        }
        n750 = case shown="真" w1435 {
          tunnel: w1440 -> [_ w1444]
          frame False {
          }
          frame True {
            w1442 = "遥控器挂空挡"
            n751 = local write "字符布尔"(FALSE ("字符布尔")) -> ()
            n752 = call "led显示更新字符串山推.vi"("显示字符"=w1442, "立显/保存"=TRUE) -> ("发送数据"=w1446:string)  [unwired: 9 in]
            n753 = local write "LED屏幕信息"(w1442) -> ()
            n754 = call "led发送数据并接收返回山推.vi"("发送数据"=w1446, "TCP网络连接输入"=w1444) -> ()  [unwired: 8 in, 2 out]
          }
        }
        n755 = Enqueue Element(queue=w1438, element=w1436) -> (queue out=w1437:refnum<queue>)  [unwired: 2 in, 2 out]
      }
      frame 41 {
        n756 = local read "遥控器按钮确认"() -> (w1451:bool)
        n757 = local read "字符布尔"() -> (w1449:bool)
        n758 = call <vilib>:"Boolean Crossing PtByPt.vi"("direction"=enum16{"either", "false-true", "true-false"}."false-true", "input"=w1451) -> ("crossing"=w1450:bool)  [unwired: 1 in]
        n759 = case shown="假" w1449 {
          tunnel: w1457 -> [w1460 _]
          frame False {
            w1458 = "车辆挂空挡"
            n760 = local write "字符布尔"(TRUE ("字符布尔")) -> ()
            n761 = call "led显示更新字符串山推.vi"("显示字符"=w1458, "立显/保存"=TRUE) -> ("发送数据"=w1462:string)  [unwired: 9 in]
            n762 = local write "LED屏幕信息"(w1458) -> ()
            n763 = call "led发送数据并接收返回山推.vi"("发送数据"=w1462, "TCP网络连接输入"=w1460) -> ()  [unwired: 8 in, 2 out]
          }
          frame True {
          }
        }
        n764 = case shown="真" w1450 {
          tunnel: [41 42] -> w1453
          frame False {
          }
          frame True {
          }
        }
        n765 = Enqueue Element(queue=w1456, element=w1453) -> (queue out=w1455:refnum<queue>)  [unwired: 2 in, 2 out]
      }
      frame 42 {
        # "由别的线程入队列"
        n766 = local read "字符布尔"() -> (w1465:bool)
        n767 = case shown="真" w1465 {
          tunnel: w1468 -> [_ w1471]
          frame False {
          }
          frame True {
            w1469 = "解开系固系统，浮动油缸，抬起举升，拆除连接，锁紧制动。"
            n768 = local write "字符布尔"(FALSE ("字符布尔")) -> ()
            n769 = local write "LED屏幕信息"(w1469) -> ()
            n770 = call "led显示更新字符串山推.vi"("显示字符"=w1469, "立显/保存"=TRUE) -> ("发送数据"=w1473:string)  [unwired: 9 in]
            n771 = call "led发送数据并接收返回山推.vi"("发送数据"=w1473, "TCP网络连接输入"=w1471) -> ()  [unwired: 8 in, 2 out]
          }
        }
      }
      frame 43 {
        w1474 = "实验完成，请出车"
        n772 = local write "LED屏幕信息"(w1474) -> ()
        n773 = call "led显示更新字符串山推.vi"("显示字符"=w1474, "立显/保存"=TRUE) -> ("发送数据"=w1479:string)  [unwired: 9 in]
        n774 = call "led发送数据并接收返回山推.vi"("发送数据"=w1479, "TCP网络连接输入"=w1477) -> ()  [unwired: 8 in, 2 out]
      }
      frame 44 {
        w1483 = "变频器故障！"
        n775 = local write "LED屏幕信息"(w1483) -> ()
        n776 = Enqueue Element(queue=w1482, element=44 ("元素")) -> (queue out=w1481:refnum<queue>)  [unwired: 2 in, 2 out]
        n777 = call "led显示更新字符串山推.vi"("显示字符"=w1483, "立显/保存"=FALSE) -> ("发送数据"=w1487:string)  [unwired: 9 in]
        n778 = call "led发送数据并接收返回山推.vi"("发送数据"=w1487, "TCP网络连接输入"=w1485) -> ()  [unwired: 8 in, 2 out]
      }
      frame 45 {
        w1493 = "遥控器中断！"
        n779 = local write "LED屏幕信息"(w1493) -> ()
        n780 = Enqueue Element(queue=w1490, element=45 ("元素")) -> (queue out=w1489:refnum<queue>)  [unwired: 2 in, 2 out]
        n781 = call "led显示更新字符串山推.vi"("显示字符"=w1493, "立显/保存"=FALSE) -> ("发送数据"=w1495:string)  [unwired: 9 in]
        n782 = call "led发送数据并接收返回山推.vi"("发送数据"=w1495, "TCP网络连接输入"=w1492) -> ()  [unwired: 8 in, 2 out]
      }
      frame 1, Default {
        n783 = local read "字符布尔"() -> (w1497:bool)
        n784 = case shown="假" w1497 {
          tunnel: w1499 -> [w1502 _]
          frame False {
            w1500 = "选择车型，输入编号，油缸调距。"
            n785 = local write "字符布尔"(TRUE ("字符布尔")) -> ()
            n786 = local write "LED屏幕信息"(w1500) -> ()
            n787 = call "led显示更新字符串山推.vi"("显示字符"=w1500, "立显/保存"=TRUE) -> ("发送数据"=w1504:string)  [unwired: 9 in]
            n788 = call "led发送数据并接收返回山推.vi"("发送数据"=w1504, "TCP网络连接输入"=w1502) -> ()  [unwired: 8 in, 2 out]
          }
          frame True {
          }
        }
      }
    }
    n789 = local read "停止"() -> (w787:bool)
    n790 = Wait (ms)(milliseconds to wait=u32 200 ("等待时间（毫秒）")) -> ()  [unwired: 1 out]
    "数值 3" <- w760
  }
  n791 = stacked-sequence {
    tunnel: w10 -> [_ w1539 _]
    frame #0 {
      w1536 = 0.0 ("D1平均速度")
      n792 = disable-structure shown="禁用" {
        frame Disabled {
          n793 = control-ref of="本VI"() -> (w1537:refnum<vi>)
          n794 = property class="VI"(reference=w1537, "Front Panel.PanelBounds"=T14 {"Left"=0, "Top"=0, "Right"=1280, "Bottom"=1024} ("前面板窗口:前面板边界")) -> ()  [unwired: 1 in, 2 out]
        }
        frame Enabled {
        }
      }
      n795 = call <vilib>:"Application Directory.vi"() -> ("Application Directory"=w1534:path)
      n796 = Build Path(base path=w1534, name or relative path="data\\参数配置.txt" ("名称或相对路径")) -> (appended path=w1532:path)
      n797 = Read from Binary File(5:"簇", 10:1 ("总数(1)"), 11:w1532) -> (2:w1531:T2)  [unwired: 3 in, 3 out]
      n798 = Index Array(array=w1531) -> (element=w1530:T1)  [unwired: 1 in]
      n799 = local write "停止"(FALSE ("停止")) -> ()
      n800 = Unbundle By Name(w1530) -> ("[0]"=w1529:T18, "[1]"=w1519:T18)
      n801 = Unbundle By Name(w1529) -> ("D1"=w1528:dbl, "D2"=w1527:dbl, "D3"=w1526:dbl, "D4"=w1525:dbl, "D5"=w1524:dbl, "D6"=w1523:dbl, "R1"=w1522:dbl, "R2"=w1521:dbl, "R3"=w1520:dbl, "SG14"=w1507:dbl, "SG16-3"=w1506:dbl, "SG18-3"=w1505:dbl)
      n802 = Unbundle By Name(w1519) -> ("D1"=w1518:dbl, "D2"=w1517:dbl, "D3"=w1516:dbl, "D4"=w1515:dbl, "D5"=w1514:dbl, "D6"=w1513:dbl, "R1"=w1512:dbl, "R2"=w1511:dbl, "R3"=w1510:dbl)
      n803 = local write "R1平均速度"(w1536) -> ()
      n804 = local write "R3平均速度"(w1536) -> ()
      n805 = local write "D4平均速度"(w1536) -> ()
      n806 = local write "D5平均速度"(w1536) -> ()
      n807 = local write "D6平均速度"(w1536) -> ()
      n808 = local write "R2平均速度"(w1536) -> ()
      n809 = local write "D3平均速度"(w1536) -> ()
      n810 = local write "D1平均速度"(w1536) -> ()
      n811 = local write "D2平均速度"(w1536) -> ()
      n812 = local write "D1S"(w1518) -> ()
      n813 = local write "D2S"(w1517) -> ()
      n814 = local write "D3S"(w1516) -> ()
      n815 = local write "D4S"(w1515) -> ()
      n816 = local write "D5S"(w1514) -> ()
      n817 = local write "D6S"(w1513) -> ()
      n818 = local write "R1S"(w1512) -> ()
      n819 = local write "R2S"(w1511) -> ()
      n820 = local write "R3S"(w1510) -> ()
      n821 = local write "D1"(w1528) -> ()
      n822 = local write "D2"(w1527) -> ()
      n823 = local write "D3"(w1526) -> ()
      n824 = local write "D4"(w1525) -> ()
      n825 = local write "D5"(w1524) -> ()
      n826 = local write "D6"(w1523) -> ()
      n827 = local write "R1"(w1522) -> ()
      n828 = local write "R2"(w1521) -> ()
      n829 = local write "R3"(w1520) -> ()
      n830 = local write "SG16-3百分比"(w1506) -> ()
      n831 = local write "SG18-3百分比"(w1505) -> ()
      n832 = local write "SG14百分比"(w1507) -> ()
    }
    frame #1 {
      n833 = while {
        shift-right: [w1543] -> _
        shift-left: enum16{"初始化", "事件结构", "退出"}."初始化" -> [w1544]
        tunnel: w1539 -> [w1541]
        stop <- w1542 stop-if-true
        n834 = case shown="\"事件结构\"" w1544 {
          tunnel: [enum16{"初始化", "事件结构", "退出"}."事件结构" w1761 enum16{"初始化", "事件结构", "退出"}."退出"] -> w1543
          tunnel: [FALSE FALSE TRUE] -> w1542
          tunnel: w1541 -> [_ w1757 _]
          frame "初始化", Default {
          }
          frame "事件结构" {
            # "AD25-AD31"
            # "AD17-AD24"
            # "AD9-AD16"
            # "中左在EM9636通道前，此模块为右模块"
            n835 = local read "输出数组左"() -> (w1756:dbl[][])
            n836 = local read "试验车型"() -> (w1758:u16)
            n837 = event shown="[3] \"生成报表\": 值改变" {
              selector: _ -> [_ _ _ _ _ _ _ _ _]
              dyn-events: _ -> [_ _ _ _ _ _ _ _ _]
              timeout: 100 -> [_ _ _ _ _ _ _ _ _]
              tunnel: [enum16{"初始化", "事件结构", "退出"}."事件结构" enum16{"初始化", "事件结构", "退出"}."事件结构" enum16{"初始化", "事件结构", "退出"}."事件结构" enum16{"初始化", "事件结构", "退出"}."事件结构" enum16{"初始化", "事件结构", "退出"}."事件结构" enum16{"初始化", "事件结构", "退出"}."事件结构" enum16{"初始化", "事件结构", "退出"}."事件结构" enum16{"初始化", "事件结构", "退出"}."事件结构" enum16{"初始化", "事件结构", "退出"}."退出"] -> w1761
              tunnel: w1757 -> [_ w1879 w1895 _ w1995 _ _ w2166 _]
              event Timeout {
                n838 = event-data() -> ()  [unwired: 1 in, 3 out]
                n839 = Format Date/Time String(time format string (%c)="%Y年%m月%d日 %H:%M:%S" ("时间格式字符串(%c)")) -> (date/time string=→"系统时间 2":string)  [unwired: 2 in]
              }
              event "确认输入": Value Change {
                # "D1档速度"
                n840 = event-data() -> ()  [unwired: 1 in, 6 out]
                n841 = Flush Queue(queue=w1879) -> (queue out=w1878:refnum<queue>)  [unwired: 1 in, 2 out]
                n842 = Enqueue Element(queue=w1878, element=2 ("元素")) -> ()  [unwired: 2 in, 3 out]
                n843 = case shown="3" "试验车型" {
                  tunnel: ["SG21-3" "SG14" "SG16-3" "SG18-3"] -> w1887
                  frame 0, Default {
                  }
                  frame 1 {
                  }
                  frame 2 {
                  }
                  frame 3 {
                  }
                }
                "车型" <- w1887
                n844 = local write "等待进车布尔"(TRUE ("等待进车布尔")) -> ()
                n845 = Build Array(w1887, "试验车编号", "发动机编号", "操作者") -> (w1882:string[])
                "中间数组" <- w1882
                n846 = Build Array (concatenate)(string[][] [], w1882) -> (→"实验基本信息":string[][])
              }
              event "试验开始": Value Change {
                n847 = event-data() -> ("NewVal"=w1896:bool)  [unwired: 1 in, 5 out]
                n848 = case shown="真" w1896 {
                  tunnel: w1895 -> [w1898 w1914]
                  frame False {
                    n849 = Flush Queue(queue=w1898) -> (queue out=w1897:refnum<queue>)  [unwired: 1 in, 2 out]
                    n850 = Enqueue Element(queue=w1897, element=43 ("元素")) -> ()  [unwired: 2 in, 3 out]
                    n851 = property on="加载电机右上启动" class="Bool (严格)"("Val(Sgnl)"=FALSE ("值(信号)")) -> ()  [unwired: 2 in, 2 out]
                    n852 = property on="加载电机左上启动" class="Bool (严格)"("Val(Sgnl)"=FALSE ("值(信号)")) -> ()  [unwired: 2 in, 2 out]
                    n853 = property on="加载电机左下启动" class="Bool (严格)"("Val(Sgnl)"=FALSE ("值(信号)")) -> ()  [unwired: 2 in, 2 out]
                    n854 = property on="驱动电机下启动" class="Bool (严格)"("Val(Sgnl)"=FALSE ("值(信号)")) -> ()  [unwired: 2 in, 2 out]
                    n855 = property on="加载电机右下启动" class="Bool (严格)"("Val(Sgnl)"=FALSE ("值(信号)")) -> ()  [unwired: 2 in, 2 out]
                    n856 = property on="驱动电机上启动" class="Bool (严格)"("Val(Sgnl)"=FALSE ("值(信号)")) -> ()  [unwired: 2 in, 2 out]
                  }
                  frame True {
                    w1906 = TRUE
                    n857 = Flush Queue(queue=w1914) -> (queue out=w1913:refnum<queue>)  [unwired: 1 in, 2 out]
                    n858 = Enqueue Element(queue=w1913, element=1 ("元素")) -> ()  [unwired: 2 in, 3 out]
                    n859 = local write "变频6"(w1906) -> ()
                    n860 = local write "变频5"(w1906) -> ()
                    n861 = local write "变频4"(w1906) -> ()
                    n862 = local write "字符布尔"(FALSE ("字符布尔")) -> ()
                    n863 = local write "变频3"(w1906) -> ()
                    n864 = local write "变频2"(w1906) -> ()
                    n865 = local write "变频1"(w1906) -> ()
                    n866 = property on="加载电机右上启动" class="Bool (严格)"("Val(Sgnl)"=TRUE ("值(信号)")) -> ()  [unwired: 2 in, 2 out]
                    n867 = property on="加载电机左上启动" class="Bool (严格)"("Val(Sgnl)"=TRUE ("值(信号)")) -> ()  [unwired: 2 in, 2 out]
                    n868 = property on="加载电机左下启动" class="Bool (严格)"("Val(Sgnl)"=TRUE ("值(信号)")) -> ()  [unwired: 2 in, 2 out]
                    n869 = property on="驱动电机下启动" class="Bool (严格)"("Val(Sgnl)"=TRUE ("值(信号)")) -> ()  [unwired: 2 in, 2 out]
                    n870 = property on="加载电机右下启动" class="Bool (严格)"("Val(Sgnl)"=TRUE ("值(信号)")) -> ()  [unwired: 2 in, 2 out]
                    n871 = property on="驱动电机上启动" class="Bool (严格)"("Val(Sgnl)"=TRUE ("值(信号)")) -> ()  [unwired: 2 in, 2 out]
                  }
                }
              }
              event "生成报表": Value Change {
                n872 = event-data() -> ()  [unwired: 1 in, 6 out]
                n873 = flat-sequence {
                  frame #0 {
                    w1922 = u16 2 items=["US", "公制", "默认"] ("measurement system")
                    w1923 = u16 2 items=["US", "公制", "默认"] ("measurement system")
                    w1924 = u16 2 items=["US", "公制", "默认"] ("measurement system")
                    w1926 = -1.0 ("column width (1)")
                    n874 = local read "实验基本信息"() -> (w1980:string[][])
                    n875 = local read "R1平均速度"() -> (w1949:dbl)
                    n876 = local read "R3平均速度"() -> (w1947:dbl)
                    n877 = local read "D4平均速度"() -> (w1952:dbl)
                    n878 = local read "D5平均速度"() -> (w1951:dbl)
                    n879 = local read "D6平均速度"() -> (w1950:dbl)
                    n880 = local read "R2平均速度"() -> (w1948:dbl)
                    n881 = local read "D3平均速度"() -> (w1953:dbl)
                    n882 = local read "D1平均速度"() -> (w1955:dbl)
                    n883 = local read "D2平均速度"() -> (w1954:dbl)
                    n884 = local read "系统时间 2"() -> (w1930:string)
                    n885 = call <vilib>:"New Report.vi"("report type"=T16."Excel", "template (empty)"=path "E:/模板/输出数据表格.xlsx") -> ("report out"=w1981:refnum<class "NI_report.lvclass">, "error out"=w1962:errorcluster)  [unwired: 12 in]
                    n886 = Build Array(w1955, w1954, w1953, w1952, w1951, w1950, w1949, w1948, w1947) -> (w1946:dbl[])
                    n887 = call-poly <vilib>:"Append Table to Report.vi"("report in"=w1981, "column width (1)"=w1926, "measurement system"=w1923, "MS Office parameters"=T15 {"position (excel)"={"row"=5, "column"=2}, "name (excel)"="", "bookmark (word)"=""}, "text data"=w1980, "error in (no error)"=w1962) -> ("report out"=w1934:refnum<class "NI_report.lvclass">, "error out"=w1935:errorcluster)  [unwired: 6 in, 2 out]
                    n888 = for {
                      tunnel: w1946 -> [w1987] mode=indexing
                      tunnel: [w1988] -> w1945 mode=indexing
                      n889 = Multiply(x=w1987, y=-1.0) -> (x*y=w1984:dbl)
                      n890 = Absolute Value(x=w1984) -> (abs(x)=w1985:dbl)
                      n891 = call "speed.vi"("rmp"=w1985) -> ("km/h"=w1988:dbl)  [unwired: 10 in]
                    }
                    n892 = Initialize Array(w1930, 1 ("维数大小"), 1 ("维数大小")) -> (w1927:string[][])
                    n893 = call-poly <vilib>:"Append Table to Report.vi"("report in"=w1934, "column width (1)"=w1926, "measurement system"=w1924, "MS Office parameters"=T15 {"position (excel)"={"row"=3, "column"=3}, "name (excel)"="", "bookmark (word)"=""}, "text data"=w1927, "error in (no error)"=w1935) -> ("report out"=w1933:refnum<class "NI_report.lvclass">, "error out"=w1932:errorcluster)  [unwired: 6 in, 2 out]
                    n894 = local read "环境温度标定"() -> (w1970:dbl)
                    n895 = local read "液压油箱温度标定"() -> (w1971:dbl)
                    n896 = local read "变矩器出口温度标定"() -> (w1972:dbl)
                    n897 = local read "左前轮轴承温度标定"() -> (w1973:dbl)
                    n898 = local read "右前轮轴承温度标定"() -> (w1974:dbl)
                    n899 = local read "振动泵压力"() -> (w1975:dbl)
                    n900 = local read "转向泵压力"() -> (w1976:dbl)
                    n901 = Index Array(array=w1945) -> (element #1=w1944:dbl, element #2=w1943:dbl, element #3=w1942:dbl, element #4=w1941:dbl, element #5=w1940:dbl, element #6=w1939:dbl, element #7=w1938:dbl, element #8=w1937:dbl, element #9=w1936:dbl)  [unwired: 9 in]
                    n902 = Build Array(w1970, w1971, w1972, w1973, w1974, w1975, w1976, w1944, w1943, w1942, w1941, w1940, w1939, w1938, w1937, w1936) -> (w1977:dbl[])
                    n903 = for {
                      tunnel: w1977 -> [w1990] mode=indexing
                      tunnel: [w1989] -> w1978 mode=indexing
                      n904 = Number To Fractional String(number=w1990, precision (6)=i16 2 ("宽度(-)")) -> (F-format string=w1989:string)  [unwired: 2 in]
                    }
                    n905 = Build Array (concatenate)("速度温度", w1978) -> (w1968:string[][])
                    n906 = local read "试验车编号"() -> (w1920:string)
                    n907 = Transpose 2D Array(2D array=w1968) -> (transposed array=w1967:string[][])
                    n908 = local read "车型"() -> (w1921:string)
                    n909 = call-poly <vilib>:"Append Table to Report.vi"("report in"=w1933, "column width (1)"=-1.0, "measurement system"=w1922, "MS Office parameters"=T15 {"position (excel)"={"row"=7, "column"=5}, "name (excel)"="", "bookmark (word)"=""}, "text data"=w1967, "error in (no error)"=w1932) -> ("report out"=w1965:refnum<class "NI_report.lvclass">, "error out"=w1960:errorcluster)  [unwired: 6 in, 2 out]
                    n910 = Concatenate Strings(w1921, "_" ("字符串"), w1920) -> (w1919:string)
                    n911 = Build Path(base path=path "E:/数据保存" ("基路径"), name or relative path=w1919) -> (appended path=w1957:path)
                    n912 = call-dynamic "Save Report to File.vi"("report in"=w1965, "report file path"=w1957, "prompt to replace? (F)"=FALSE, "error in (no error)"=w1960) -> ("report out"=w1964:refnum<class "NI_report.lvclass">, "error out"=w1959:errorcluster)  [unwired: 10 in]
                    n913 = call-dynamic "Dispose Report.vi"("report in"=w1964, "wait until printing completed? (T)"=TRUE, "error in (no error)"=w1959) -> ("error out"=w1956:errorcluster)  [unwired: 12 in]
                    n914 = call <vilib>:"Clear Errors.vi"("error in (no error)"=w1956) -> ()  [unwired: 5 in, 2 out]
                  }
                  frame #1 {
                    w1992 = string[][] []
                    n915 = local write "实验基本信息"(w1992) -> ()
                    n916 = local write "速度温度"(w1992) -> ()
                  }
                }
              }
              event "重新实验": Value Change {
                n917 = event-data() -> ()  [unwired: 1 in, 6 out]
                n918 = Flush Queue(queue=w1995) -> (queue out=w1994:refnum<queue>)  [unwired: 1 in, 2 out]
                n919 = Enqueue Element(queue=w1994, element=2 ("元素")) -> ()  [unwired: 2 in, 3 out]
                n920 = local write "速度温度"(string[][] []) -> ()
                "等待进车布尔" <- TRUE ("重新实验布尔")
              }
              event "高级参数": Value Change {
                n921 = event-data() -> ()  [unwired: 1 in, 6 out]
                n922 = property class="App"() -> ("App.Kind"=w2011:T19)  [unwired: 2 in, 2 out]
                n923 = case shown="\"Run Time System\"" w2011 {
                  tunnel: ["授权文件\\登录界面.vi" ("名称或相对路径") "..\\授权文件\\登录界面.vi" ("名称或相对路径")] -> w2012
                  tunnel: [w2014 w2017] -> w2013
                  frame "Development System", Default {
                    n924 = call <vilib>:"Application Directory.vi"() -> ("Application Directory"=w2014:path)
                  }
                  frame "Run Time System" {
                    n925 = Current VI's Path() -> (path=w2017:path)
                  }
                }
                n926 = Build Path(base path=w2013, name or relative path=w2012) -> (appended path=w2000:path)
                n927 = Open VI Reference(vi path=w2000) -> (vi reference=w2004:refnum<vi>, error out=w2007:errorcluster)  [unwired: 5 in]
                n928 = invoke class="VI" method="FP.Open"(reference=w2004, error in=w2007, "Activate"=TRUE ("激活？"), "State"=T17."Standard" ("状态")) -> (reference out=w2001:refnum<vi>, error out=w2008:errorcluster)  [unwired: 1 in, 3 out]
                n929 = invoke class="VI" method="Run VI"(reference=w2001, error in=w2008, "Wait until done"=FALSE ("结束前等待")) -> (reference out=w2003:refnum<vi>, error out=w2009:errorcluster)  [unwired: 2 in, 3 out]
                n930 = Close Reference(reference=w2003, error in (no error)=w2009) -> (error out=→"错误输出 7":errorcluster)
              }
              event "刷新参数": Value Change {
                n931 = event-data() -> ()  [unwired: 1 in, 6 out]
                n932 = call <vilib>:"Application Directory.vi"() -> ("Application Directory"=w2060:path)
                n933 = Build Path(base path=w2060, name or relative path="data\\参数配置.txt" ("名称或相对路径")) -> (appended path=w2058:path)
                n934 = Read from Binary File(5:"簇 3", 10:1 ("总数(1)"), 11:w2058) -> (2:w2055:T2)  [unwired: 3 in, 3 out]
                "数据" <- w2055
                n935 = Index Array(array=w2055) -> (element=w2057:T1)  [unwired: 1 in]
                n936 = Unbundle By Name(w2057) -> ("[0]"=w2056:T18, "[1]"=w2031:T18, "[2]"=w2030:T18, "[3]"=w2029:T18, "[4]"=w2028:T18)
                n937 = Unbundle By Name(w2056) -> ("D1"=w2053:dbl, "D2"=w2052:dbl, "D3"=w2051:dbl, "D4"=w2050:dbl, "D5"=w2049:dbl, "D6"=w2048:dbl, "R1"=w2047:dbl, "R2"=w2046:dbl, "R3"=w2045:dbl, "SG14"=w2044:dbl, "SG16-3"=w2043:dbl, "SG18-3"=w2042:dbl)
                "D3" <- w2051
                "D4" <- w2050
                "D5" <- w2049
                "D6" <- w2048
                "R1" <- w2047
                "R2" <- w2046
                "R3" <- w2045
                "D2" <- w2052
                "D1" <- w2053
                "SG14百分比" <- w2044
                "SG16-3百分比" <- w2043
                "SG18-3百分比" <- w2042
                n938 = local read "试验车型"() -> (w2054:u16)
                n939 = case shown="3" w2054 {
                  tunnel: w2053 -> [w2083 w2108 w2133 w2158]
                  tunnel: w2052 -> [w2082 w2107 w2132 w2157]
                  tunnel: w2051 -> [w2081 w2106 w2131 w2156]
                  tunnel: w2050 -> [w2080 w2105 w2130 w2155]
                  tunnel: w2049 -> [w2079 w2104 w2129 w2154]
                  tunnel: w2048 -> [w2078 w2103 w2128 w2153]
                  tunnel: w2047 -> [w2077 w2102 w2127 w2152]
                  tunnel: w2046 -> [w2076 w2101 w2126 w2151]
                  tunnel: w2045 -> [w2075 w2100 w2125 w2150]
                  tunnel: w2044 -> [_ w2098 _ _]
                  tunnel: w2043 -> [_ _ w2123 _]
                  tunnel: w2042 -> [_ _ _ w2148]
                  tunnel: [w2072 w2096 w2121 w2146] -> w2041
                  tunnel: [w2071 w2095 w2120 w2145] -> w2040
                  tunnel: [w2070 w2094 w2119 w2144] -> w2039
                  tunnel: [w2069 w2093 w2118 w2143] -> w2038
                  tunnel: [w2068 w2092 w2117 w2142] -> w2037
                  tunnel: [w2067 w2091 w2116 w2141] -> w2036
                  tunnel: [w2066 w2090 w2115 w2140] -> w2035
                  tunnel: [w2065 w2089 w2114 w2139] -> w2034
                  tunnel: [w2064 w2088 w2113 w2138] -> w2033
                  tunnel: w2031 -> [w2063 _ _ _]
                  tunnel: w2030 -> [_ w2087 _ _]
                  tunnel: w2029 -> [_ _ w2112 _]
                  tunnel: w2028 -> [_ _ _ w2137]
                  tunnel: [w2063 w2087 w2112 w2137] -> w2027
                  frame 0, Default {
                    n940 = Build Array(w2083, w2082, w2081, w2080, w2079, w2078, w2077, w2076, w2075) -> (w2074:dbl[])
                    n941 = for {
                      tunnel: w2074 -> [w2086] mode=indexing
                      tunnel: [w2084] -> w2073 mode=indexing
                      n942 = call "实验车型选择比例 (子VI).vi"("SG14百分比"=100.0, "D1"=w2086) -> ("数值"=w2084:dbl)  [unwired: 9 in]
                    }
                    n943 = Index Array(array=w2073) -> (element #1=w2072:dbl, element #2=w2071:dbl, element #3=w2070:dbl, element #4=w2069:dbl, element #5=w2068:dbl, element #6=w2067:dbl, element #7=w2066:dbl, element #8=w2065:dbl, element #9=w2064:dbl)  [unwired: 9 in]
                  }
                  frame 1 {
                    n944 = Build Array(w2108, w2107, w2106, w2105, w2104, w2103, w2102, w2101, w2100) -> (w2099:dbl[])
                    n945 = for {
                      tunnel: w2099 -> [w2111] mode=indexing
                      tunnel: w2098 -> [w2110]
                      tunnel: [w2109] -> w2097 mode=indexing
                      n946 = call "实验车型选择比例 (子VI).vi"("SG14百分比"=w2110, "D1"=w2111) -> ("数值"=w2109:dbl)  [unwired: 9 in]
                    }
                    n947 = Index Array(array=w2097) -> (element #1=w2096:dbl, element #2=w2095:dbl, element #3=w2094:dbl, element #4=w2093:dbl, element #5=w2092:dbl, element #6=w2091:dbl, element #7=w2090:dbl, element #8=w2089:dbl, element #9=w2088:dbl)  [unwired: 9 in]
                  }
                  frame 2 {
                    n948 = Build Array(w2133, w2132, w2131, w2130, w2129, w2128, w2127, w2126, w2125) -> (w2124:dbl[])
                    n949 = for {
                      tunnel: w2124 -> [w2136] mode=indexing
                      tunnel: w2123 -> [w2135]
                      tunnel: [w2134] -> w2122 mode=indexing
                      n950 = call "实验车型选择比例 (子VI).vi"("SG14百分比"=w2135, "D1"=w2136) -> ("数值"=w2134:dbl)  [unwired: 9 in]
                    }
                    n951 = Index Array(array=w2122) -> (element #1=w2121:dbl, element #2=w2120:dbl, element #3=w2119:dbl, element #4=w2118:dbl, element #5=w2117:dbl, element #6=w2116:dbl, element #7=w2115:dbl, element #8=w2114:dbl, element #9=w2113:dbl)  [unwired: 9 in]
                  }
                  frame 3 {
                    n952 = Build Array(w2158, w2157, w2156, w2155, w2154, w2153, w2152, w2151, w2150) -> (w2149:dbl[])
                    n953 = for {
                      tunnel: w2149 -> [w2161] mode=indexing
                      tunnel: w2148 -> [w2160]
                      tunnel: [w2159] -> w2147 mode=indexing
                      n954 = call "实验车型选择比例 (子VI).vi"("SG14百分比"=w2160, "D1"=w2161) -> ("数值"=w2159:dbl)  [unwired: 9 in]
                    }
                    n955 = Index Array(array=w2147) -> (element #1=w2146:dbl, element #2=w2145:dbl, element #3=w2144:dbl, element #4=w2143:dbl, element #5=w2142:dbl, element #6=w2141:dbl, element #7=w2140:dbl, element #8=w2139:dbl, element #9=w2138:dbl)  [unwired: 9 in]
                  }
                }
                "D3 act" <- w2039
                "D4 act" <- w2038
                "D5 act" <- w2037
                "D6 act" <- w2036
                "R1 act" <- w2035
                "R2 act" <- w2034
                "R3 act" <- w2033
                "D2 act" <- w2040
                "D1 act" <- w2041
                n956 = Unbundle By Name(w2027) -> ("D1"=→"D1S":dbl, "D2"=→"D2S":dbl, "D3"=→"D3S":dbl, "D4"=→"D4S":dbl, "D5"=→"D5S":dbl, "D6"=→"D6S":dbl, "R1"=→"R1S":dbl, "R2"=→"R2S":dbl, "R3"=→"R3S":dbl)
              }
              event "确认换挡": Value Change {
                w2162 = TRUE ("Reset")
                w2164 = TRUE
                n957 = event-data() -> ()  [unwired: 1 in, 6 out]
                n958 = Flush Queue(queue=w2166) -> (queue out=w2165:refnum<queue>)  [unwired: 1 in, 2 out]
                n959 = case shown="\"D2\"" "重新选档档位" {
                  tunnel: w2165 -> [w2171 w2174 w2177 w2180 w2183 w2186 w2189 w2192 w2195]
                  frame "D1", Default {
                    n960 = Enqueue Element(queue=w2171, element=4 ("元素")) -> ()  [unwired: 2 in, 3 out]
                    n961 = local write "字符布尔"(FALSE ("字符布尔")) -> ()
                  }
                  frame "D2" {
                    n962 = local write "字符布尔"(FALSE ("字符布尔")) -> ()
                    n963 = Enqueue Element(queue=w2174, element=8 ("元素")) -> ()  [unwired: 2 in, 3 out]
                  }
                  frame "D3" {
                    n964 = local write "字符布尔"(FALSE ("字符布尔")) -> ()
                    n965 = Enqueue Element(queue=w2177, element=12 ("元素")) -> ()  [unwired: 2 in, 3 out]
                  }
                  frame "D4" {
                    n966 = local write "字符布尔"(FALSE ("字符布尔")) -> ()
                    n967 = Enqueue Element(queue=w2180, element=16 ("元素")) -> ()  [unwired: 2 in, 3 out]
                  }
                  frame "D5" {
                    n968 = Enqueue Element(queue=w2183, element=20 ("元素")) -> ()  [unwired: 2 in, 3 out]
                    n969 = local write "字符布尔"(FALSE ("字符布尔")) -> ()
                  }
                  frame "D6" {
                    n970 = Enqueue Element(queue=w2186, element=24 ("元素")) -> ()  [unwired: 2 in, 3 out]
                    n971 = local write "字符布尔"(FALSE ("字符布尔")) -> ()
                  }
                  frame "R1" {
                    n972 = local write "字符布尔"(TRUE ("字符布尔")) -> ()
                    n973 = Enqueue Element(queue=w2189, element=29 ("元素")) -> ()  [unwired: 2 in, 3 out]
                  }
                  frame "R2" {
                    n974 = local write "字符布尔"(FALSE ("字符布尔")) -> ()
                    n975 = Enqueue Element(queue=w2192, element=33 ("元素")) -> ()  [unwired: 2 in, 3 out]
                  }
                  frame "R3" {
                    n976 = local write "字符布尔"(FALSE ("字符布尔")) -> ()
                    n977 = Enqueue Element(queue=w2195, element=37 ("元素")) -> ()  [unwired: 2 in, 3 out]
                  }
                }
                n978 = local write "Reset 7"(w2162) -> ()
                n979 = local write "Reset 9"(w2162) -> ()
                n980 = local write "Reset 8"(w2162) -> ()
                n981 = local write "Reset"(w2162) -> ()
                n982 = local write "Reset 2"(w2162) -> ()
                n983 = local write "Reset 3"(w2162) -> ()
                n984 = local write "Reset 4"(w2162) -> ()
                n985 = local write "Reset 5"(w2162) -> ()
                n986 = local write "Reset 6"(w2162) -> ()
                n987 = local write "变频6"(w2164) -> ()
                n988 = local write "变频5"(w2164) -> ()
                n989 = local write "变频4"(w2164) -> ()
                n990 = local write "变频3"(w2164) -> ()
                n991 = local write "变频2"(w2164) -> ()
                n992 = local write "变频1"(w2164) -> ()
                n993 = local write "comcnt"(u16 0 ("comcnt")) -> ()
              }
              event "停止": Value Change {
                n994 = event-data() -> ()  [unwired: 1 in, 6 out]
              }
            }
            n995 = Index Array(array=w1756) -> (element #1=w1754:dbl[], element #2=w1743:dbl[], element #3=w1734:dbl[], element #4=w1724:dbl[])  [unwired: 8 in]
            n996 = case shown="1" w1758 {
              frame 0, Default {
                n997 = local read "D1"() -> (w1798:dbl)
                n998 = local read "D2"() -> (w1797:dbl)
                n999 = local read "D3"() -> (w1796:dbl)
                n1000 = local read "D4"() -> (w1795:dbl)
                n1001 = local read "D5"() -> (w1794:dbl)
                n1002 = local read "D6"() -> (w1793:dbl)
                n1003 = local read "R1"() -> (w1792:dbl)
                n1004 = local read "R2"() -> (w1791:dbl)
                n1005 = local read "R3"() -> (w1790:dbl)
                n1006 = Build Array(w1798, w1797, w1796, w1795, w1794, w1793, w1792, w1791, w1790) -> (w1789:dbl[])
                n1007 = for {
                  tunnel: w1789 -> [w1801] mode=indexing
                  tunnel: [w1800] -> w1788 mode=indexing
                  tunnel: 100.0 -> [w1799]
                  n1008 = call "档位加载比例 (子VI).vi"("更换车型加载比例"=w1799, "D1-D3/R1/R2加载比例"=w1801) -> ("数值"=w1800:dbl)  [unwired: 9 in]
                }
                n1009 = Index Array(array=w1788) -> (element #1=w1787:dbl, element #2=w1786:dbl, element #3=w1785:dbl, element #4=w1784:dbl, element #5=w1783:dbl, element #6=w1782:dbl, element #7=w1781:dbl, element #8=w1780:dbl, element #9=w1779:dbl)  [unwired: 9 in]
                n1010 = local write "D1扭矩给定"(w1787) -> ()
                n1011 = local write "D2扭矩给定"(w1786) -> ()
                n1012 = local write "D3扭矩给定"(w1785) -> ()
                n1013 = local write "D4扭矩给定"(w1784) -> ()
                n1014 = local write "D5扭矩给定"(w1783) -> ()
                n1015 = local write "D6扭矩给定"(w1782) -> ()
                n1016 = local write "R1扭矩给定"(w1781) -> ()
                n1017 = local write "R2扭矩给定"(w1780) -> ()
                n1018 = local write "R3扭矩给定"(w1779) -> ()
              }
              frame 1 {
                n1019 = local read "D1"() -> (w1820:dbl)
                n1020 = local read "D2"() -> (w1819:dbl)
                n1021 = local read "D3"() -> (w1818:dbl)
                n1022 = local read "D4"() -> (w1817:dbl)
                n1023 = local read "D5"() -> (w1816:dbl)
                n1024 = local read "D6"() -> (w1815:dbl)
                n1025 = local read "R1"() -> (w1814:dbl)
                n1026 = local read "R2"() -> (w1813:dbl)
                n1027 = local read "R3"() -> (w1812:dbl)
                n1028 = local read "SG14百分比"() -> (w1802:dbl)
                n1029 = Build Array(w1820, w1819, w1818, w1817, w1816, w1815, w1814, w1813, w1812) -> (w1822:dbl[])
                n1030 = for {
                  tunnel: w1822 -> [w1824] mode=indexing
                  tunnel: [w1825] -> w1821 mode=indexing
                  tunnel: w1802 -> [w1823]
                  n1031 = call "档位加载比例 (子VI).vi"("更换车型加载比例"=w1823, "D1-D3/R1/R2加载比例"=w1824) -> ("数值"=w1825:dbl)  [unwired: 9 in]
                }
                n1032 = Index Array(array=w1821) -> (element #1=w1811:dbl, element #2=w1810:dbl, element #3=w1809:dbl, element #4=w1808:dbl, element #5=w1807:dbl, element #6=w1806:dbl, element #7=w1805:dbl, element #8=w1804:dbl, element #9=w1803:dbl)  [unwired: 9 in]
                n1033 = local write "D2扭矩给定"(w1810) -> ()
                n1034 = local write "D3扭矩给定"(w1809) -> ()
                n1035 = local write "D4扭矩给定"(w1808) -> ()
                n1036 = local write "D1扭矩给定"(w1811) -> ()
                n1037 = local write "D5扭矩给定"(w1807) -> ()
                n1038 = local write "D6扭矩给定"(w1806) -> ()
                n1039 = local write "R1扭矩给定"(w1805) -> ()
                n1040 = local write "R2扭矩给定"(w1804) -> ()
                n1041 = local write "R3扭矩给定"(w1803) -> ()
              }
              frame 2 {
                n1042 = local read "D1"() -> (w1844:dbl)
                n1043 = local read "D2"() -> (w1843:dbl)
                n1044 = local read "D3"() -> (w1842:dbl)
                n1045 = local read "D4"() -> (w1841:dbl)
                n1046 = local read "D5"() -> (w1840:dbl)
                n1047 = local read "D6"() -> (w1839:dbl)
                n1048 = local read "R1"() -> (w1838:dbl)
                n1049 = local read "R2"() -> (w1837:dbl)
                n1050 = local read "R3"() -> (w1836:dbl)
                n1051 = local read "SG16-3百分比"() -> (w1826:dbl)
                n1052 = Build Array(w1844, w1843, w1842, w1841, w1840, w1839, w1838, w1837, w1836) -> (w1846:dbl[])
                n1053 = for {
                  tunnel: w1846 -> [w1848] mode=indexing
                  tunnel: [w1849] -> w1845 mode=indexing
                  tunnel: w1826 -> [w1847]
                  n1054 = call "档位加载比例 (子VI).vi"("更换车型加载比例"=w1847, "D1-D3/R1/R2加载比例"=w1848) -> ("数值"=w1849:dbl)  [unwired: 9 in]
                }
                n1055 = Index Array(array=w1845) -> (element #1=w1835:dbl, element #2=w1834:dbl, element #3=w1833:dbl, element #4=w1832:dbl, element #5=w1831:dbl, element #6=w1830:dbl, element #7=w1829:dbl, element #8=w1828:dbl, element #9=w1827:dbl)  [unwired: 9 in]
                n1056 = local write "D2扭矩给定"(w1834) -> ()
                n1057 = local write "D3扭矩给定"(w1833) -> ()
                n1058 = local write "R1扭矩给定"(w1829) -> ()
                n1059 = local write "R2扭矩给定"(w1828) -> ()
                n1060 = local write "D1扭矩给定"(w1835) -> ()
                n1061 = local write "R3扭矩给定"(w1827) -> ()
                n1062 = local write "D4扭矩给定"(w1832) -> ()
                n1063 = local write "D5扭矩给定"(w1831) -> ()
                n1064 = local write "D6扭矩给定"(w1830) -> ()
              }
              frame 3 {
                n1065 = local read "D1"() -> (w1868:dbl)
                n1066 = local read "D2"() -> (w1867:dbl)
                n1067 = local read "D3"() -> (w1866:dbl)
                n1068 = local read "D4"() -> (w1865:dbl)
                n1069 = local read "D5"() -> (w1864:dbl)
                n1070 = local read "D6"() -> (w1863:dbl)
                n1071 = local read "R1"() -> (w1862:dbl)
                n1072 = local read "R2"() -> (w1861:dbl)
                n1073 = local read "R3"() -> (w1860:dbl)
                n1074 = local read "SG18-3百分比"() -> (w1850:dbl)
                n1075 = Build Array(w1868, w1867, w1866, w1865, w1864, w1863, w1862, w1861, w1860) -> (w1870:dbl[])
                n1076 = for {
                  tunnel: w1870 -> [w1872] mode=indexing
                  tunnel: [w1873] -> w1869 mode=indexing
                  tunnel: w1850 -> [w1871]
                  n1077 = call "档位加载比例 (子VI).vi"("更换车型加载比例"=w1871, "D1-D3/R1/R2加载比例"=w1872) -> ("数值"=w1873:dbl)  [unwired: 9 in]
                }
                n1078 = Index Array(array=w1869) -> (element #1=w1859:dbl, element #2=w1858:dbl, element #3=w1857:dbl, element #4=w1856:dbl, element #5=w1855:dbl, element #6=w1854:dbl, element #7=w1853:dbl, element #8=w1852:dbl, element #9=w1851:dbl)  [unwired: 9 in]
                n1079 = local write "D4扭矩给定"(w1856) -> ()
                n1080 = local write "D5扭矩给定"(w1855) -> ()
                n1081 = local write "D6扭矩给定"(w1854) -> ()
                n1082 = local write "R1扭矩给定"(w1853) -> ()
                n1083 = local write "R2扭矩给定"(w1852) -> ()
                n1084 = local write "D2扭矩给定"(w1858) -> ()
                n1085 = local write "D3扭矩给定"(w1857) -> ()
                n1086 = local write "R3扭矩给定"(w1851) -> ()
                n1087 = local write "D1扭矩给定"(w1859) -> ()
              }
            }
            n1088 = for {
              N: 8 -> [_]
              tunnel: w1754 -> [w1777] mode=indexing
              tunnel: [w1776] -> w1753 mode=indexing
              n1089 = call "温度标定.vi"("输入电压"=w1777) -> ("输出温度"=w1776:dbl)  [unwired: 10 in]
            }
            n1090 = Index Array(array=w1753) -> (element #1=→"前左滚筒左轴承":dbl, element #2=→"前左滚筒右轴承":dbl, element #3=→"前左电机左轴承":dbl, element #4=→"前左电机右轴承":dbl, element #5=→"前左电机绕组" →"前左":dbl, element #6=→"前右滚筒左轴承":dbl, element #7=→"前左滚筒右轴承":dbl, element #8=→"前右滚筒左轴承":dbl)  [unwired: 8 in]
            n1091 = for {
              N: 8 -> [_]
              tunnel: w1743 -> [w1775] mode=indexing
              tunnel: [w1774] -> w1745 mode=indexing
              n1092 = call "温度标定.vi"("输入电压"=w1775) -> ("输出温度"=w1774:dbl)  [unwired: 10 in]
            }
            n1093 = Index Array(array=w1745) -> (element #1=→"前右电机右轴承":dbl, element #2=→"前右电机绕组" →"前右":dbl, element #3=→"中左滚筒左轴承":dbl, element #4=→"中左滚筒右轴承":dbl, element #5=→"中左电机左轴承":dbl, element #6=→"中左电机右轴承":dbl, element #7=→"中左电机绕组" →"中左":dbl, element #8=→"中右滚筒左轴承":dbl)  [unwired: 8 in]
            n1094 = local read "输出数组右"() -> (w1719:dbl[][])
            n1095 = Index Array(array=w1719) -> (element #1=w1718:dbl[], element #2=w1680:dbl[], element #3=w1705:dbl[], element #4=w1692:dbl[])  [unwired: 8 in]
            n1096 = for {
              N: 8 -> [_]
              tunnel: w1734 -> [w1773] mode=indexing
              tunnel: [w1772] -> w1735 mode=indexing
              n1097 = call "温度标定.vi"("输入电压"=w1773) -> ("输出温度"=w1772:dbl)  [unwired: 10 in]
            }
            n1098 = Index Array(array=w1718) -> (element #1=w1717:dbl, element #2=w1716:dbl, element #3=w1714:dbl, element #4=w1713:dbl, element #5=w1712:dbl, element #6=w1711:dbl, element #7=w1710:dbl, element #8=w1709:dbl)  [unwired: 8 in]
            n1099 = Build Array(w1714, w1713, w1712, w1711, w1710, w1709) -> (w1671:dbl[])
            n1100 = Index Array(array=w1671, index=2 ("索引")) -> (element=w1668:dbl)
            n1101 = call "泵压力标定.vi"("振动泵信号输入"=w1717) -> ("振动泵压力输出"=w1704:dbl)  [unwired: 10 in]
            n1102 = Subtract(x=w1668, y=0.0) -> (x-y=→"中左电机左轴承振动":dbl)
            n1103 = for {
              N: 6 -> [_]
              tunnel: w1671 -> [w1769] mode=indexing
              tunnel: [w1769] -> w1708 mode=indexing
            }
            n1104 = Index Array(array=w1735) -> (element #1=→"中右滚筒右轴承":dbl, element #2=→"中右电机左轴承":dbl, element #3=→"中右电机右轴承":dbl, element #4=→"中右电机绕组" →"中右":dbl, element #5=→"后左滚筒左轴承":dbl, element #6=→"后左滚筒右轴承":dbl, element #7=→"后左电机左轴承":dbl, element #8=→"后左电机右轴承":dbl)  [unwired: 8 in]
            n1105 = call "泵压力标定.vi"("振动泵信号输入"=w1716) -> ("振动泵压力输出"=w1701:dbl)  [unwired: 10 in]
            n1106 = Index Array(array=w1708) -> (element #1=w1570:dbl, element #2=w1568:dbl, element #4=w1565:dbl, element #5=w1562:dbl, element #6=w1559:dbl)  [unwired: 6 in, 1 out]
            n1107 = Divide(x=w1704, y=10.0) -> (x/y=→"振动泵压力":dbl)
            n1108 = Divide(x=w1701, y=10.0) -> (x/y=→"转向泵压力":dbl)
            n1109 = Add(x=w1570, y=920.0) -> (x+y=→"中左滚筒左轴承振动":dbl)
            n1110 = Add(x=w1568, y=1000.0) -> (x+y=→"中左滚筒右轴承振动":dbl)
            n1111 = Add(x=w1565, y=1000.0) -> (x+y=→"中左电机右轴承振动":dbl)
            n1112 = for {
              N: 8 -> [_]
              tunnel: w1724 -> [w1771] mode=indexing
              tunnel: [w1770] -> w1726 mode=indexing
              n1113 = call "温度标定.vi"("输入电压"=w1771) -> ("输出温度"=w1770:dbl)  [unwired: 10 in]
            }
            n1114 = Add(x=w1562, y=1000.0) -> (x+y=→"中右滚筒左振动":dbl)
            n1115 = Add(x=w1559, y=1000.0) -> (x+y=→"中右滚筒右振动":dbl)
            n1116 = Index Array(array=w1680, index #1=1 ("索引"), index #2=4 ("索引")) -> (element #1=w1677:dbl, element #2=w1673:dbl)
            n1117 = for {
              N: 8 -> [_]
              tunnel: w1680 -> [w1768] mode=indexing
              tunnel: [w1768] -> w1706 mode=indexing
            }
            n1118 = Index Array(array=w1726) -> (element #1=→"后左电机绕组" →"后左":dbl, element #2=→"后右滚筒左轴承":dbl, element #3=→"后左滚筒右轴承":dbl, element #4=→"后右滚筒左轴承":dbl, element #5=→"后右电机右轴承":dbl, element #6=→"后右电机绕组" →"后右":dbl)  [unwired: 6 in]
            n1119 = Subtract(x=w1673, y=0.0) -> (x-y=→"后左电机左振动":dbl)
            n1120 = Subtract(x=w1677, y=0.0) -> (x-y=→"中右电机右振动":dbl)
            n1121 = Index Array(array=w1706) -> (element #1=w1550:dbl, element #3=w1556:dbl, element #4=w1553:dbl, element #6=w1583:dbl, element #7=w1580:dbl, element #8=w1577:dbl)  [unwired: 8 in, 2 out]
            n1122 = Index Array(array=w1705) -> (element #1=w1574:dbl, element #2=w1683:dbl, element #3=w1593:dbl, element #4=w1591:dbl, element #5=w1589:dbl, element #6=w1588:dbl, element #7=w1586:dbl, element #8=→"前左滚筒左轴承振动":dbl)  [unwired: 8 in]
            n1123 = Add(x=w1583, y=1000.0) -> (x+y=→"后左电机右振动":dbl)
            n1124 = Add(x=w1550, y=1000.0) -> (x+y=→"中右电机左振动":dbl)
            n1125 = Add(x=w1577, y=1000.0) -> (x+y=→"后右滚筒右振动":dbl)
            n1126 = Add(x=w1580, y=950.0) -> (x+y=→"后右滚筒左振动":dbl)
            n1127 = Add(x=w1556, y=1000.0) -> (x+y=→"后左滚筒左振动":dbl)
            n1128 = Add(x=w1553, y=1000.0) -> (x+y=→"后左滚筒右振动":dbl)
            n1129 = for {
              tunnel: w1692 -> [w1767] mode=indexing
              tunnel: [w1767] -> w1691 mode=indexing
            }
            n1130 = Subtract(x=w1683, y=0.0) -> (x-y=→"后右电机右振动":dbl)
            n1131 = call "变矩器及前轮左右温度标定.vi"("变矩器，前轮左和右信号输入"=w1588) -> ("变矩器，前轮左和右信号输出"=→"右前轮轴承温度标定":dbl)  [unwired: 10 in]
            n1132 = call "温度标定.vi"("输入电压"=w1586) -> ("输出温度"=→"左前轮轴承温度标定":dbl)  [unwired: 10 in]
            n1133 = call "温度标定.vi"("输入电压"=w1589) -> ("输出温度"=→"变矩器出口温度标定":dbl)  [unwired: 10 in]
            n1134 = call "温度标定.vi"("输入电压"=w1591) -> ("输出温度"=→"液压油箱温度标定":dbl)  [unwired: 10 in]
            n1135 = call "环境温度标定.vi"("环境温度信号输入"=w1593) -> ("环境温度输出"=→"环境温度标定":dbl)  [unwired: 10 in]
            n1136 = Add(x=w1574, y=900.0) -> (x+y=→"后右电机左振动":dbl)
            n1137 = Index Array(array=w1691) -> (element #1=→"前左滚筒右轴承振动":dbl, element #2=→"前左电机左轴承振动":dbl, element #3=→"前左电机右轴承振动":dbl, element #4=→"前右滚筒左轴承振动":dbl, element #5=→"前右滚筒右轴承振动":dbl, element #6=→"前右电机左轴承振动":dbl, element #7=→"前右电机右轴承振动":dbl)  [unwired: 8 in, 1 out]
            n1138 = local read "中右电机绕组"() -> (w1662:dbl)
            n1139 = local read "中左电机绕组"() -> (w1656:dbl)
            n1140 = local read "前右电机绕组"() -> (w1651:dbl)
            n1141 = local read "前左电机绕组"() -> (w1646:dbl)
            n1142 = local read "后左滚筒右轴承"() -> (w1666:dbl)
            n1143 = local read "后左滚筒左轴承"() -> (w1665:dbl)
            n1144 = local read "后左电机右轴承"() -> (w1664:dbl)
            n1145 = local read "后左电机左轴承"() -> (w1663:dbl)
            n1146 = local read "液压油箱温度标定"() -> (w1643:dbl)
            n1147 = local read "变矩器出口温度标定"() -> (w1642:dbl)
            n1148 = local read "右前轮轴承温度标定"() -> (w1641:dbl)
            n1149 = local read "中右电机右轴承"() -> (w1661:dbl)
            n1150 = local read "中右电机左轴承"() -> (w1660:dbl)
            n1151 = local read "中右滚筒右轴承"() -> (w1659:dbl)
            n1152 = local read "中右滚筒左轴承"() -> (w1658:dbl)
            n1153 = local read "前右滚筒左轴承"() -> (w1657:dbl)
            n1154 = local read "中左电机右轴承"() -> (w1655:dbl)
            n1155 = local read "中左电机左轴承"() -> (w1654:dbl)
            n1156 = local read "中左滚筒左轴承"() -> (w1653:dbl)
            n1157 = local read "中左滚筒右轴承"() -> (w1652:dbl)
            n1158 = local read "前右电机右轴承"() -> (w1650:dbl)
            n1159 = local read "前左滚筒右轴承"() -> (w1649:dbl)
            n1160 = local read "前右滚筒左轴承"() -> (w1648:dbl)
            n1161 = local read "前左电机左轴承"() -> (w1647:dbl)
            n1162 = local read "前左电机右轴承"() -> (w1645:dbl)
            n1163 = local read "前左滚筒左轴承"() -> (w1644:dbl)
            n1164 = local read "左前轮轴承温度标定"() -> (w1600:dbl)
            n1165 = local read "前左滚筒右轴承"() -> (w1598:dbl)
            n1166 = local read "前左"() -> (w1640:dbl)
            n1167 = local read "中左"() -> (w1639:dbl)
            n1168 = local read "后右"() -> (w1638:dbl)
            n1169 = local read "后左"() -> (w1637:dbl)
            n1170 = local read "后右"() -> (w1636:dbl)
            n1171 = local read "中右"() -> (w1635:dbl)
            n1172 = Build Array(w1666, w1665, w1664, w1663, w1662, w1661, w1660, w1659, w1658, w1657, w1656, w1655, w1654, w1653, w1652, w1651, w1650, w1649, w1648, w1647, w1646, w1645, w1644, w1643, w1642, w1641, w1640, w1639, w1638, w1637, w1636, w1635, w1600, w1598) -> (w1634:dbl[])
            n1173 = for {
              tunnel: w1634 -> [w1766] mode=indexing
              tunnel: [w1765] -> w1633 mode=indexing
              n1174 = call "报警判断 (子VI).vi"("后左滚筒右轴承"=w1766) -> ("布尔"=w1765:bool)  [unwired: 10 in]
            }
            n1175 = Index Array(array=w1633) -> (element #1=w1632:bool, element #2=w1631:bool, element #3=w1630:bool, element #4=w1629:bool, element #5=w1628:bool, element #6=w1627:bool, element #7=w1626:bool, element #8=w1625:bool, element #9=w1624:bool, element #10=w1623:bool, element #11=w1622:bool, element #12=w1621:bool, element #13=w1620:bool, element #14=w1619:bool, element #15=w1618:bool, element #16=w1617:bool, element #17=w1616:bool, element #18=w1615:bool, element #19=w1614:bool, element #20=w1613:bool, element #21=w1612:bool, element #22=w1611:bool, element #23=w1610:bool, element #24=w1609:bool, element #25=w1608:bool, element #26=w1607:bool, element #27=w1606:bool, element #28=w1605:bool, element #29=w1604:bool, element #30=w1603:bool, element #31=w1602:bool, element #32=w1601:bool, element #33=w1599:bool, element #34=w1597:bool)  [unwired: 34 in]
            n1176 = Compound Arithmetic op=OR ("复合运算")(w1632, w1631, w1630, w1629, w1628, w1627, w1626, w1625, w1624, w1623, w1622, w1621, w1620, w1619, w1618, w1617, w1616, w1615, w1614, w1613, w1612, w1611, w1610, w1609, w1608, w1607, w1606, w1605, w1604, w1603, w1602, w1601, w1599, w1597) -> (w1594:bool)
            n1177 = case shown="真" w1594 {
              frame False {
                n1178 = local write "超温报警"(FALSE ("超温报警")) -> ()
              }
              frame True {
                "超温报警" <- TRUE ("超温报警")
              }
            }
            n1179 = call <vilib>:"Boolean Crossing PtByPt.vi"("direction"=enum16{"either", "false-true", "true-false"}."false-true", "input"=w1594) -> ("crossing"=w1596:bool)  [unwired: 1 in]
            n1180 = case shown="真" w1596 {
              frame False {
              }
              frame True {
                "对话框传递" <- TRUE ("对话框传递")
              }
            }
          }
          frame "退出" {
          }
        }
      }
    }
    frame #2 {
    }
  }
  n1181 = while "主线程" {
    shift-right: [w2211] -> _
    shift-left: enum16{"Init", "Wait", "Run", "Exit"}."Init" -> [w2201]
    shift-right: [w2212] -> _
    shift-left: _ -> [w2213]
    shift-right: [w2210] -> _
    shift-left: _ -> [w2209]
    shift-right: [w2208] -> _
    shift-left: _ -> [w2207]
    shift-right: [w2206] -> _
    shift-left: _ -> [w2205]
    shift-right: [w2203] -> _
    shift-left: u32 0 -> [w2204]
    tunnel: [w2202] -> w4
    stop <- w2199 stop-if-true
    # "CAN Status"
    # "Config"
    # "EventReg"
    # "UpdateUIEvent"
    # "SendCnt"
    n1182 = Equal?(x=w2201, y=enum16{"Init", "Wait", "Run", "Exit"}."Exit") -> (x = y?=w2199:bool)
    n1183 = case shown="\"Run\"" w2201 {
      tunnel: w2213 -> [_ w2245 w2355 w2625]
      tunnel: [w2236 w2244 w2354 w2625] -> w2212
      tunnel: [enum16{"Init", "Wait", "Run", "Exit"}."Wait" w2241 w2356 enum16{"Init", "Wait", "Run", "Exit"}."Exit"] -> w2211
      tunnel: [w2232 w2242 w2353 w2623] -> w2210
      tunnel: w2209 -> [_ w2243 w2353 w2623]
      tunnel: [w2224 w2240 w2351 w2628] -> w2208
      tunnel: w2207 -> [_ w2240 w2352 w2628]
      tunnel: [w2223 w2239 w2350 w2626] -> w2206
      tunnel: w2205 -> [_ w2239 w2350 w2626]
      tunnel: w2204 -> [w2221 w2238 w2349 w2621]
      tunnel: [w2221 w2238 w2348 w2621] -> w2203
      tunnel: [_ _ _ errorcluster {"status"=FALSE, "code"=0, "source"=""} ("error constant")] -> w2202
      frame "Init", Default {
        w2225 = cluster{"CANOpen":bool} {"CANOpen"=FALSE}  # UpdateUI
        w2235 = T9 {"DevType"=2, "DevIndex"=0, "CanIndex"=0, "VCI_INIT_CONFIG"={"AccCode"=0, "AccMask"=0, "InitFlag"=0, "Fliter"=0, "Timing0"=0, "Timing1"=0, "Mode"=0}}  # Config
        w2236 = cluster{"Open":bool, "SendCnt":u32} {"Open"=FALSE, "SendCnt"=0}  # CAN Status
        n1184 = local write "comcnt"(u16 0 ("comcnt")) -> ()
        n1185 = local write "停止"(FALSE ("停止")) -> ()
        n1186 = local write "Open"(FALSE ("Open")) -> ()
        n1187 = property class="VI"("Front Panel.Closeable"=TRUE ("前面板窗口:可关闭")) -> ()  [unwired: 2 in, 2 out]
        n1188 = call "Demo_GetT0T1.vi"("kBaudRate"="kBaudRate") -> ("Timing0"=w2218:u8, "Timing1"=w2217:u8)
        n1189 = Bundle By Name(cluster=w2235, "DevType"="DevType", "CanIndex"="Channel", "VCI_INIT_CONFIG.AccCode"="AccCode", "VCI_INIT_CONFIG.AccMask"="AccMask", "VCI_INIT_CONFIG.InitFlag"="InitFlag", "VCI_INIT_CONFIG.Fliter"="Fliter", "VCI_INIT_CONFIG.Timing0"=w2218, "VCI_INIT_CONFIG.Timing1"=w2217, "VCI_INIT_CONFIG.Mode"="Mode") -> (w2232:T9)
        n1190 = local write "RcvEnable"(TRUE ("RcvEnable")) -> ()
        n1191 = Create User Event(user event datatype=w2225) -> (user event=w2223:refnum<user-event>)  [unwired: 1 in, 1 out]
        n1192 = register-events(w2223) -> (reference out=w2224:refnum<event-registration>)  [unwired: 2 in, 1 out]
        "Config" <- w2235
      }
      frame "Wait" {
        n1193 = event shown="[10] 超时" {
          selector: _ -> [_ _ _ _ _ _ _ _ _ _ _]
          dyn-events: _ -> [_ _ _ _ _ _ _ _ _ _ _]
          timeout: 50 -> [_ _ _ _ _ _ _ _ _ _ _]
          tunnel: w2245 -> [w2249 w2303 w2306 w2311 w2316 w2321 w2326 w2331 w2338 w2343 w2346]
          tunnel: [w2248 w2303 w2306 w2311 w2316 w2321 w2326 w2331 w2338 w2343 w2346] -> w2244
          tunnel: w2243 -> [w2251 w2302 w2305 w2310 w2315 w2320 w2325 w2330 w2337 w2342 w2345]
          tunnel: [w2251 w2301 w2305 w2308 w2313 w2318 w2323 w2328 w2336 w2340 w2345] -> w2242
          tunnel: [w2250 enum16{"Init", "Wait", "Run", "Exit"}."Wait" enum16{"Init", "Wait", "Run", "Exit"}."Exit" enum16{"Init", "Wait", "Run", "Exit"}."Wait" enum16{"Init", "Wait", "Run", "Exit"}."Wait" enum16{"Init", "Wait", "Run", "Exit"}."Wait" enum16{"Init", "Wait", "Run", "Exit"}."Wait" enum16{"Init", "Wait", "Run", "Exit"}."Wait" enum16{"Init", "Wait", "Run", "Exit"}."Wait" enum16{"Init", "Wait", "Run", "Exit"}."Wait" enum16{"Init", "Wait", "Run", "Exit"}."Wait"] -> w2241
          tunnel: w2239 -> [w2247 _ _ _ _ _ _ _ _ _ _]
          event Menu Selection (User) {
            n1194 = event-data() -> ("ItemTag"=w2246:string)  [unwired: 8 out]
            n1195 = case shown="\"遥控器\"" w2246 {
              tunnel: w2251 -> [_ w2267]
              tunnel: [enum16{"Init", "Wait", "Run", "Exit"}."Wait" w2258] -> w2250
              tunnel: w2249 -> [w2253 w2257]
              tunnel: [w2253 w2256] -> w2248
              tunnel: w2247 -> [_ w2255]
              frame "假", Default {
              }
              frame "遥控器" {
                w2261 = T21 1 items=["OK"=1, "ERROR1"=0, "ERROR2"=-1] ("y")
                # "打开CAN的步骤：\n1.Open\n2.Init\n3.Start"
                n1196 = Unbundle By Name(w2267) -> ("DevType"=w2266:T3, "DevIndex"=w2265:u32)
                n1197 = call "VCI_OpenDevice.vi"("DevIndex"=w2265, "DevType"=w2266) -> ("error out"=w2262:errorcluster, "Return Val"=w2264:T21)  [unwired: 2 in, 6 out]
                n1198 = Equal?(x=w2264, y=w2261) -> (x = y?=w2263:bool)
                n1199 = case shown="真" w2263 {
                  tunnel: w2262 -> [_ w2282]
                  tunnel: w2267 -> [_ w2281]
                  tunnel: w2261 -> [_ w2273]
                  tunnel: [_ w2272] -> w2254
                  frame False {
                  }
                  frame True {
                    n1200 = Unbundle By Name(w2281) -> ("VCI_INIT_CONFIG"=w2280:T5, "DevType"=w2276:T3, "DevIndex"=w2275:u32, "CanIndex"=w2274:T4)
                    n1201 = call "VCI_InitCAN.vi"("VCI_INIT_CONFIG"=w2280, "error in (no error)"=w2282, "CANIndex"=w2274, "DevIndex"=w2275, "DevType"=w2276) -> ("error out"=w2277:errorcluster, "Return Val"=w2279:T21)  [unwired: 5 out]
                    n1202 = Equal?(x=w2273, y=w2279) -> (x = y?=w2278:bool)
                    n1203 = case shown="真" w2278 {
                      tunnel: w2277 -> [_ w2293]
                      tunnel: w2276 -> [_ w2292]
                      tunnel: w2275 -> [_ w2291]
                      tunnel: w2274 -> [_ w2290]
                      tunnel: w2273 -> [_ w2288]
                      tunnel: [_ w2284] -> w2272
                      frame False {
                      }
                      frame True {
                        n1204 = call "VCI_StartCAN.vi"("error in (no error)"=w2293, "CANIndex"=w2290, "DevIndex"=w2291, "DevType"=w2292) -> ("error out"=w2286:errorcluster, "Return Val"=w2289:T21)  [unwired: 6 out]
                        n1205 = Unbundle By Name(w2286) -> ("status"=w2283:bool)
                        n1206 = Equal?(x=w2288, y=w2289) -> (x = y?=w2287:bool)
                        n1207 = Not(x=w2283) -> (.not. x?=w2285:bool)
                        n1208 = And(x=w2287, y=w2285) -> (x .and. y?=w2284:bool)
                      }
                    }
                  }
                }
                n1209 = case shown="真" w2254 {
                  tunnel: w2255 -> [_ w2271]
                  tunnel: w2254 -> [_ w2269]
                  frame False {
                  }
                  frame True {
                    n1210 = Bundle By Name(cluster=cluster{"CANOpen":bool} {"CANOpen"=FALSE} ("事件数据"), "CANOpen"=w2269) -> (w2268:cluster{"CANOpen":bool})
                    n1211 = Generate User Event(user event=w2271, event data cluster=w2268) -> ()  [unwired: 2 in, 2 out]
                  }
                }
                n1212 = Select(t=enum16{"Init", "Wait", "Run", "Exit"}."Run", s=w2254, f=enum16{"Init", "Wait", "Run", "Exit"}."Wait") -> (s? t:f=w2258:enum16{"Init", "Wait", "Run", "Exit"})
                n1213 = Bundle By Name(cluster=w2257, "Open"=w2254) -> (w2256:cluster{"Open":bool, "SendCnt":u32})
              }
            }
          }
          event Value Change {
            w2299 = T3 3 items=["USB-CAN"=2, "USB-CAN2"=3] ("y")
            n1214 = event-data() -> ("NewVal"=w2300:T3)  [unwired: 1 out]
            n1215 = Equal?(x=w2300, y=w2299) -> (x = y?=w2298:bool)
            n1216 = Bundle By Name(cluster=w2302, "DevType"=w2300) -> (w2301:T9)
            n1217 = Select(t=i32[] [] ("禁用项[]"), s=w2298, f=i32[] [1] ("禁用项[]")) -> (s? t:f=w2297:i32[])
            n1218 = property on="Channel" class="Ring (严格)"("Disabled Items []"=w2297) -> ()  [unwired: 2 in, 2 out]
          }
          event "停止": Value Change {
            n1219 = event-data() -> ()  [unwired: 7 out]
          }
          event Value Change {
            n1220 = event-data() -> ("NewVal"=w2309:T4)  [unwired: 1 out]
            n1221 = Bundle By Name(cluster=w2310, "CanIndex"=w2309) -> (w2308:T9)
          }
          event "AccCode": Value Change {
            n1222 = event-data() -> ("NewVal"=w2314:u32)  [unwired: 1 out]
            n1223 = Bundle By Name(cluster=w2315, "VCI_INIT_CONFIG.AccCode"=w2314) -> (w2313:T9)
          }
          event "AccMask": Value Change {
            n1224 = event-data() -> ("NewVal"=w2319:u32)  [unwired: 1 out]
            n1225 = Bundle By Name(cluster=w2320, "VCI_INIT_CONFIG.AccMask"=w2319) -> (w2318:T9)
          }
          event Value Change {
            n1226 = event-data() -> ("NewVal"=w2324:T6)  [unwired: 1 out]
            n1227 = Bundle By Name(cluster=w2325, "VCI_INIT_CONFIG.InitFlag"=w2324) -> (w2323:T9)
          }
          event Value Change {
            n1228 = event-data() -> ("NewVal"=w2329:T8)  [unwired: 1 out]
            n1229 = Bundle By Name(cluster=w2330, "VCI_INIT_CONFIG.Mode"=w2329) -> (w2328:T9)
          }
          event "kBaudRate": Value Change {
            n1230 = event-data() -> ("NewVal"=w2334:u8)  [unwired: 1 out]
            n1231 = call "Demo_GetT0T1.vi"("kBaudRate"=w2334) -> ("Timing0"=w2333:u8, "Timing1"=w2332:u8)
            n1232 = Bundle By Name(cluster=w2337, "VCI_INIT_CONFIG.Timing0"=w2333, "VCI_INIT_CONFIG.Timing1"=w2332) -> (w2336:T9)
          }
          event Value Change {
            n1233 = event-data() -> ("NewVal"=w2341:T7)  [unwired: 1 out]
            n1234 = Bundle By Name(cluster=w2342, "VCI_INIT_CONFIG.Fliter"=w2341) -> (w2340:T9)
          }
          event Timeout {
            n1235 = event-data() -> ()  [unwired: 4 out]
          }
        }
      }
      frame "Run" {
        n1236 = event shown="[0] 超时" {
          selector: w2352 -> [_ _ _ _]
          dyn-events: [_ _ _ _] -> w2351
          timeout: 100 -> [_ _ _ _]
          tunnel: [enum16{"Init", "Wait", "Run", "Exit"}."Run" enum16{"Init", "Wait", "Run", "Exit"}."Run" enum16{"Init", "Wait", "Run", "Exit"}."Run" w2614] -> w2356
          tunnel: [w2361 w2588 w2597 w2615] -> w2354
          tunnel: w2355 -> [w2361 w2588 w2599 w2615]
          tunnel: w2353 -> [w2360 w2583 w2604 _]
          tunnel: w2350 -> [_ _ w2596 _]
          tunnel: w2349 -> [w2358 w2573 w2592 w2613]
          tunnel: [w2359 w2572 w2592 w2613] -> w2348
          event Timeout {
            n1237 = event-data() -> ()  [unwired: 4 out]
            n1238 = local read "Open"() -> (w2357:bool)
            n1239 = case shown="真" w2357 {
              tunnel: w2360 -> [_ w2378]
              tunnel: [w2363 w2377] -> w2359
              tunnel: w2358 -> [w2363 w2376]
              frame False {
              }
              frame True {
                n1240 = local read "发送左侧字符"() -> (w2365:bool)
                n1241 = case shown="假" w2365 {
                  tunnel: [w2467 w2518] -> w2375
                  tunnel: [w2465 w2517] -> w2368
                  tunnel: [w2464 w2516] -> w2367
                  tunnel: [w2461 w2515] -> w2366
                  tunnel: [w2380 w2469] -> w2364
                  frame False {
                    # "扭矩"
                    # "功率"
                    # "车速"
                    # "档位"
                    # "右侧数据"
                    n1242 = Build Array("0byte 8", "1byte 8", "2byte 8", "3byte 8", "4byte 8", "5byte 8", "6byte 8", "7byte 8") -> (w2424:u8[])
                    n1243 = Build Array("0byte 5", "1byte 5", "2byte 5", "3byte 5", "4byte 5", "5byte 5", "6byte 5", "7byte 5") -> (w2397:u8[])
                    n1244 = Build Array("0byte 6", "1byte 6", "2byte 6", "3byte 6", "4byte 6", "5byte 6", "6byte 6", "7byte 6") -> (w2406:u8[])
                    n1245 = Build Array("0byte 7", "1byte 7", "2byte 7", "3byte 7", "4byte 7", "5byte 7", "6byte 7", "7byte 7") -> (w2415:u8[])
                    n1246 = call "遥控器IP地址参数.vi"("数组"=w2397, "ID_VCU_MCU_1输入"="ID_VCU_MCU_1 5") -> ("Send"=w2384:T12)  [unwired: 9 in]
                    n1247 = call "遥控器IP地址参数.vi"("数组"=w2406, "ID_VCU_MCU_1输入"="ID_VCU_MCU_1 6") -> ("Send"=w2383:T12)  [unwired: 9 in]
                    n1248 = call "遥控器IP地址参数.vi"("数组"=w2415, "ID_VCU_MCU_1输入"="ID_VCU_MCU_2 4") -> ("Send"=w2382:T12)  [unwired: 9 in]
                    n1249 = call "遥控器IP地址参数.vi"("数组"=w2424, "ID_VCU_MCU_1输入"="ID_VCU_MCU_33 3") -> ("Send"=w2381:T12)  [unwired: 9 in]
                    n1250 = Build Array(w2384, w2383, w2382, w2381) -> (w2380:T12[])
                    n1251 = Build Array("0byte 4", "1byte 4", "2byte 4", "3byte 4", "4byte 4", "5byte 4", "6byte 4", "7byte 4") -> (w2425:u8[])
                    n1252 = Build Array("0byte", "1byte", "2byte", "3byte", "4byte", "5byte", "6byte", "7byte") -> (w2452:u8[])
                    n1253 = Build Array("0byte 2", "1byte 2", "2byte 2", "3byte 2", "4byte 2", "5byte 2", "6byte 2", "7byte 2") -> (w2443:u8[])
                    n1254 = Build Array("0byte 3", "1byte 3", "2byte 3", "3byte 3", "4byte 3", "5byte 3", "6byte 3", "7byte 3") -> (w2434:u8[])
                    n1255 = call "遥控器IP地址参数.vi"("数组"=w2452, "ID_VCU_MCU_1输入"="ID_VCU_MCU_1 2") -> ("Send"=w2467:T12)  [unwired: 9 in]
                    n1256 = call "遥控器IP地址参数.vi"("数组"=w2443, "ID_VCU_MCU_1输入"="ID_VCU_MCU_1") -> ("Send"=w2465:T12)  [unwired: 9 in]
                    n1257 = call "遥控器IP地址参数.vi"("数组"=w2434, "ID_VCU_MCU_1输入"="ID_VCU_MCU_2 2") -> ("Send"=w2464:T12)  [unwired: 9 in]
                    n1258 = call "遥控器IP地址参数.vi"("数组"=w2425, "ID_VCU_MCU_1输入"="ID_VCU_MCU_33") -> ("Send"=w2461:T12)  [unwired: 9 in]
                    "发送左侧字符" <- TRUE ("发送左侧字符")
                  }
                  frame True {
                    # "左侧字符串"
                    n1259 = Build Array("0byte 16", "1byte 16", "2byte 16", "3byte 16", "4byte 16", "5byte 16", "6byte 16", "7byte 16") -> (w2513:u8[])
                    n1260 = Build Array("0byte 13", "1byte 13", "2byte 13", "3byte 13", "4byte 13", "5byte 13", "6byte 13", "7byte 13") -> (w2486:u8[])
                    n1261 = Build Array("0byte 14", "1byte 14", "2byte 14", "3byte 14", "4byte 14", "5byte 14", "6byte 14", "7byte 14") -> (w2495:u8[])
                    n1262 = Build Array("0byte 15", "1byte 15", "2byte 15", "3byte 15", "4byte 15", "5byte 15", "6byte 15", "7byte 15") -> (w2504:u8[])
                    n1263 = call "遥控器IP地址参数.vi"("数组"=w2486, "ID_VCU_MCU_1输入"="ID_VCU_MCU_1 7") -> ("Send"=w2473:T12)  [unwired: 9 in]
                    n1264 = call "遥控器IP地址参数.vi"("数组"=w2495, "ID_VCU_MCU_1输入"="ID_VCU_MCU_1 8") -> ("Send"=w2472:T12)  [unwired: 9 in]
                    n1265 = call "遥控器IP地址参数.vi"("数组"=w2504, "ID_VCU_MCU_1输入"="ID_VCU_MCU_2 5") -> ("Send"=w2471:T12)  [unwired: 9 in]
                    n1266 = call "遥控器IP地址参数.vi"("数组"=w2513, "ID_VCU_MCU_1输入"="ID_VCU_MCU_33 4") -> ("Send"=w2470:T12)  [unwired: 9 in]
                    n1267 = Build Array(w2473, w2472, w2471, w2470) -> (w2469:T12[])
                    n1268 = Build Array("0byte 12", "1byte 12", "2byte 12", "3byte 12", "4byte 12", "5byte 12", "6byte 12", "7byte 12") -> (w2519:u8[])
                    n1269 = Build Array("0byte 9", "1byte 9", "2byte 9", "3byte 9", "4byte 9", "5byte 9", "6byte 9", "7byte 9") -> (w2546:u8[])
                    n1270 = Build Array("0byte 10", "1byte 10", "2byte 10", "3byte 10", "4byte 10", "5byte 10", "6byte 10", "7byte 10") -> (w2537:u8[])
                    n1271 = Build Array("0byte 11", "1byte 11", "2byte 11", "3byte 11", "4byte 11", "5byte 11", "6byte 11", "7byte 11") -> (w2528:u8[])
                    n1272 = flat-sequence {
                      tunnel: FALSE ("发送左侧字符") -> [w2560]
                      frame #0 {
                        n1273 = local write "发送左侧字符"(w2560) -> ()
                        n1274 = Wait (ms)(milliseconds to wait=u32 100 ("等待时间（毫秒）")) -> ()  [unwired: 1 out]
                      }
                    }
                    n1275 = call "遥控器IP地址参数.vi"("数组"=w2546, "ID_VCU_MCU_1输入"="ID_VCU_MCU_1 3") -> ("Send"=w2518:T12)  [unwired: 9 in]
                    n1276 = call "遥控器IP地址参数.vi"("数组"=w2537, "ID_VCU_MCU_1输入"="ID_VCU_MCU_1 4") -> ("Send"=w2517:T12)  [unwired: 9 in]
                    n1277 = call "遥控器IP地址参数.vi"("数组"=w2519, "ID_VCU_MCU_1输入"="ID_VCU_MCU_33 2") -> ("Send"=w2515:T12)  [unwired: 9 in]
                    n1278 = call "遥控器IP地址参数.vi"("数组"=w2528, "ID_VCU_MCU_1输入"="ID_VCU_MCU_2 3") -> ("Send"=w2516:T12)  [unwired: 9 in]
                  }
                }
                n1279 = Build Array (concatenate)(w2375, w2368, w2367, w2366, w2364) -> (w2369:T12[])
                n1280 = Unbundle By Name(w2378) -> ("DevType"=w2374:T3, "DevIndex"=w2373:u32, "CanIndex"=w2371:T4)
                n1281 = Get Date/Time In Seconds() -> (seconds since 1Jan1904=w2370:timestamp)
                n1282 = disable-structure shown="禁用" {
                  disable-tunnel: _ -> [w2568 _]
                  disable-tunnel: enum16{"接收", "发送"}."发送" ("Type") -> [w2566 _]
                  disable-tunnel: w2371 -> [w2565 _]
                  disable-tunnel: w2370 -> [w2564 _]
                  disable-tunnel: w2369 -> [w2561 _]
                  frame Disabled {
                    n1283 = Bundle By Name(cluster=T20 {"Type"=enum."发送", "Channel"=0, "Time"=timestamp(0 s since 1904-01-01), "VCI_CAN_OBJ"={"ID"=0, "TimeStamp"=0, "TimeFlag"=0, "SendType"=0, "RemoteFlag"=0, "ExternFlag"=0, "DataLen"=0, "Data"=[], "Reserved"=[]}}, "Type"=w2566, "Channel"=w2565, "Time"=w2564, "VCI_CAN_OBJ"=w2561) -> (w2563:T20)
                    n1284 = Build Array(w2563) -> (w2562:T13)
                    n1285 = Enqueue Element(queue=w2568, element=w2562) -> ()  [unwired: 1 in, 4 out]
                  }
                  frame Enabled {
                  }
                }
                n1286 = call "VCI_Transmit.vi"("Buffer"=w2369, "CANIndex"=w2371, "DevIndex"=w2373, "DevType"=w2374) -> ()  [unwired: 1 in, 7 out]
                n1287 = Increment(x=w2376) -> (x+1=w2377:u32)
                n1288 = local write "SendCnt"(w2377) -> ()
              }
            }
          }
          event "Send": Value Change {
            n1289 = event-data() -> ()  [unwired: 2 out]
            n1290 = Increment(x=w2573) -> (x+1=w2572:u32)
            "SendCnt" <- w2572
            n1291 = call "Demo_MakeData.vi"("DataString"="Data") -> ("Data"=w2578:u8[], "DataLen"=w2579:u8)  [unwired: 9 out]
            n1292 = Bundle By Name(cluster=T12 {"ID"=0, "TimeStamp"=0, "TimeFlag"=0, "SendType"=0, "RemoteFlag"=0, "ExternFlag"=0, "DataLen"=0, "Data"=[], "Reserved"=[]} ("Send"), "ID"="ID", "RemoteFlag"="Type", "ExternFlag"="Format", "DataLen"=w2579, "Data"=w2578) -> (w2570:T12)
            n1293 = Build Array(w2570) -> (w2571:T12[])
            n1294 = Get Date/Time In Seconds() -> (seconds since 1Jan1904=w2574:timestamp)
            n1295 = Unbundle By Name(w2583) -> ("DevType"=w2582:T3, "DevIndex"=w2581:u32, "CanIndex"=w2575:T4)
            n1296 = Bundle By Name(cluster=T20 {"Type"=enum."发送", "Channel"=0, "Time"=timestamp(0 s since 1904-01-01), "VCI_CAN_OBJ"={"ID"=0, "TimeStamp"=0, "TimeFlag"=0, "SendType"=0, "RemoteFlag"=0, "ExternFlag"=0, "DataLen"=0, "Data"=[], "Reserved"=[]}}, "Type"=enum16{"接收", "发送"}."发送", "Channel"=w2575, "Time"=w2574, "VCI_CAN_OBJ"=w2570) -> (w2569:T20)
            n1297 = call "VCI_Transmit.vi"("Buffer"=w2571, "CANIndex"=w2575, "DevIndex"=w2581, "DevType"=w2582) -> ()  [unwired: 1 in, 7 out]
            n1298 = disable-structure shown="禁用" {
              disable-tunnel: w2569 -> [w2591 _]
              frame Disabled {
                n1299 = Build Array(w2591) -> (w2590:T13)
                n1300 = Enqueue Element(element=w2590) -> ()  [unwired: 2 in, 4 out]
              }
              frame Enabled {
              }
            }
          }
          event "停止": Value Change {
            w2600 = T21 1 items=["OK"=1, "ERROR1"=0, "ERROR2"=-1] ("y")
            n1301 = event-data() -> ()  [unwired: 7 out]
            n1302 = Unbundle By Name(w2604) -> ("DevType"=w2603:T3, "DevIndex"=w2602:u32)
            n1303 = call "VCI_CloseDevice.vi"("DevIndex"=w2602, "DevType"=w2603) -> ("Return Val"=w2601:T21)  [unwired: 1 in, 8 out]
            n1304 = Equal?(x=w2601, y=w2600) -> (x = y?=w2598:bool)
            n1305 = Not(x=w2598) -> (.not. x?=w2594:bool)
            n1306 = Bundle By Name(cluster=cluster{"CANOpen":bool} {"CANOpen"=FALSE} ("事件数据"), "CANOpen"=w2594) -> (w2593:cluster{"CANOpen":bool})
            n1307 = Bundle By Name(cluster=w2599, "Open"=w2594) -> (w2597:cluster{"Open":bool, "SendCnt":u32})
            n1308 = local write "Open"(w2594) -> ()
            n1309 = Generate User Event(user event=w2596, event data cluster=w2593) -> ()  [unwired: 2 in, 2 out]
          }
          event User Event {
            w2610 = 0
            w2609 = 2
            n1310 = event-data() -> ("CANOpen"=w2612:bool)  [unwired: 1 out]
            "Open" <- w2612
            n1311 = disable-structure shown="禁用" {
              disable-tunnel: w2612 -> [w2617 _]
              frame Disabled {
                n1312 = Not(x=w2617) -> (.not. x?=w2616:bool)
                n1313 = property class="VI"("Front Panel.Closeable"=w2616) -> ()  [unwired: 2 in, 2 out]
              }
              frame Enabled {
              }
            }
            n1314 = Select(t=w2609, s=w2612, f=w2610) -> (s? t:f=w2611:i32)
            n1315 = Select(t=w2610, s=w2612, f=w2609) -> (s? t:f=w2606:i32)
            n1316 = Select(t=enum16{"Init", "Wait", "Run", "Exit"}."Run", s=w2612, f=enum16{"Init", "Wait", "Run", "Exit"}."Wait") -> (s? t:f=w2614:enum16{"Init", "Wait", "Run", "Exit"})
            n1317 = disable-structure shown="禁用" {
              disable-tunnel: w2611 -> [w2619 _]
              disable-tunnel: w2606 -> [w2618 _]
              frame Disabled {
                n1318 = property on="Close" class="Bool"("DisabledEnum"=w2618) -> ()  [unwired: 2 in, 2 out]
                n1319 = property on="ID" class="DigNum (严格)"("DisabledEnum"=w2618) -> ()  [unwired: 2 in, 2 out]
                n1320 = property on="Data" class="Str"("DisabledEnum"=w2618) -> ()  [unwired: 2 in, 2 out]
                n1321 = property on="Format" class="Ring (严格)"("DisabledEnum"=w2618) -> ()  [unwired: 2 in, 2 out]
                n1322 = property on="Type" class="Ring (严格)"("DisabledEnum"=w2618) -> ()  [unwired: 2 in, 2 out]
                n1323 = property on="Send" class="Bool"("DisabledEnum"=w2618) -> ()  [unwired: 2 in, 2 out]
                n1324 = property on="Clear" class="Bool"("DisabledEnum"=w2618) -> ()  [unwired: 2 in, 2 out]
                n1325 = property on="Fliter" class="Ring (严格)"("DisabledEnum"=w2619) -> ()  [unwired: 2 in, 2 out]
                n1326 = property on="DevType" class="Ring (严格)"("DisabledEnum"=w2619) -> ()  [unwired: 2 in, 2 out]
                n1327 = property on="Channel" class="Ring (严格)"("DisabledEnum"=w2619) -> ()  [unwired: 2 in, 2 out]
                n1328 = property on="AccCode" class="DigNum (严格)"("DisabledEnum"=w2619) -> ()  [unwired: 2 in, 2 out]
                n1329 = property on="AccMask" class="DigNum (严格)"("DisabledEnum"=w2619) -> ()  [unwired: 2 in, 2 out]
                n1330 = property on="InitFlag" class="Ring (严格)"("DisabledEnum"=w2619) -> ()  [unwired: 2 in, 2 out]
                n1331 = property on="Mode" class="Ring (严格)"("DisabledEnum"=w2619) -> ()  [unwired: 2 in, 2 out]
                n1332 = property on="kBaudRate" class="Ring (严格)"("DisabledEnum"=w2619) -> ()  [unwired: 2 in, 2 out]
                n1333 = property on="Open 2" class="Bool"("DisabledEnum"=w2619) -> ()  [unwired: 2 in, 2 out]
              }
              frame Enabled {
              }
            }
          }
        }
      }
      frame "Exit" {
        n1334 = Unregister For Events(event registration refnum=w2628) -> (error out=w2627:errorcluster)  [unwired: 1 in]
        n1335 = Destroy User Event(user event=w2626, error in=w2627) -> ()  [unwired: 1 out]
        n1336 = Unbundle By Name(w2625) -> ("Open"=w2624:bool)
        n1337 = local write "RcvEnable"(FALSE ("RcvEnable")) -> ()
        n1338 = case shown="真" w2624 {
          tunnel: w2623 -> [_ w2632]
          frame False {
          }
          frame True {
            n1339 = Unbundle By Name(w2632) -> ("DevType"=w2631:T3, "DevIndex"=w2630:u32)
            n1340 = call "VCI_CloseDevice.vi"("DevIndex"=w2630, "DevType"=w2631) -> ()  [unwired: 1 in, 9 out]
          }
        }
      }
    }
  }
  n1341 = flat-sequence {
    frame #0 {
      "启动布尔" <- TRUE ("启动布尔")
      "停止布尔" <- TRUE ("停止布尔")
    }
    frame #1 {
      n1342 = while {
        stop <- w2640 stop-if-true
        n1343 = local read "停止布尔"() -> (→"停止布尔 2":bool)
        n1344 = local read "当前试验档位"() -> (w2638:string)
        n1345 = local read "485启动给遥控器布尔"() -> (w2641:bool)
        n1346 = String Length(string=w2638) -> (length=w2637:i32)
        n1347 = local read "Open"() -> (w2643:bool)
        n1348 = local read "试验开始"() -> (w2635:bool)
        n1349 = Not Equal To 0?(x=w2637) -> (x != 0?=w2636:bool)
        n1350 = Not Equal?(x="无效档" ("y"), y=w2638) -> (x != y?=w2644:bool)
        n1351 = Not Equal?(x=w2638, y="N") -> (x != y?=w2645:bool)
        n1352 = Compound Arithmetic op=AND ("复合运算")(w2645, w2644, w2636, w2643, w2641, w2635) -> (w2642:bool)
        n1353 = case shown="真" w2642 {
          tunnel: w2638 -> [_ w2663]
          frame False {
          }
          frame True {
            n1354 = case shown="\"D6\"" w2663 {
              frame "D1" {
                n1355 = local write "加载电机右上转矩给定"("D1扭矩给定") -> ()
                n1356 = local write "加载电机右下转矩给定"("D1扭矩给定") -> ()
                n1357 = local write "加载电机左下转矩给定"("D1扭矩给定") -> ()
                n1358 = local write "加载电机左上转矩给定"("D1扭矩给定") -> ()
              }
              frame "D2" {
                n1359 = local write "加载电机右上转矩给定"("D2扭矩给定") -> ()
                n1360 = local write "加载电机右下转矩给定"("D2扭矩给定") -> ()
                n1361 = local write "加载电机左下转矩给定"("D2扭矩给定") -> ()
                n1362 = local write "加载电机左上转矩给定"("D2扭矩给定") -> ()
              }
              frame "D3" {
                n1363 = local write "加载电机右上转矩给定"("D3扭矩给定") -> ()
                n1364 = local write "加载电机右下转矩给定"("D3扭矩给定") -> ()
                n1365 = local write "加载电机左下转矩给定"("D3扭矩给定") -> ()
                n1366 = local write "加载电机左上转矩给定"("D3扭矩给定") -> ()
              }
              frame "D4" {
                n1367 = local write "加载电机右上转矩给定"("D4扭矩给定") -> ()
                n1368 = local write "加载电机右下转矩给定"("D4扭矩给定") -> ()
                n1369 = local write "加载电机左下转矩给定"("D4扭矩给定") -> ()
                n1370 = local write "加载电机左上转矩给定"("D4扭矩给定") -> ()
              }
              frame "D5" {
                n1371 = local write "加载电机右上转矩给定"("D5扭矩给定") -> ()
                n1372 = local write "加载电机右下转矩给定"("D5扭矩给定") -> ()
                n1373 = local write "加载电机左下转矩给定"("D5扭矩给定") -> ()
                n1374 = local write "加载电机左上转矩给定"("D5扭矩给定") -> ()
              }
              frame "D6" {
                n1375 = local write "加载电机右上转矩给定"("D6扭矩给定") -> ()
                n1376 = local write "加载电机右下转矩给定"("D6扭矩给定") -> ()
                n1377 = local write "加载电机左下转矩给定"("D6扭矩给定") -> ()
                n1378 = local write "加载电机左上转矩给定"("D6扭矩给定") -> ()
              }
              frame "R1" {
                n1379 = Multiply(x="R1扭矩给定", y=i16 -1) -> (x*y=w2684:i16)
                n1380 = local write "加载电机右上转矩给定"(w2684) -> ()
                n1381 = local write "加载电机右下转矩给定"(w2684) -> ()
                n1382 = local write "加载电机左下转矩给定"(w2684) -> ()
                n1383 = local write "加载电机左上转矩给定"(w2684) -> ()
              }
              frame "R2" {
                n1384 = Multiply(x="R2扭矩给定", y=i16 -1) -> (x*y=w2687:i16)
                n1385 = local write "加载电机右上转矩给定"(w2687) -> ()
                n1386 = local write "加载电机右下转矩给定"(w2687) -> ()
                n1387 = local write "加载电机左下转矩给定"(w2687) -> ()
                n1388 = local write "加载电机左上转矩给定"(w2687) -> ()
              }
              frame "R3" {
                n1389 = Multiply(x="R3扭矩给定", y=i16 -1) -> (x*y=w2690:i16)
                n1390 = local write "加载电机右上转矩给定"(w2690) -> ()
                n1391 = local write "加载电机右下转矩给定"(w2690) -> ()
                n1392 = local write "加载电机左下转矩给定"(w2690) -> ()
                n1393 = local write "加载电机左上转矩给定"(w2690) -> ()
              }
              frame "假", Default {
              }
            }
            n1394 = local read "启动布尔"() -> (w2662:bool)
            n1395 = case shown="真" w2662 {
              frame False {
              }
              frame True {
                n1396 = stacked-sequence {
                  frame #0 {
                    n1397 = property on="加载电机左上启动" class="Bool (严格)"("Val(Sgnl)"=TRUE ("值(信号)")) -> ()  [unwired: 2 in, 2 out]
                    n1398 = Wait (ms)(milliseconds to wait=u32 10 ("等待时间（毫秒）")) -> ()  [unwired: 1 out]
                  }
                  frame #1 {
                    n1399 = property on="加载电机左下启动" class="Bool (严格)"("Val(Sgnl)"=TRUE ("值(信号)")) -> ()  [unwired: 2 in, 2 out]
                    n1400 = Wait (ms)(milliseconds to wait=u32 10 ("等待时间（毫秒）")) -> ()  [unwired: 1 out]
                  }
                  frame #2 {
                    n1401 = property on="加载电机右上启动" class="Bool (严格)"("Val(Sgnl)"=TRUE ("值(信号)")) -> ()  [unwired: 2 in, 2 out]
                    n1402 = Wait (ms)(milliseconds to wait=u32 10 ("等待时间（毫秒）")) -> ()  [unwired: 1 out]
                  }
                  frame #3 {
                    n1403 = property on="加载电机右下启动" class="Bool (严格)"("Val(Sgnl)"=TRUE ("值(信号)")) -> ()  [unwired: 2 in, 2 out]
                    n1404 = Wait (ms)(milliseconds to wait=u32 10 ("等待时间（毫秒）")) -> ()  [unwired: 1 out]
                  }
                  frame #4 {
                    n1405 = property on="驱动电机上启动" class="Bool (严格)"("Val(Sgnl)"=TRUE ("值(信号)")) -> ()  [unwired: 2 in, 2 out]
                    n1406 = Wait (ms)(milliseconds to wait=u32 10 ("等待时间（毫秒）")) -> ()  [unwired: 1 out]
                  }
                  frame #5 {
                    n1407 = property on="驱动电机下启动" class="Bool (严格)"("Val(Sgnl)"=TRUE ("值(信号)")) -> ()  [unwired: 2 in, 2 out]
                    n1408 = Wait (ms)(milliseconds to wait=u32 10 ("等待时间（毫秒）")) -> ()  [unwired: 1 out]
                  }
                  frame #6 {
                    n1409 = local write "启动布尔"(FALSE ("启动布尔")) -> ()
                    n1410 = local write "停止布尔"(TRUE ("停止布尔")) -> ()
                  }
                }
              }
            }
          }
        }
        n1411 = case shown="\"N\"" w2638 {
          frame "假", Default {
          }
          frame "N" {
            n1412 = local read "停止布尔"() -> (w2649:bool)
            n1413 = case shown="真" w2649 {
              frame False {
              }
              frame True {
                n1414 = stacked-sequence {
                  frame #0 {
                    n1415 = local write "加载电机左上转矩给定"(i16 0 ("加载电机左上转矩给定")) -> ()
                    n1416 = Wait (ms)(milliseconds to wait=u32 10 ("等待时间（毫秒）")) -> ()  [unwired: 1 out]
                  }
                  frame #1 {
                    n1417 = local write "加载电机左下转矩给定"(i16 0 ("加载电机左下转矩给定")) -> ()
                    n1418 = Wait (ms)(milliseconds to wait=u32 10 ("等待时间（毫秒）")) -> ()  [unwired: 1 out]
                  }
                  frame #2 {
                    n1419 = local write "加载电机右上转矩给定"(i16 0 ("加载电机右上转矩给定")) -> ()
                    n1420 = Wait (ms)(milliseconds to wait=u32 10 ("等待时间（毫秒）")) -> ()  [unwired: 1 out]
                  }
                  frame #3 {
                    n1421 = local write "加载电机右下转矩给定"(i16 0 ("加载电机右下转矩给定")) -> ()
                    n1422 = Wait (ms)(milliseconds to wait=u32 10 ("等待时间（毫秒）")) -> ()  [unwired: 1 out]
                  }
                  frame #4 {
                    n1423 = Wait (ms)(milliseconds to wait=u32 10 ("等待时间（毫秒）")) -> ()  [unwired: 1 out]
                  }
                  frame #5 {
                    n1424 = Wait (ms)(milliseconds to wait=u32 10 ("等待时间（毫秒）")) -> ()  [unwired: 1 out]
                  }
                  frame #6 {
                    n1425 = local write "启动布尔"(TRUE ("启动布尔")) -> ()
                    n1426 = local write "停止布尔"(FALSE ("停止布尔")) -> ()
                  }
                }
              }
            }
          }
        }
        n1427 = local read "停止"() -> (w2640:bool)
        n1428 = Wait (ms)(milliseconds to wait=u32 50 ("等待时间（毫秒）")) -> ()  [unwired: 1 out]
      }
    }
  }
  n1429 = stacked-sequence {
    frame #0 {
      n1430 = stacked-sequence {
        frame #0 {
          w2695 = FALSE ("AD开始采集")
          n1431 = local write "AD开始采集"(w2695) -> ()
          n1432 = local write "PWM输出"(w2695) -> ()
          n1433 = local write "布尔"(FALSE ("布尔")) -> ()
          n1434 = local write "采集卡左"(FALSE ("采集卡左")) -> ()
          n1435 = local write "停止"(FALSE ("停止")) -> ()
          n1436 = local write "close"(FALSE ("close")) -> ()
        }
        frame #1 {
          n1437 = flat-sequence {
            tunnel: [w2708] -> w2705
            tunnel: [w2707] -> w2704
            tunnel: w2705 -> [w2713]
            tunnel: w2704 -> [w2712]
            tunnel: [w2711] -> w2703
            tunnel: [w2710] -> w2702
            tunnel: w2703 -> [w2720]
            tunnel: w2702 -> [w2719]
            tunnel: [w2718] -> w2701
            tunnel: [w2717] -> w2700
            tunnel: w2701 -> [w2726]
            tunnel: w2700 -> [w2725]
            tunnel: [w2724] -> w2699
            tunnel: [w2723] -> w2698
            tunnel: w2699 -> [w2730]
            tunnel: w2698 -> [w2729]
            frame #0 {
              n1438 = call "建立设备.vi"() -> ("错误输出"=w2707:errorcluster, "设备句柄"=w2708:i32)  [unwired: 10 in]
              n1439 = Wait (ms)(milliseconds to wait=u32 10 ("等待时间（毫秒）")) -> ()  [unwired: 1 out]
            }
            frame #1 {
              n1440 = Wait (ms)(milliseconds to wait=u32 10 ("等待时间（毫秒）")) -> ()  [unwired: 1 out]
              n1441 = call "建立命令连接.vi"("IP地址"="IP地址", "错误输入"=w2712, "端口号"="命令端口", "设备句柄入"=w2713) -> ("错误输出"=w2710:errorcluster, "设备句柄"=w2711:i32)  [unwired: 6 in]
            }
            frame #2 {
              n1442 = Wait (ms)(milliseconds to wait=u32 10 ("等待时间（毫秒）")) -> ()  [unwired: 1 out]
              n1443 = call "建立数据连接.vi"("错误输入"=w2719, "端口号"="数据端口", "设备句柄入"=w2720) -> ("错误输出"=w2717:errorcluster, "设备句柄"=w2718:i32)  [unwired: 7 in]
            }
            frame #3 {
              n1444 = local write "设置开关量方向"(cluster{"IO1~IO8":i8, "IO9~IO16":i8} {"IO1~IO8"=1, "IO9~IO16"=1} ("设置开关量方向")) -> ()
              n1445 = call "设置开关量方向.vi"("错误输入"=w2725, "方向"=i8[] [1, 1, 1, 1], "设备句柄入"=w2726) -> ("错误输出"=w2723:errorcluster, "设备句柄"=w2724:i32)  [unwired: 7 in]
              n1446 = Wait (ms)(milliseconds to wait=u32 10 ("等待时间（毫秒）")) -> ()  [unwired: 1 out]
            }
            frame #4 {
              n1447 = local write "错误输出"(w2729) -> ()
              "设备句柄" <- w2730
            }
          }
        }
        frame #2 {
        }
      }
    }
    frame #1 {
      n1448 = local read "错误输出"() -> (w2731:errorcluster)
      n1449 = while {
        shift-right: [w2733] -> _
        shift-left: w2731 -> [w2734]
        stop <- w2736 stop-if-true
        n1450 = local read "设备句柄"() -> (w2732:i32)
        n1451 = event shown="[1] 菜单选择(用户)" {
          selector: _ -> [_ _ _ _ _ _ _ _ _ _ _ _ _ _]
          dyn-events: _ -> [_ _ _ _ _ _ _ _ _ _ _ _ _ _]
          timeout: 100 -> [_ _ _ _ _ _ _ _ _ _ _ _ _ _]
          tunnel: w2732 -> [w2756 w2788 w2830 w2835 w2851 w2884 w2906 w2911 w2921 w2942 w2957 _ w2975 w2980]
          tunnel: w2734 -> [w2755 w2787 w2832 w2834 w2850 w2883 w2905 w2910 w2920 w2941 w2956 w2960 w2974 w2979]
          tunnel: [w2740 w2786 w2831 w2833 w2849 w2859 w2898 w2909 w2919 w2923 w2951 w2960 w2973 w2977] -> w2733
          event Timeout {
            n1452 = event-data() -> ()  [unwired: 1 in, 2 out]
            n1453 = call "得到所有通道开关量值.vi"("错误输入"=w2755, "设备句柄入"=w2756) -> ("错误输出"=w2738:errorcluster, "iStatus"=w2747:i8[], "设备句柄"=w2752:i32)  [unwired: 7 in]
            "错误输出 3" <- w2738
            n1454 = Array Subset(array=w2747, index=0 ("索引"), length=16 ("长度")) -> (w2744:i8[])
            n1455 = for {
              tunnel: w2744 -> [w2776] mode=indexing
              tunnel: [w2773] -> w2743 mode=indexing
              n1456 = Equal?(x=w2776, y=i8 1) -> (x = y?=w2774:bool)
              n1457 = case shown="假" w2774 {
                tunnel: [FALSE TRUE] -> w2773
                frame False {
                }
                frame True {
                }
              }
            }
            n1458 = Array Subset(array=w2747, index=16 ("索引"), length=8 ("长度")) -> (w2746:i8[])
            n1459 = for {
              tunnel: [w2780] -> w2745 mode=indexing
              tunnel: w2746 -> [w2779] mode=indexing
              n1460 = Equal?(x=w2779, y=i8 1) -> (x = y?=w2781:bool)
              n1461 = case shown="假" w2781 {
                tunnel: [FALSE TRUE] -> w2780
                frame False {
                }
                frame True {
                }
              }
            }
            "光隔离输入" <- w2745
            n1462 = Array To Cluster(array=w2743) -> (cluster=→"可编程数字量I/O(映射控件)--得到所有通道开关量值":T22)
            n1463 = call "读取编码器.vi"("错误输入"=w2738, "设备句柄入"=w2752) -> ("错误输出"=w2742:errorcluster, "编码器过零值"=→"编码器过零值":i16[], "编码器AB值"=→"编码器AB值":i32[], "设备句柄"=w2741:i32)  [unwired: 6 in]
            n1464 = local read "开启计数"() -> (w2739:bool)
            n1465 = case shown="真" w2739 {
              tunnel: w2742 -> [w2757 w2765]
              tunnel: w2741 -> [_ w2764]
              tunnel: [w2757 w2763] -> w2740
              frame False {
              }
              frame True {
                n1466 = call "读取所有路计数器的原码值.vi"("错误输入"=w2765, "设备句柄入"=w2764) -> ("错误输出"=w2761:errorcluster, "计数器的原码值"=w2758:u32[], "设备句柄"=w2762:i32)  [unwired: 7 in]
                n1467 = for {
                  N: 6 -> [_]
                  tunnel: w2762 -> [w2772]
                  tunnel: w2761 -> [w2771]
                  tunnel: [w2770] -> w2763
                  tunnel: [w2767] -> w2759 mode=indexing
                  tunnel: w2758 -> [w2766] mode=indexing
                  i -> [w2769]
                  n1468 = Increment(x=w2769) -> (x+1=w2768:i32)
                  n1469 = call "计数器值转换成对应的物理值.vi"("错误输入"=w2771, "ctCode"=w2766, "chNo"=w2768, "设备句柄入"=w2772) -> ("错误输出"=w2770:errorcluster, "ctValue"=w2767:dbl)  [unwired: 5 in, 1 out]
                }
                "计数/测频（Hz）值" <- w2759
              }
            }
          }
          event Menu Selection (User) {
            n1470 = event-data() -> ("ItemTag"=w2785:string)  [unwired: 1 in, 6 out]
            n1471 = case shown="\"采集卡左\"" w2785 {
              tunnel: w2788 -> [_ w2791]
              tunnel: w2787 -> [_ w2790]
              tunnel: [_ w2789] -> w2786
              frame "假", Default {
              }
              frame "采集卡左" {
                n1472 = flat-sequence {
                  tunnel: w2791 -> [w2795]
                  tunnel: w2790 -> [w2794]
                  tunnel: [w2793] -> w2792
                  tunnel: [w2829] -> w2789
                  tunnel: w2792 -> [w2829]
                  frame #0 {
                    n1473 = call "AD设置范围.vi"("错误输入"=w2794, "范围"="AD范围", "设备句柄入"=w2795) -> ("错误输出"=w2816:errorcluster, "设备句柄"=w2815:i32)  [unwired: 7 in]
                    n1474 = call "AD设置单双端.vi"("错误输入"=w2816, "单双端"="单双端", "设备句柄入"=w2815) -> ("错误输出"=w2818:errorcluster, "设备句柄"=w2817:i32)  [unwired: 7 in]
                    n1475 = call "AD设置增益.vi"("错误输入"=w2818, "增益"="增益", "设备句柄入"=w2817) -> ("错误输出"=w2825:errorcluster, "设备句柄"=w2824:i32)  [unwired: 7 in]
                    n1476 = call "AD设置通道范围.vi"("错误输入"=w2825, "起始通道"="AD起始通道", "终止通道"="AD终止通道", "设备句柄入"=w2824) -> ("错误输出"=w2819:errorcluster, "设备句柄"=w2820:i32)  [unwired: 6 in]
                    n1477 = Subtract(x="AD终止通道", y="AD起始通道") -> (x-y=w2803:i32)
                    n1478 = Increment(x=w2803) -> (x+1=w2821:i32)
                    "通道数量" <- w2821
                    n1479 = call "设定通道频率.vi"("错误输入"=w2819, "通道频率"="通道频率Hz", "设备句柄入"=w2820) -> ("错误输出"=w2807:errorcluster, "设备句柄"=w2806:i32)  [unwired: 7 in]
                    n1480 = local read "伪同步"() -> (w2812:i32)
                    n1481 = case shown="0, 默认" w2812 {
                      tunnel: "通道频率Hz" -> [w2826 _]
                      tunnel: [w2826 w2827] -> w2798
                      tunnel: "组频率Hz" -> [_ w2827]
                      frame 0, Default {
                      }
                      frame 1 {
                      }
                    }
                    n1482 = call "设定组频率.vi"("错误输入"=w2807, "组频率"="组频率Hz", "设备句柄入"=w2806) -> ("错误输出"=w2823:errorcluster, "设备句柄"=w2822:i32)  [unwired: 7 in]
                    n1483 = Divide(x=w2798, y=2.0 ("每秒刷新数据次数")) -> (x/y=w2796:dbl)
                    n1484 = To Long Integer(number=w2796) -> (32bit integer=w2801:i32)
                    n1485 = Quotient & Remainder(x=w2801, y=w2821) -> (floor(x/y)=w2800:i32)  [unwired: 1 out]
                    "每通道数据量" <- w2800
                    n1486 = Multiply(x=w2800, y=w2821) -> (x*y=→"每次总数据量":i32)
                    n1487 = call "启动采集(M系列).vi"("错误输入"=w2823, "时钟源"="时钟源", "伪同步"="伪同步", "设备句柄入"=w2822) -> ("错误输出"=w2793:errorcluster)  [unwired: 6 in, 1 out]
                  }
                  frame #1 {
                    n1488 = local write "布尔"(TRUE ("布尔")) -> ()
                  }
                }
              }
            }
          }
          event "AD停止采集": Value Change {
            n1489 = event-data() -> ()  [unwired: 1 in, 5 out]
            n1490 = call "停止采集(M).vi"("错误输入"=w2832, "设备句柄入"=w2830) -> ("错误输出"=w2831:errorcluster)  [unwired: 8 in, 1 out]
          }
          event "开启计数": Value Change {
            n1491 = event-data() -> ()  [unwired: 1 in, 5 out]
            n1492 = Initialize Array("工作方式", 6 ("维数大小")) -> (w2839:u16[])
            n1493 = call "设置所有路计数器的工作方式.vi"("错误输入"=w2834, "ctMode"=w2839, "设备句柄入"=w2835) -> ("错误输出"=w2838:errorcluster, "设备句柄"=w2837:i32)  [unwired: 7 in]
            n1494 = for {
              N: 6 -> [_]
              tunnel: w2838 -> [w2847]
              tunnel: w2837 -> [w2846]
              tunnel: [w2842] -> w2833
              i -> [w2844]
              n1495 = Increment(x=w2844) -> (x+1=w2843:i32)
              n1496 = call "设置指定通道的测频基准脉冲周期.vi"("错误输入"=w2847, "freqBase_ms"=1000.0, "chNo"=w2843, "设备句柄入"=w2846) -> ("错误输出"=w2842:errorcluster)  [unwired: 5 in, 2 out]
            }
          }
          event "计数器清零": Value Change {
            n1497 = event-data() -> ()  [unwired: 1 in, 5 out]
            n1498 = for {
              N: 6 -> [_]
              tunnel: w2851 -> [w2856]
              tunnel: w2850 -> [w2855]
              tunnel: [w2854] -> w2849
              i -> [w2853]
              n1499 = Increment(x=w2853) -> (x+1=w2852:i32)
              n1500 = call "指定通道计数器清零.vi"("错误输入"=w2855, "chNo"=w2852, "设备句柄入"=w2856) -> ("错误输出"=w2854:errorcluster)  [unwired: 7 in, 1 out]
            }
          }
          event "PWM输出": Value Change {
            n1501 = event-data() -> ("OldVal"=w2857:bool)  [unwired: 1 in, 4 out]
            n1502 = local write "PWM输出"(w2857) -> ()
            n1503 = call "设置开关量方向.vi"("错误输入"=w2883, "方向"=i8[] [1, 1], "设备句柄入"=w2884) -> ("错误输出"=w2881:errorcluster, "设备句柄"=w2882:i32)  [unwired: 7 in]
            n1504 = call "设置PWM频率和占空比.vi"("占空比(0~1)"="占空比(0~1)", "频率"="频率1", "错误输入"=w2881, "通道号"=1, "设备句柄入"=w2882) -> ("错误输出"=w2873:errorcluster, "设备句柄"=w2867:i32, "实际占空比"=→"实际占空比":dbl, "实际频率"=→"实际频率":dbl)  [unwired: 3 in]
            n1505 = call "设置PWM频率和占空比.vi"("占空比(0~1)"="占空比(0~1) 2", "频率"="频率2", "错误输入"=w2873, "通道号"=2, "设备句柄入"=w2867) -> ("错误输出"=w2866:errorcluster, "设备句柄"=w2868:i32, "实际占空比"=→"实际占空比 2":dbl, "实际频率"=→"实际频率 2":dbl)  [unwired: 3 in]
            n1506 = call "设置PWM频率和占空比.vi"("占空比(0~1)"="占空比(0~1) 3", "频率"="频率3", "错误输入"=w2866, "通道号"=3, "设备句柄入"=w2868) -> ("错误输出"=w2860:errorcluster, "设备句柄"=w2861:i32, "实际占空比"=→"实际占空比 3":dbl, "实际频率"=→"实际频率 3":dbl)  [unwired: 3 in]
            n1507 = call "使能或禁止PWM输出.vi"("错误输入"=w2860, "所用PWM使能"=i8 1, "设备句柄入"=w2861) -> ("错误输出"=w2859:errorcluster)  [unwired: 7 in, 1 out]
          }
          event "M系列PWM输出": Value Change {
            w2893 = 2 ("通道号")
            w2888 = 0.5 ("占空比(0~1)")
            w2889 = 2000.0 ("频率")
            w2901 = 1 ("通道号")
            n1508 = event-data() -> ()  [unwired: 1 in, 5 out]
            n1509 = call "设置开关量方向.vi"("错误输入"=w2905, "方向"=i8[] [1, 1], "设备句柄入"=w2906) -> ("错误输出"=w2903:errorcluster, "设备句柄"=w2904:i32)  [unwired: 7 in]
            n1510 = call "设置PWM频率和占空比.vi"("占空比(0~1)"=w2888, "频率"=w2889, "错误输入"=w2903, "通道号"=w2901, "设备句柄入"=w2904) -> ("错误输出"=w2899:errorcluster, "设备句柄"=w2902:i32)  [unwired: 3 in, 2 out]
            n1511 = call "设定输出脉冲个数.vi"("错误输入"=w2899, "脉冲个数"="设定输出脉冲个数", "通道号"=w2901, "设备句柄入"=w2902) -> ("错误输出"=w2891:errorcluster, "设备句柄"=w2890:i32)  [unwired: 2 in]
            n1512 = call "设置PWM频率和占空比.vi"("占空比(0~1)"=w2888, "频率"=w2889, "错误输入"=w2891, "通道号"=w2893, "设备句柄入"=w2890) -> ("错误输出"=w2892:errorcluster, "设备句柄"=w2894:i32)  [unwired: 3 in, 2 out]
            n1513 = call "设定输出脉冲个数.vi"("错误输入"=w2892, "通道号"=w2893, "设备句柄入"=w2894) -> ("错误输出"=w2886:errorcluster, "设备句柄"=w2887:i32)  [unwired: 3 in]
            n1514 = call "使能或禁止PWM输出(只支持EM9636M).vi"("错误输入"=w2886, "相位设置数组"=i8[] [1, 0, 0] ("PWM使能"), "PWM使能"=i8[] [1, 1, 0], "设备句柄入"=w2887) -> ("错误输出"=w2898:errorcluster)  [unwired: 6 in, 1 out]
          }
          event "设置开关量方向": Value Change {
            n1515 = event-data() -> ()  [unwired: 1 in, 5 out]
            n1516 = Cluster To Array(cluster="设置开关量方向") -> (array=w2907:i8[])
            "数组 4" <- w2907
            n1517 = call "设置开关量方向.vi"("错误输入"=w2910, "方向"=w2907, "设备句柄入"=w2911) -> ("错误输出"=w2909:errorcluster)  [unwired: 7 in, 1 out]
          }
          event "光隔离输出", "可编程数字量I/O": Value Change {
            n1518 = event-data() -> ()  [unwired: 1 in, 5 out]
            n1519 = local read "光隔离输入"() -> (w2918:bool[])
            n1520 = Cluster To Array(cluster="可编程数字量I/O") -> (array=w2912:bool[])
            n1521 = Build Array (concatenate)(w2912, w2918, "光隔离输出") -> (w2916:bool[])
            n1522 = Boolean To (0,1)(Boolean=w2916) -> (0, 1=w2915:i16[])
            n1523 = To Byte Integer(number=w2915) -> (8bit integer=w2914:i8[])
            n1524 = call "设置所有通道开关量值.vi"("错误输入"=w2920, "oStatus"=w2914, "设备句柄入"=w2921) -> ("错误输出"=w2919:errorcluster)  [unwired: 7 in, 1 out]
          }
          event "DA输出", "CH1", "CH2", "CH3", "CH4": Value Change {
            n1525 = event-data() -> ()  [unwired: 1 in, 5 out]
            n1526 = for {
              N: 4 -> [_]
              tunnel: w2942 -> [w2950]
              tunnel: w2941 -> [w2949]
              tunnel: "DA输出范围" -> [w2945]
              tunnel: [w2944] -> w2939
              tunnel: [w2943] -> w2938
              i -> [w2947]
              n1527 = Increment(x=w2947) -> (x+1=w2948:i32)
              n1528 = call "DA输出方式.vi"("输出范围"=w2945, "错误输入"=w2949, "输出值方式"=i16 1, "通道号"=w2948, "设备句柄入"=w2950) -> ("错误输出"=w2944:errorcluster, "设备句柄"=w2943:i32)  [unwired: 5 in]
            }
            n1529 = call "设置DA输出值.vi"("错误输入"=w2939, "输出值"="CH1", "通道号"=1, "设备句柄入"=w2938) -> ("错误输出"=w2932:errorcluster, "设备句柄"=w2934:i32)  [unwired: 6 in]
            n1530 = call "设置DA输出值.vi"("错误输入"=w2932, "输出值"="CH2", "通道号"=2, "设备句柄入"=w2934) -> ("错误输出"=w2926:errorcluster, "设备句柄"=w2931:i32)  [unwired: 6 in]
            n1531 = call "设置DA输出值.vi"("错误输入"=w2926, "输出值"="CH3", "通道号"=3, "设备句柄入"=w2931) -> ("错误输出"=w2925:errorcluster, "设备句柄"=w2930:i32)  [unwired: 6 in]
            n1532 = call "设置DA输出值.vi"("错误输入"=w2925, "输出值"="CH4", "通道号"=4, "设备句柄入"=w2930) -> ("错误输出"=w2923:errorcluster)  [unwired: 6 in, 1 out]
          }
          event "编码器清零": Value Change {
            n1533 = event-data() -> ()  [unwired: 1 in, 5 out]
            n1534 = call "编码器清零.vi"("错误输入"=w2956, "通道号"=1, "设备句柄入"=w2957) -> ("错误输出"=w2952:errorcluster, "设备句柄"=w2953:i32)  [unwired: 7 in]
            n1535 = call "编码器清零.vi"("错误输入"=w2952, "通道号"=2, "设备句柄入"=w2953) -> ("错误输出"=w2951:errorcluster)  [unwired: 7 in, 1 out]
          }
          event "DA输出范围": Value Change {
            n1536 = event-data() -> ()  [unwired: 1 in, 5 out]
            n1537 = local read "DA输出范围"() -> (w2961:i32)
            n1538 = case shown="4" w2961 {
              tunnel: [10000.0 ("标尺.范围:最大值") 5000.0 ("标尺.范围:最大值") 10000.0 ("标尺.范围:最大值") 5000.0 ("标尺.范围:最大值") 20000.0 ("标尺.范围:最大值")] -> w2959
              tunnel: [-10000.0 ("标尺.范围:最大值") -5000.0 ("标尺.范围:最大值") 0.0 ("标尺.范围:最大值") 0.0 ("标尺.范围:最大值") 0.0 ("标尺.范围:最大值")] -> w2958
              frame 0, Default {
              }
              frame 1 {
              }
              frame 2 {
              }
              frame 3 {
              }
              frame 4 {
              }
            }
            n1539 = property on="CH1" class="Slide (严格)"("Scale.Maximum"=w2959, "Scale.Minimum"=w2958) -> ()  [unwired: 2 in, 2 out]
            n1540 = property on="CH2" class="Slide (严格)"("Scale.Maximum"=w2959, "Scale.Minimum"=w2958) -> ()  [unwired: 2 in, 2 out]
            n1541 = property on="CH3" class="Slide (严格)"("Scale.Maximum"=w2959, "Scale.Minimum"=w2958) -> ()  [unwired: 2 in, 2 out]
            n1542 = property on="CH4" class="Slide (严格)"("Scale.Maximum"=w2959, "Scale.Minimum"=w2958) -> ()  [unwired: 2 in, 2 out]
          }
          event "M系列PWM停止": Value Change {
            n1543 = event-data() -> ()  [unwired: 1 in, 5 out]
            n1544 = call "使能或禁止PWM输出(只支持EM9636M).vi"("错误输入"=w2974, "相位设置数组"=i8[] [0, 0, 0] ("PWM使能"), "PWM使能"=i8[] [0, 0, 0], "设备句柄入"=w2975) -> ("错误输出"=w2973:errorcluster)  [unwired: 6 in, 1 out]
          }
          event "PWM停止": Value Change {
            n1545 = event-data() -> ()  [unwired: 1 in, 5 out]
            n1546 = call "使能或禁止PWM输出.vi"("错误输入"=w2979, "所用PWM使能"=i8 0, "设备句柄入"=w2980) -> ("错误输出"=w2977:errorcluster)  [unwired: 7 in, 1 out]
          }
        }
        "错误输出 2" <- w2733
        n1547 = local read "停止"() -> (w2736:bool)
      }
      n1548 = while {
        stop <- "停止" stop-if-true
        n1549 = local read "布尔"() -> (w2983:bool)
        n1550 = Wait (ms)(milliseconds to wait=u32 10 ("等待时间（毫秒）")) -> ()  [unwired: 1 out]
        n1551 = case shown="真" w2983 {
          frame False {
          }
          frame True {
            n1552 = local read "设备句柄"() -> (w2994:i32)
            n1553 = local read "每次总数据量"() -> (w2992:i32)
            n1554 = call "得到上位机软件缓冲区数据个数(M).vi"("设备句柄入"=w2994) -> ("错误输出"=w2990:errorcluster, "可读数据个数"=w2993:i32, "设备句柄"=w2991:i32)  [unwired: 8 in]
            n1555 = call <vilib>:"Clear Errors.vi"("error in (no error)"=w2990) -> ()  [unwired: 5 in, 2 out]
            n1556 = Not(x=w2990) -> (.not. x?=→"采集卡左":bool)
            n1557 = Greater Or Equal?(x=w2993, y=w2992) -> (x >= y?=w2989:bool)
            n1558 = case shown="真" w2989 {
              tunnel: w2992 -> [_ w3006]
              tunnel: w2991 -> [_ w3005]
              frame False {
              }
              frame True {
                n1559 = call "读取高速数据(M).vi"("数据个数"=w3006, "设备句柄入"=w3005) -> ("错误输出"=w3012:errorcluster, "返回数据个数"=w3013:i32, "原码值"=w3014:u16[], "设备句柄"=w3015:i32)  [unwired: 6 in]
                "错误输出" <- w3012
                n1560 = local read "每次总数据量"() -> (w3010:i32)
                n1561 = local read "通道数量"() -> (w2999:i32)
                n1562 = Divide(x=w3010, y=w2999) -> (x/y=w3009:dbl)
                n1563 = call "AD原码转物理.vi"("设备句柄入"=w3015, "原码值"=w3014, "个数"=w3013, "错误输入"=w3012) -> ("物理值"=w3011:dbl[])  [unwired: 4 in, 2 out]
                n1564 = To Long Integer(number=w3009) -> (32bit integer=w3008:i32)
                n1565 = Reshape Array "重排数组维数"(w3011, w3008, w2999) -> (w3007:dbl[][])
                n1566 = Transpose 2D Array(2D array=w3007) -> (transposed array=w3003:dbl[][])
                n1567 = Array Size(array=w3003) -> (size(s)=w3002:i32[])
                n1568 = for {
                  tunnel: w3003 -> [w3017] mode=indexing
                  tunnel: [w3016] -> w3004 mode=indexing
                  n1569 = Add Array Elements(numeric array=w3017) -> (sum=w3016:dbl)
                }
                n1570 = Index Array(array=w3002, index=1 ("索引")) -> (element=w3000:i32)
                n1571 = Divide(x=w3004, y=w3000) -> (x/y=w2998:dbl[])
                "AD均值数据" <- w2998
                n1572 = Reshape Array(w2998, 4 ("维数大小"), 8 ("维数大小")) -> (→"输出数组左":dbl[][])
              }
            }
          }
        }
        n1573 = local read "设备句柄"() -> (w2981:i32)
        n1574 = case shown="真" "停止" {
          tunnel: w2981 -> [_ w2985]
          frame False {
          }
          frame True {
            n1575 = flat-sequence {
              tunnel: w2985 -> [w2986]
              frame #0 {
                n1576 = call "停止采集(M).vi"("设备句柄入"=w2986) -> ()  [unwired: 9 in, 2 out]
              }
              frame #1 {
                "布尔" <- FALSE ("布尔")
              }
            }
          }
        }
      }
    }
    frame #2 {
      n1577 = flat-sequence {
        tunnel: [w3028] -> w3024
        tunnel: [w3026] -> w3023
        tunnel: w3024 -> [w3034]
        tunnel: [w3033] -> w3022
        tunnel: w3023 -> [w3032]
        tunnel: [w3031] -> w3021
        tunnel: w3022 -> [w3040]
        tunnel: [w3039] -> w3020
        tunnel: w3021 -> [w3038]
        tunnel: [w3037] -> w3019
        tunnel: w3020 -> [w3045]
        tunnel: [w3044] -> w3018
        tunnel: w3019 -> [w3043]
        tunnel: w3018 -> [w3046]
        frame #0 {
          n1578 = local read "设备句柄"() -> (w3029:i32)
          n1579 = local read "错误输出"() -> (w3027:errorcluster)
          n1580 = call "停止采集(M).vi"("错误输入"=w3027, "设备句柄入"=w3029) -> ("错误输出"=w3026:errorcluster, "设备句柄"=w3028:i32)  [unwired: 8 in]
          n1581 = Wait (ms)(milliseconds to wait=u32 10 ("等待时间（毫秒）")) -> ()  [unwired: 1 out]
        }
        frame #1 {
          n1582 = call "使能或禁止PWM输出.vi"("错误输入"=w3032, "所用PWM使能"=i8 0, "设备句柄入"=w3034) -> ("错误输出"=w3031:errorcluster, "设备句柄"=w3033:i32)  [unwired: 7 in]
          n1583 = Wait (ms)(milliseconds to wait=u32 10 ("等待时间（毫秒）")) -> ()  [unwired: 1 out]
        }
        frame #2 {
          n1584 = call "关闭数据连接.vi"("错误输入"=w3038, "设备句柄入"=w3040) -> ("错误输出"=w3037:errorcluster, "设备句柄"=w3039:i32)  [unwired: 8 in]
          n1585 = Wait (ms)(milliseconds to wait=u32 10 ("等待时间（毫秒）")) -> ()  [unwired: 1 out]
        }
        frame #3 {
          n1586 = call "关闭命令连接.vi"("错误输入"=w3043, "设备句柄入"=w3045) -> ("错误输出"=w3042:errorcluster, "设备句柄"=w3044:i32)  [unwired: 8 in]
          n1587 = Wait (ms)(milliseconds to wait=u32 10 ("等待时间（毫秒）")) -> ()  [unwired: 1 out]
          n1588 = local write "错误输出"(w3042) -> ()
        }
        frame #4 {
          n1589 = call "关闭设备.vi"("设备句柄"=w3046) -> ()  [unwired: 10 in]
        }
        frame #5 {
          "close" <- TRUE ("close")
        }
      }
    }
  }
  n1590 = while {
    stop <- w3138 stop-if-true
    # "原本以为返回的是百分比，要\n重新标定"
    # "4"
    # "3"
    # "2"
    # "1"
    # "档位"
    # "功率"
    # "扭矩"
    # "车速"
    n1591 = local read "加载功率"() -> (w3093:dbl)
    n1592 = call "asc转换.vi"("输入数据"=w3093) -> ("数值位 5"=w3104:u8, "数值位 4"=w3105:u8, "数值位 3"=w3106:u8, "数值位 2"=w3107:u8)  [unwired: 7 in]
    n1593 = local write "0byte 5"(u8 80 ("6byte 3")) -> ()
    n1594 = local write "1byte 5"(u8 6 ("7byte 3")) -> ()
    n1595 = local write "2byte 5"(u8 32 ("7byte 3")) -> ()
    n1596 = local write "3byte 5"(w3107) -> ()
    n1597 = local write "4byte 5"(w3106) -> ()
    n1598 = local write "5byte 5"(w3105) -> ()
    n1599 = local write "6byte 5"(w3104) -> ()
    n1600 = local write "7byte 5"(u8 32 ("7byte 3")) -> ()
    n1601 = local write "0byte"(u8 16 ("6byte 3")) -> ()
    n1602 = local write "1byte"(u8 6 ("7byte 3")) -> ()
    n1603 = local write "2byte"("左1字符") -> ()
    n1604 = local write "3byte"("左2字符") -> ()
    n1605 = local write "4byte"("左3字符") -> ()
    n1606 = local write "5byte"("左4字符") -> ()
    n1607 = local write "6byte"("左5字符") -> ()
    n1608 = local write "7byte"(u8 32 ("7byte 3")) -> ()
    n1609 = local read "加载左上转速监控"() -> (w3094:dbl)
    n1610 = local read "加载左上转矩监控"() -> (w3119:i16)
    n1611 = Greater Or Equal?(x=w3094, y=0.0) -> (x >= y?=w3130:bool)
    n1612 = Absolute Value(x=w3094) -> (abs(x)=w3123:dbl)
    n1613 = Greater Or Equal?(x=w3119, y=0.0) -> (x >= y?=w3122:bool)
    n1614 = Absolute Value(x=w3119) -> (abs(x)=w3108:i16)
    n1615 = case shown="真" w3130 {
      tunnel: w3123 -> [w3203 w3205]
      tunnel: [w3203 w3205] -> w3125
      tunnel: [u8 45 ("6byte 3") u8 32 ("6byte 3")] -> w3124
      frame False {
      }
      frame True {
      }
    }
    n1616 = case shown="假" w3122 {
      tunnel: w3108 -> [w3199 w3201]
      tunnel: [w3199 w3201] -> w3120
      tunnel: [u8 45 ("6byte 3") u8 32 ("6byte 3")] -> w3114
      frame False {
      }
      frame True {
      }
    }
    n1617 = call <vilib>:"Boolean Crossing PtByPt.vi"("direction"=enum16{"either", "false-true", "true-false"}."false-true", "input"="加载电机复位") -> ("crossing"=w3068:bool)  [unwired: 1 in]
    n1618 = call "asc转换.vi"("输入数据"=w3125) -> ("数值位 5"=w3126:u8, "数值位 4"=w3127:u8, "数值位 3"=w3128:u8, "数值位 2"=w3129:u8)  [unwired: 7 in]
    n1619 = case shown="真" w3068 {
      frame False {
      }
      frame True {
        w3140 = TRUE
        n1620 = local write "变频6"(w3140) -> ()
        n1621 = local write "变频5"(w3140) -> ()
        n1622 = local write "变频4"(w3140) -> ()
        n1623 = local write "变频3"(w3140) -> ()
        n1624 = local write "变频2"(w3140) -> ()
        n1625 = local write "变频1"(w3140) -> ()
      }
    }
    n1626 = call "asc转换.vi"("输入数据"=w3120) -> ("数值位 5"=w3115:u8, "数值位 4"=w3116:u8, "数值位 3"=w3117:u8, "数值位 2"=w3118:u8)  [unwired: 7 in]
    n1627 = local write "0byte 3"(u8 48 ("6byte 3")) -> ()
    n1628 = local write "1byte 3"(u8 6 ("7byte 3")) -> ()
    n1629 = local write "2byte 3"(w3124) -> ()
    n1630 = local write "3byte 3"(w3129) -> ()
    n1631 = local write "4byte 3"(w3128) -> ()
    n1632 = local write "5byte 3"(w3127) -> ()
    n1633 = local write "6byte 3"(w3126) -> ()
    n1634 = local write "7byte 3"(u8 82 ("7byte 3")) -> ()
    n1635 = local write "0byte 7"(u8 112 ("6byte 3")) -> ()
    n1636 = local write "1byte 7"(u8 6 ("7byte 3")) -> ()
    n1637 = local write "2byte 7"(w3114) -> ()
    n1638 = local write "3byte 7"(w3118) -> ()
    n1639 = local write "4byte 7"(w3117) -> ()
    n1640 = local write "5byte 7"(w3116) -> ()
    n1641 = local write "6byte 7"(w3115) -> ()
    n1642 = local write "7byte 7"(u8 32 ("7byte 3")) -> ()
    n1643 = local read "加载右上转速监控"() -> (w3051:dbl)
    n1644 = local read "加载左上转速监控"() -> (w3050:dbl)
    n1645 = local read "加载转速右下监控"() -> (w3049:dbl)
    n1646 = local read "加载左下转速监控"() -> (w3048:dbl)
    n1647 = local read "加载转矩右上监控"() -> (w3081:i16)
    n1648 = local read "加载右下转矩监控"() -> (w3076:i16)
    n1649 = local read "加载左下转矩监控"() -> (w3075:i16)
    n1650 = local read "加载左上转矩监控"() -> (w3077:i16)
    n1651 = local read "加载左上转速监控"() -> (w3103:dbl)
    n1652 = Multiply(x=w3081, y=0.1) -> (x*y=w3067:dbl)
    n1653 = Multiply(x=w3077, y=0.1) -> (x*y=w3066:dbl)
    n1654 = Multiply(x=w3075, y=0.1) -> (x*y=w3064:dbl)
    n1655 = Multiply(x=w3076, y=0.1) -> (x*y=w3065:dbl)
    n1656 = Compound Arithmetic op=MULTIPLY(w3103, 0.52 ("值"), 3.141592653589793, 60.0 ("值")) -> (w3099:dbl)
    n1657 = Multiply(x=w3067, y=w3051) -> (x*y=w3060:dbl)
    n1658 = Multiply(x=w3066, y=w3050) -> (x*y=w3059:dbl)
    n1659 = Multiply(x=w3065, y=w3049) -> (x*y=w3058:dbl)
    n1660 = Multiply(x=w3064, y=w3048) -> (x*y=w3057:dbl)
    n1661 = local read "元素 4"() -> (w3083:bool)
    n1662 = Divide(x=w3099, y=1000.0) -> (x/y=w3073:dbl)
    n1663 = local read "布尔数组"() -> (w3096:bool[])
    n1664 = local write "遥控器按钮确认"(w3083) -> ()
    n1665 = Multiply(x=w3073, y=-1.0) -> (x*y=→"车速":dbl)
    n1666 = Divide(x=w3057, y=9550.0) -> (x/y=w3053:dbl)
    n1667 = Divide(x=w3060, y=9550.0) -> (x/y=w3056:dbl)
    n1668 = Divide(x=w3059, y=9550.0) -> (x/y=w3055:dbl)
    n1669 = Divide(x=w3058, y=9550.0) -> (x/y=w3054:dbl)
    n1670 = Index Array(array=w3096) -> (element #1=→"元素 3":bool, element #2=→"元素 4":bool, element #5=w3095:bool)  [unwired: 8 in, 5 out]
    n1671 = Compound Arithmetic op=ADD(w3056, w3055, w3054, w3053) -> (w3052:dbl)
    n1672 = Absolute Value(x=w3052) -> (abs(x)=→"加载功率":dbl)
    n1673 = case shown="假" w3095 {
      frame False {
        w3154 = u8 32 ("左1字符")
        n1674 = local read "布尔数组 2"() -> (w3167:bool[])
        n1675 = local read "布尔数组"() -> (w3168:bool[])
        n1676 = local write "左3字符"(w3154) -> ()
        n1677 = local write "左4字符"(w3154) -> ()
        n1678 = local write "左5字符"(w3154) -> ()
        n1679 = Index Array(array=w3167) -> (element #1=w3159:bool, element #2=w3158:bool, element #3=w3157:bool, element #4=w3156:bool)  [unwired: 8 in, 4 out]
        n1680 = Index Array(array=w3168) -> (element #2=→"元素":bool, element #3=→"元素 2":bool, element #4=w3166:bool, element #6=w3155:bool, element #7=w3165:bool, element #8=w3164:bool)  [unwired: 8 in, 2 out]
        n1681 = And(x=w3155, y=w3159) -> (x .and. y?=w3146:bool)
        n1682 = And(x=w3155, y=w3164) -> (x .and. y?=w3145:bool)
        n1683 = And(x=w3155, y=w3165) -> (x .and. y?=w3144:bool)
        n1684 = Compound Arithmetic op=OR ("复合运算")(w3144, w3145, w3146) -> (w3143:bool)
        n1685 = case shown="真" w3143 {
          frame False {
          }
          frame True {
            n1686 = local write "左1字符"(u8 82 ("左1字符")) -> ()
          }
        }
        n1687 = And(x=w3155, y=w3158) -> (x .and. y?=w3162:bool)
        n1688 = And(x=w3155, y=w3157) -> (x .and. y?=w3161:bool)
        n1689 = And(x=w3155, y=w3156) -> (x .and. y?=w3160:bool)
        n1690 = And(x=w3166, y=w3165) -> (x .and. y?=w3153:bool)
        n1691 = And(x=w3166, y=w3164) -> (x .and. y?=w3152:bool)
        n1692 = And(x=w3166, y=w3159) -> (x .and. y?=w3151:bool)
        n1693 = And(x=w3166, y=w3158) -> (x .and. y?=w3150:bool)
        n1694 = And(x=w3166, y=w3157) -> (x .and. y?=w3149:bool)
        n1695 = And(x=w3166, y=w3156) -> (x .and. y?=w3148:bool)
        n1696 = Compound Arithmetic op=OR ("复合运算")(w3153, w3152, w3151, w3150, w3149, w3148) -> (w3147:bool)
        n1697 = case shown="假" w3147 {
          frame False {
          }
          frame True {
            n1698 = local write "左1字符"(u8 68 ("左1字符")) -> ()
          }
        }
        n1699 = Compound Arithmetic op=OR ("复合运算")(w3162, w3161, w3160) -> (w3163:bool)
        n1700 = case shown="真" w3163 {
          frame False {
          }
          frame True {
            n1701 = local write "左1字符"(u8 69 ("左1字符")) -> ()
            n1702 = local write "左2字符"(u8 82 ("左1字符")) -> ()
            n1703 = local write "左3字符"(u8 82 ("左1字符")) -> ()
            n1704 = local write "左4字符"(u8 79 ("左1字符")) -> ()
            n1705 = local write "左5字符"(u8 82 ("左1字符")) -> ()
            n1706 = local write "当前试验档位"("无效档" ("当前试验档位")) -> ()
          }
        }
        n1707 = case shown="真" w3146 {
          frame False {
          }
          frame True {
            n1708 = local write "当前试验档位"("R3" ("当前试验档位")) -> ()
            n1709 = local write "左2字符"(u8 51 ("左1字符")) -> ()
          }
        }
        n1710 = case shown="真" w3145 {
          frame False {
          }
          frame True {
            n1711 = local write "当前试验档位"("R2" ("当前试验档位")) -> ()
            n1712 = local write "左2字符"(u8 50 ("左1字符")) -> ()
          }
        }
        n1713 = case shown="真" w3149 {
          frame False {
          }
          frame True {
            n1714 = local write "当前试验档位"("D5" ("当前试验档位")) -> ()
            n1715 = local write "左2字符"(u8 53 ("左1字符")) -> ()
          }
        }
        n1716 = case shown="真" w3150 {
          frame False {
          }
          frame True {
            n1717 = local write "当前试验档位"("D4" ("当前试验档位")) -> ()
            n1718 = local write "左2字符"(u8 52 ("左1字符")) -> ()
          }
        }
        n1719 = case shown="真" w3144 {
          frame False {
          }
          frame True {
            n1720 = local write "当前试验档位"("R1" ("当前试验档位")) -> ()
            n1721 = local write "左2字符"(u8 49 ("左1字符")) -> ()
          }
        }
        n1722 = case shown="真" w3153 {
          frame False {
          }
          frame True {
            n1723 = local write "当前试验档位"("D1" ("当前试验档位")) -> ()
            n1724 = local write "左2字符"(u8 49 ("左1字符")) -> ()
          }
        }
        n1725 = case shown="真" w3151 {
          frame False {
          }
          frame True {
            n1726 = local write "当前试验档位"("D3" ("当前试验档位")) -> ()
            n1727 = local write "左2字符"(u8 51 ("左1字符")) -> ()
          }
        }
        n1728 = case shown="真" w3148 {
          frame False {
          }
          frame True {
            n1729 = local write "当前试验档位"("D6" ("当前试验档位")) -> ()
            n1730 = local write "左2字符"(u8 54 ("左1字符")) -> ()
          }
        }
        n1731 = case shown="真" w3152 {
          frame False {
          }
          frame True {
            n1732 = local write "当前试验档位"("D2" ("当前试验档位")) -> ()
            n1733 = local write "左2字符"(u8 50 ("左1字符")) -> ()
          }
        }
      }
      frame True {
        w3195 = u8 32 ("左1字符")
        n1734 = local write "当前试验档位"("N" ("当前试验档位")) -> ()
        n1735 = local write "左2字符"(w3195) -> ()
        n1736 = local write "左3字符"(w3195) -> ()
        n1737 = local write "左4字符"(w3195) -> ()
        n1738 = local write "左5字符"(w3195) -> ()
        n1739 = local write "左1字符"(u8 78 ("左1字符")) -> ()
      }
    }
    n1740 = local read "停止"() -> (w3138:bool)
    n1741 = Wait (ms)(milliseconds to wait=u32 50 ("等待时间（毫秒）")) -> ()  [unwired: 1 out]
  }
  n1742 = stacked-sequence {
    frame #0 {
      n1743 = stacked-sequence {
        frame #0 {
          w3209 = FALSE ("AD开始采集")
          n1744 = local write "AD开始采集 2"(w3209) -> ()
          n1745 = local write "PWM输出 2"(w3209) -> ()
          n1746 = local write "布尔 2"(FALSE ("布尔")) -> ()
          n1747 = local write "采集卡右"(FALSE ("采集卡右")) -> ()
          n1748 = local write "停止"(FALSE ("停止")) -> ()
          n1749 = local write "close2"(FALSE ("close2")) -> ()
        }
        frame #1 {
          n1750 = flat-sequence {
            tunnel: [w3221] -> w3218
            tunnel: [w3220] -> w3217
            tunnel: w3218 -> [w3226]
            tunnel: w3217 -> [w3225]
            tunnel: [w3224] -> w3216
            tunnel: [w3223] -> w3215
            tunnel: w3216 -> [w3233]
            tunnel: w3215 -> [w3232]
            tunnel: [w3231] -> w3214
            tunnel: [w3230] -> w3213
            tunnel: w3214 -> [w3239]
            tunnel: w3213 -> [w3238]
            tunnel: [w3237] -> w3212
            tunnel: [w3236] -> w3211
            tunnel: w3212 -> [w3243]
            tunnel: w3211 -> [w3242]
            frame #0 {
              n1751 = call "建立设备.vi"() -> ("错误输出"=w3220:errorcluster, "设备句柄"=w3221:i32)  [unwired: 10 in]
              n1752 = Wait (ms)(milliseconds to wait=u32 10 ("等待时间（毫秒）")) -> ()  [unwired: 1 out]
            }
            frame #1 {
              n1753 = Wait (ms)(milliseconds to wait=u32 10 ("等待时间（毫秒）")) -> ()  [unwired: 1 out]
              n1754 = call "建立命令连接.vi"("IP地址"="192.168.1.126" ("IP地址 2"), "错误输入"=w3225, "端口号"=8000 ("命令端口 2"), "设备句柄入"=w3226) -> ("错误输出"=w3223:errorcluster, "设备句柄"=w3224:i32)  [unwired: 6 in]
            }
            frame #2 {
              n1755 = Wait (ms)(milliseconds to wait=u32 10 ("等待时间（毫秒）")) -> ()  [unwired: 1 out]
              n1756 = call "建立数据连接.vi"("错误输入"=w3232, "端口号"=8001 ("数据端口 2"), "设备句柄入"=w3233) -> ("错误输出"=w3230:errorcluster, "设备句柄"=w3231:i32)  [unwired: 7 in]
            }
            frame #3 {
              n1757 = local write "设置开关量方向 2"(cluster{"IO1~IO8":i8, "IO9~IO16":i8} {"IO1~IO8"=1, "IO9~IO16"=1} ("设置开关量方向")) -> ()
              n1758 = call "设置开关量方向.vi"("错误输入"=w3238, "方向"=i8[] [1, 1, 1, 1], "设备句柄入"=w3239) -> ("错误输出"=w3236:errorcluster, "设备句柄"=w3237:i32)  [unwired: 7 in]
              n1759 = Wait (ms)(milliseconds to wait=u32 10 ("等待时间（毫秒）")) -> ()  [unwired: 1 out]
            }
            frame #4 {
              n1760 = local write "错误输出 6"(w3242) -> ()
              "设备句柄 2" <- w3243
            }
          }
        }
        frame #2 {
        }
      }
    }
    frame #1 {
      n1761 = local read "错误输出 6"() -> (w3244:errorcluster)
      n1762 = while {
        stop <- w3495 stop-if-true
        n1763 = local read "布尔 2"() -> (w3496:bool)
        n1764 = Wait (ms)(milliseconds to wait=u32 10 ("等待时间（毫秒）")) -> ()  [unwired: 1 out]
        n1765 = case shown="真" w3496 {
          frame False {
          }
          frame True {
            n1766 = local read "设备句柄 2"() -> (w3507:i32)
            n1767 = local read "每次总数据量 2"() -> (w3505:i32)
            n1768 = call "得到上位机软件缓冲区数据个数(M).vi"("设备句柄入"=w3507) -> ("错误输出"=w3503:errorcluster, "可读数据个数"=w3506:i32, "设备句柄"=w3504:i32)  [unwired: 8 in]
            n1769 = call <vilib>:"Clear Errors.vi"("error in (no error)"=w3503) -> ()  [unwired: 5 in, 2 out]
            n1770 = Not(x=w3503) -> (.not. x?=→"采集卡右":bool)
            n1771 = Greater Or Equal?(x=w3506, y=w3505) -> (x >= y?=w3502:bool)
            n1772 = case shown="真" w3502 {
              tunnel: w3505 -> [_ w3519]
              tunnel: w3504 -> [_ w3518]
              frame False {
              }
              frame True {
                n1773 = local read "每次总数据量 2"() -> (w3523:i32)
                n1774 = local read "通道数量 2"() -> (w3512:i32)
                n1775 = call "读取高速数据(M).vi"("数据个数"=w3519, "设备句柄入"=w3518) -> ("错误输出"=w3525:errorcluster, "返回数据个数"=w3526:i32, "原码值"=w3527:u16[], "设备句柄"=w3528:i32)  [unwired: 6 in]
                "错误输出 6" <- w3525
                n1776 = Divide(x=w3523, y=w3512) -> (x/y=w3522:dbl)
                n1777 = call "AD原码转物理.vi"("设备句柄入"=w3528, "原码值"=w3527, "个数"=w3526, "错误输入"=w3525) -> ("物理值"=w3524:dbl[])  [unwired: 4 in, 2 out]
                n1778 = To Long Integer(number=w3522) -> (32bit integer=w3521:i32)
                n1779 = Reshape Array "重排数组维数"(w3524, w3521, w3512) -> (w3520:dbl[][])
                n1780 = Transpose 2D Array(2D array=w3520) -> (transposed array=w3516:dbl[][])
                n1781 = Array Size(array=w3516) -> (size(s)=w3515:i32[])
                n1782 = for {
                  tunnel: w3516 -> [w3530] mode=indexing
                  tunnel: [w3529] -> w3517 mode=indexing
                  n1783 = Add Array Elements(numeric array=w3530) -> (sum=w3529:dbl)
                }
                n1784 = Index Array(array=w3515, index=1 ("索引")) -> (element=w3513:i32)
                n1785 = Divide(x=w3517, y=w3513) -> (x/y=w3511:dbl[])
                "AD均值数据 2" <- w3511
                n1786 = Reshape Array(w3511, 4 ("维数大小"), 8 ("维数大小")) -> (→"输出数组右":dbl[][])
              }
            }
          }
        }
        n1787 = local read "设备句柄 2"() -> (w3494:i32)
        n1788 = local read "停止"() -> (w3495:bool)
        n1789 = case shown="真" w3495 {
          tunnel: w3494 -> [_ w3498]
          frame False {
          }
          frame True {
            n1790 = flat-sequence {
              tunnel: w3498 -> [w3499]
              frame #0 {
                n1791 = call "停止采集(M).vi"("设备句柄入"=w3499) -> ()  [unwired: 9 in, 2 out]
              }
              frame #1 {
                "布尔 2" <- FALSE ("布尔")
              }
            }
          }
        }
      }
      n1792 = while {
        shift-right: [w3246] -> _
        shift-left: w3244 -> [w3247]
        stop <- w3249 stop-if-true
        n1793 = local read "设备句柄 2"() -> (w3245:i32)
        n1794 = event shown="[1] 菜单选择(用户)" {
          selector: _ -> [_ _ _ _ _ _ _ _ _ _ _ _ _ _]
          dyn-events: _ -> [_ _ _ _ _ _ _ _ _ _ _ _ _ _]
          timeout: 100 -> [_ _ _ _ _ _ _ _ _ _ _ _ _ _]
          tunnel: w3245 -> [w3269 w3301 w3343 w3348 w3364 w3397 w3419 w3424 w3434 w3455 w3470 _ w3488 w3493]
          tunnel: w3247 -> [w3268 w3300 w3345 w3347 w3363 w3396 w3418 w3423 w3433 w3454 w3469 w3473 w3487 w3492]
          tunnel: [w3253 w3299 w3344 w3346 w3362 w3372 w3411 w3422 w3432 w3436 w3464 w3473 w3486 w3490] -> w3246
          event Timeout {
            n1795 = event-data() -> ()  [unwired: 1 in, 2 out]
            n1796 = call "得到所有通道开关量值.vi"("错误输入"=w3268, "设备句柄入"=w3269) -> ("错误输出"=w3251:errorcluster, "iStatus"=w3260:i8[], "设备句柄"=w3265:i32)  [unwired: 7 in]
            "错误输出 5" <- w3251
            n1797 = Array Subset(array=w3260, index=0 ("索引"), length=16 ("长度")) -> (w3257:i8[])
            n1798 = for {
              tunnel: w3257 -> [w3289] mode=indexing
              tunnel: [w3286] -> w3256 mode=indexing
              n1799 = Equal?(x=w3289, y=i8 1) -> (x = y?=w3287:bool)
              n1800 = case shown="假" w3287 {
                tunnel: [FALSE TRUE] -> w3286
                frame False {
                }
                frame True {
                }
              }
            }
            n1801 = Array Subset(array=w3260, index=16 ("索引"), length=8 ("长度")) -> (w3259:i8[])
            n1802 = for {
              tunnel: [w3293] -> w3258 mode=indexing
              tunnel: w3259 -> [w3292] mode=indexing
              n1803 = Equal?(x=w3292, y=i8 1) -> (x = y?=w3294:bool)
              n1804 = case shown="假" w3294 {
                tunnel: [FALSE TRUE] -> w3293
                frame False {
                }
                frame True {
                }
              }
            }
            "光隔离输入 2" <- w3258
            n1805 = Array To Cluster(array=w3256) -> (cluster=→"可编程数字量I/O(映射控件)--得到所有通道开关量值 2":T22)
            n1806 = call "读取编码器.vi"("错误输入"=w3251, "设备句柄入"=w3265) -> ("错误输出"=w3255:errorcluster, "编码器过零值"=→"编码器过零值 2":i16[], "编码器AB值"=→"编码器AB值 2":i32[], "设备句柄"=w3254:i32)  [unwired: 6 in]
            n1807 = local read "开启计数 2"() -> (w3252:bool)
            n1808 = case shown="真" w3252 {
              tunnel: w3255 -> [w3270 w3278]
              tunnel: w3254 -> [_ w3277]
              tunnel: [w3270 w3276] -> w3253
              frame False {
              }
              frame True {
                n1809 = call "读取所有路计数器的原码值.vi"("错误输入"=w3278, "设备句柄入"=w3277) -> ("错误输出"=w3274:errorcluster, "计数器的原码值"=w3271:u32[], "设备句柄"=w3275:i32)  [unwired: 7 in]
                n1810 = for {
                  N: 6 -> [_]
                  tunnel: w3275 -> [w3285]
                  tunnel: w3274 -> [w3284]
                  tunnel: [w3283] -> w3276
                  tunnel: [w3280] -> w3272 mode=indexing
                  tunnel: w3271 -> [w3279] mode=indexing
                  i -> [w3282]
                  n1811 = Increment(x=w3282) -> (x+1=w3281:i32)
                  n1812 = call "计数器值转换成对应的物理值.vi"("错误输入"=w3284, "ctCode"=w3279, "chNo"=w3281, "设备句柄入"=w3285) -> ("错误输出"=w3283:errorcluster, "ctValue"=w3280:dbl)  [unwired: 5 in, 1 out]
                }
                "计数/测频（Hz）值 2" <- w3272
              }
            }
          }
          event Menu Selection (User) {
            n1813 = event-data() -> ("ItemTag"=w3298:string)  [unwired: 1 in, 6 out]
            n1814 = case shown="\"采集卡右\"" w3298 {
              tunnel: w3301 -> [_ w3304]
              tunnel: w3300 -> [_ w3303]
              tunnel: [_ w3302] -> w3299
              frame "假", Default {
              }
              frame "采集卡右" {
                n1815 = flat-sequence {
                  tunnel: w3304 -> [w3308]
                  tunnel: w3303 -> [w3307]
                  tunnel: [w3306] -> w3305
                  tunnel: [w3342] -> w3302
                  tunnel: w3305 -> [w3342]
                  frame #0 {
                    n1816 = call "AD设置范围.vi"("错误输入"=w3307, "范围"="AD范围 2", "设备句柄入"=w3308) -> ("错误输出"=w3329:errorcluster, "设备句柄"=w3328:i32)  [unwired: 7 in]
                    n1817 = call "AD设置单双端.vi"("错误输入"=w3329, "单双端"="单双端 2", "设备句柄入"=w3328) -> ("错误输出"=w3331:errorcluster, "设备句柄"=w3330:i32)  [unwired: 7 in]
                    n1818 = call "AD设置增益.vi"("错误输入"=w3331, "增益"="增益 2", "设备句柄入"=w3330) -> ("错误输出"=w3338:errorcluster, "设备句柄"=w3337:i32)  [unwired: 7 in]
                    n1819 = call "AD设置通道范围.vi"("错误输入"=w3338, "起始通道"="AD起始通道 2", "终止通道"="AD终止通道 2", "设备句柄入"=w3337) -> ("错误输出"=w3332:errorcluster, "设备句柄"=w3333:i32)  [unwired: 6 in]
                    n1820 = Subtract(x="AD终止通道 2", y="AD起始通道 2") -> (x-y=w3316:i32)
                    n1821 = Increment(x=w3316) -> (x+1=w3334:i32)
                    "通道数量 2" <- w3334
                    n1822 = call "设定通道频率.vi"("错误输入"=w3332, "通道频率"="通道频率Hz 2", "设备句柄入"=w3333) -> ("错误输出"=w3320:errorcluster, "设备句柄"=w3319:i32)  [unwired: 7 in]
                    n1823 = local read "伪同步 2"() -> (w3325:i32)
                    n1824 = case shown="0, 默认" w3325 {
                      tunnel: "通道频率Hz 2" -> [w3339 _]
                      tunnel: [w3339 w3340] -> w3311
                      tunnel: "组频率Hz 2" -> [_ w3340]
                      frame 0, Default {
                      }
                      frame 1 {
                      }
                    }
                    n1825 = call "设定组频率.vi"("错误输入"=w3320, "组频率"="组频率Hz 2", "设备句柄入"=w3319) -> ("错误输出"=w3336:errorcluster, "设备句柄"=w3335:i32)  [unwired: 7 in]
                    n1826 = Divide(x=w3311, y=2.0 ("每秒刷新数据次数")) -> (x/y=w3309:dbl)
                    n1827 = To Long Integer(number=w3309) -> (32bit integer=w3314:i32)
                    n1828 = Quotient & Remainder(x=w3314, y=w3334) -> (floor(x/y)=w3313:i32)  [unwired: 1 out]
                    "每通道数据量 2" <- w3313
                    n1829 = Multiply(x=w3313, y=w3334) -> (x*y=→"每次总数据量 2":i32)
                    n1830 = call "启动采集(M系列).vi"("错误输入"=w3336, "时钟源"="时钟源 2", "伪同步"="伪同步 2", "设备句柄入"=w3335) -> ("错误输出"=w3306:errorcluster)  [unwired: 6 in, 1 out]
                  }
                  frame #1 {
                    n1831 = local write "布尔 2"(TRUE ("布尔")) -> ()
                  }
                }
              }
            }
          }
          event "AD停止采集 2": Value Change {
            n1832 = event-data() -> ()  [unwired: 1 in, 5 out]
            n1833 = call "停止采集(M).vi"("错误输入"=w3345, "设备句柄入"=w3343) -> ("错误输出"=w3344:errorcluster)  [unwired: 8 in, 1 out]
          }
          event "开启计数 2": Value Change {
            n1834 = event-data() -> ()  [unwired: 1 in, 5 out]
            n1835 = Initialize Array("工作方式 2", 6 ("维数大小")) -> (w3352:u16[])
            n1836 = call "设置所有路计数器的工作方式.vi"("错误输入"=w3347, "ctMode"=w3352, "设备句柄入"=w3348) -> ("错误输出"=w3351:errorcluster, "设备句柄"=w3350:i32)  [unwired: 7 in]
            n1837 = for {
              N: 6 -> [_]
              tunnel: w3351 -> [w3360]
              tunnel: w3350 -> [w3359]
              tunnel: [w3355] -> w3346
              i -> [w3357]
              n1838 = Increment(x=w3357) -> (x+1=w3356:i32)
              n1839 = call "设置指定通道的测频基准脉冲周期.vi"("错误输入"=w3360, "freqBase_ms"=1000.0, "chNo"=w3356, "设备句柄入"=w3359) -> ("错误输出"=w3355:errorcluster)  [unwired: 5 in, 2 out]
            }
          }
          event "计数器清零 2": Value Change {
            n1840 = event-data() -> ()  [unwired: 1 in, 5 out]
            n1841 = for {
              N: 6 -> [_]
              tunnel: w3364 -> [w3369]
              tunnel: w3363 -> [w3368]
              tunnel: [w3367] -> w3362
              i -> [w3366]
              n1842 = Increment(x=w3366) -> (x+1=w3365:i32)
              n1843 = call "指定通道计数器清零.vi"("错误输入"=w3368, "chNo"=w3365, "设备句柄入"=w3369) -> ("错误输出"=w3367:errorcluster)  [unwired: 7 in, 1 out]
            }
          }
          event "PWM输出 2": Value Change {
            n1844 = event-data() -> ("OldVal"=w3370:bool)  [unwired: 1 in, 4 out]
            n1845 = local write "PWM输出 2"(w3370) -> ()
            n1846 = call "设置开关量方向.vi"("错误输入"=w3396, "方向"=i8[] [1, 1], "设备句柄入"=w3397) -> ("错误输出"=w3394:errorcluster, "设备句柄"=w3395:i32)  [unwired: 7 in]
            n1847 = call "设置PWM频率和占空比.vi"("占空比(0~1)"="占空比(0~1) 6", "频率"="频率1 2", "错误输入"=w3394, "通道号"=1, "设备句柄入"=w3395) -> ("错误输出"=w3386:errorcluster, "设备句柄"=w3380:i32, "实际占空比"=→"实际占空比 6":dbl, "实际频率"=→"实际频率 6":dbl)  [unwired: 3 in]
            n1848 = call "设置PWM频率和占空比.vi"("占空比(0~1)"="占空比(0~1) 5", "频率"="频率2 2", "错误输入"=w3386, "通道号"=2, "设备句柄入"=w3380) -> ("错误输出"=w3379:errorcluster, "设备句柄"=w3381:i32, "实际占空比"=→"实际占空比 5":dbl, "实际频率"=→"实际频率 5":dbl)  [unwired: 3 in]
            n1849 = call "设置PWM频率和占空比.vi"("占空比(0~1)"="占空比(0~1) 4", "频率"="频率3 2", "错误输入"=w3379, "通道号"=3, "设备句柄入"=w3381) -> ("错误输出"=w3373:errorcluster, "设备句柄"=w3374:i32, "实际占空比"=→"实际占空比 4":dbl, "实际频率"=→"实际频率 4":dbl)  [unwired: 3 in]
            n1850 = call "使能或禁止PWM输出.vi"("错误输入"=w3373, "所用PWM使能"=i8 1, "设备句柄入"=w3374) -> ("错误输出"=w3372:errorcluster)  [unwired: 7 in, 1 out]
          }
          event "M系列PWM输出 2": Value Change {
            w3406 = 2 ("通道号")
            w3401 = 0.5 ("占空比(0~1)")
            w3402 = 2000.0 ("频率")
            w3414 = 1 ("通道号")
            n1851 = event-data() -> ()  [unwired: 1 in, 5 out]
            n1852 = call "设置开关量方向.vi"("错误输入"=w3418, "方向"=i8[] [1, 1], "设备句柄入"=w3419) -> ("错误输出"=w3416:errorcluster, "设备句柄"=w3417:i32)  [unwired: 7 in]
            n1853 = call "设置PWM频率和占空比.vi"("占空比(0~1)"=w3401, "频率"=w3402, "错误输入"=w3416, "通道号"=w3414, "设备句柄入"=w3417) -> ("错误输出"=w3412:errorcluster, "设备句柄"=w3415:i32)  [unwired: 3 in, 2 out]
            n1854 = call "设定输出脉冲个数.vi"("错误输入"=w3412, "脉冲个数"="设定输出脉冲个数 2", "通道号"=w3414, "设备句柄入"=w3415) -> ("错误输出"=w3404:errorcluster, "设备句柄"=w3403:i32)  [unwired: 2 in]
            n1855 = call "设置PWM频率和占空比.vi"("占空比(0~1)"=w3401, "频率"=w3402, "错误输入"=w3404, "通道号"=w3406, "设备句柄入"=w3403) -> ("错误输出"=w3405:errorcluster, "设备句柄"=w3407:i32)  [unwired: 3 in, 2 out]
            n1856 = call "设定输出脉冲个数.vi"("错误输入"=w3405, "通道号"=w3406, "设备句柄入"=w3407) -> ("错误输出"=w3399:errorcluster, "设备句柄"=w3400:i32)  [unwired: 3 in]
            n1857 = call "使能或禁止PWM输出(只支持EM9636M).vi"("错误输入"=w3399, "相位设置数组"=i8[] [1, 0, 0] ("PWM使能"), "PWM使能"=i8[] [1, 1, 0], "设备句柄入"=w3400) -> ("错误输出"=w3411:errorcluster)  [unwired: 6 in, 1 out]
          }
          event "设置开关量方向 3": Value Change {
            n1858 = event-data() -> ()  [unwired: 1 in, 5 out]
            n1859 = Cluster To Array(cluster="设置开关量方向 2") -> (array=w3420:i8[])
            "数组 7" <- w3420
            n1860 = call "设置开关量方向.vi"("错误输入"=w3423, "方向"=w3420, "设备句柄入"=w3424) -> ("错误输出"=w3422:errorcluster)  [unwired: 7 in, 1 out]
          }
          event "光隔离输出 2", "可编程数字量I/O 2": Value Change {
            n1861 = event-data() -> ()  [unwired: 1 in, 5 out]
            n1862 = local read "光隔离输入 2"() -> (w3431:bool[])
            n1863 = Cluster To Array(cluster="可编程数字量I/O 2") -> (array=w3425:bool[])
            n1864 = Build Array (concatenate)(w3425, w3431, "光隔离输出 2") -> (w3429:bool[])
            n1865 = Boolean To (0,1)(Boolean=w3429) -> (0, 1=w3428:i16[])
            n1866 = To Byte Integer(number=w3428) -> (8bit integer=w3427:i8[])
            n1867 = call "设置所有通道开关量值.vi"("错误输入"=w3433, "oStatus"=w3427, "设备句柄入"=w3434) -> ("错误输出"=w3432:errorcluster)  [unwired: 7 in, 1 out]
          }
          event "DA输出 2", "CH1 2", "CH2 2", "CH3 2", "CH4 2": Value Change {
            n1868 = event-data() -> ()  [unwired: 1 in, 5 out]
            n1869 = for {
              N: 4 -> [_]
              tunnel: w3455 -> [w3463]
              tunnel: w3454 -> [w3462]
              tunnel: "DA输出范围 2" -> [w3458]
              tunnel: [w3457] -> w3452
              tunnel: [w3456] -> w3451
              i -> [w3460]
              n1870 = Increment(x=w3460) -> (x+1=w3461:i32)
              n1871 = call "DA输出方式.vi"("输出范围"=w3458, "错误输入"=w3462, "输出值方式"=i16 1, "通道号"=w3461, "设备句柄入"=w3463) -> ("错误输出"=w3457:errorcluster, "设备句柄"=w3456:i32)  [unwired: 5 in]
            }
            n1872 = call "设置DA输出值.vi"("错误输入"=w3452, "输出值"="CH1 2", "通道号"=1, "设备句柄入"=w3451) -> ("错误输出"=w3445:errorcluster, "设备句柄"=w3447:i32)  [unwired: 6 in]
            n1873 = call "设置DA输出值.vi"("错误输入"=w3445, "输出值"="CH2 2", "通道号"=2, "设备句柄入"=w3447) -> ("错误输出"=w3439:errorcluster, "设备句柄"=w3444:i32)  [unwired: 6 in]
            n1874 = call "设置DA输出值.vi"("错误输入"=w3439, "输出值"="CH3 2", "通道号"=3, "设备句柄入"=w3444) -> ("错误输出"=w3438:errorcluster, "设备句柄"=w3443:i32)  [unwired: 6 in]
            n1875 = call "设置DA输出值.vi"("错误输入"=w3438, "输出值"="CH4 2", "通道号"=4, "设备句柄入"=w3443) -> ("错误输出"=w3436:errorcluster)  [unwired: 6 in, 1 out]
          }
          event "编码器清零 2": Value Change {
            n1876 = event-data() -> ()  [unwired: 1 in, 5 out]
            n1877 = call "编码器清零.vi"("错误输入"=w3469, "通道号"=1, "设备句柄入"=w3470) -> ("错误输出"=w3465:errorcluster, "设备句柄"=w3466:i32)  [unwired: 7 in]
            n1878 = call "编码器清零.vi"("错误输入"=w3465, "通道号"=2, "设备句柄入"=w3466) -> ("错误输出"=w3464:errorcluster)  [unwired: 7 in, 1 out]
          }
          event "DA输出范围 2": Value Change {
            n1879 = event-data() -> ()  [unwired: 1 in, 5 out]
            n1880 = local read "DA输出范围 2"() -> (w3474:i32)
            n1881 = case shown="4" w3474 {
              tunnel: [10000.0 ("标尺.范围:最大值") 5000.0 ("标尺.范围:最大值") 10000.0 ("标尺.范围:最大值") 5000.0 ("标尺.范围:最大值") 20000.0 ("标尺.范围:最大值")] -> w3472
              tunnel: [-10000.0 ("标尺.范围:最大值") -5000.0 ("标尺.范围:最大值") 0.0 ("标尺.范围:最大值") 0.0 ("标尺.范围:最大值") 0.0 ("标尺.范围:最大值")] -> w3471
              frame 0, Default {
              }
              frame 1 {
              }
              frame 2 {
              }
              frame 3 {
              }
              frame 4 {
              }
            }
            n1882 = property on="CH1 2" class="Slide (严格)"("Scale.Maximum"=w3472, "Scale.Minimum"=w3471) -> ()  [unwired: 2 in, 2 out]
            n1883 = property on="CH2 2" class="Slide (严格)"("Scale.Maximum"=w3472, "Scale.Minimum"=w3471) -> ()  [unwired: 2 in, 2 out]
            n1884 = property on="CH3 2" class="Slide (严格)"("Scale.Maximum"=w3472, "Scale.Minimum"=w3471) -> ()  [unwired: 2 in, 2 out]
            n1885 = property on="CH4 2" class="Slide (严格)"("Scale.Maximum"=w3472, "Scale.Minimum"=w3471) -> ()  [unwired: 2 in, 2 out]
          }
          event "M系列PWM停止 2": Value Change {
            n1886 = event-data() -> ()  [unwired: 1 in, 5 out]
            n1887 = call "使能或禁止PWM输出(只支持EM9636M).vi"("错误输入"=w3487, "相位设置数组"=i8[] [0, 0, 0] ("PWM使能"), "PWM使能"=i8[] [0, 0, 0], "设备句柄入"=w3488) -> ("错误输出"=w3486:errorcluster)  [unwired: 6 in, 1 out]
          }
          event "PWM停止 2": Value Change {
            n1888 = event-data() -> ()  [unwired: 1 in, 5 out]
            n1889 = call "使能或禁止PWM输出.vi"("错误输入"=w3492, "所用PWM使能"=i8 0, "设备句柄入"=w3493) -> ("错误输出"=w3490:errorcluster)  [unwired: 7 in, 1 out]
          }
        }
        "错误输出 4" <- w3246
        n1890 = local read "停止"() -> (w3249:bool)
      }
    }
    frame #2 {
      n1891 = flat-sequence {
        tunnel: [w3541] -> w3537
        tunnel: [w3539] -> w3536
        tunnel: w3537 -> [w3547]
        tunnel: [w3546] -> w3535
        tunnel: w3536 -> [w3545]
        tunnel: [w3544] -> w3534
        tunnel: w3535 -> [w3553]
        tunnel: [w3552] -> w3533
        tunnel: w3534 -> [w3551]
        tunnel: [w3550] -> w3532
        tunnel: w3533 -> [w3558]
        tunnel: [w3557] -> w3531
        tunnel: w3532 -> [w3556]
        tunnel: w3531 -> [w3559]
        frame #0 {
          n1892 = local read "设备句柄 2"() -> (w3542:i32)
          n1893 = local read "错误输出 6"() -> (w3540:errorcluster)
          n1894 = call "停止采集(M).vi"("错误输入"=w3540, "设备句柄入"=w3542) -> ("错误输出"=w3539:errorcluster, "设备句柄"=w3541:i32)  [unwired: 8 in]
          n1895 = Wait (ms)(milliseconds to wait=u32 10 ("等待时间（毫秒）")) -> ()  [unwired: 1 out]
        }
        frame #1 {
          n1896 = call "使能或禁止PWM输出.vi"("错误输入"=w3545, "所用PWM使能"=i8 0, "设备句柄入"=w3547) -> ("错误输出"=w3544:errorcluster, "设备句柄"=w3546:i32)  [unwired: 7 in]
          n1897 = Wait (ms)(milliseconds to wait=u32 10 ("等待时间（毫秒）")) -> ()  [unwired: 1 out]
        }
        frame #2 {
          n1898 = call "关闭数据连接.vi"("错误输入"=w3551, "设备句柄入"=w3553) -> ("错误输出"=w3550:errorcluster, "设备句柄"=w3552:i32)  [unwired: 8 in]
          n1899 = Wait (ms)(milliseconds to wait=u32 10 ("等待时间（毫秒）")) -> ()  [unwired: 1 out]
        }
        frame #3 {
          n1900 = call "关闭命令连接.vi"("错误输入"=w3556, "设备句柄入"=w3558) -> ("错误输出"=w3555:errorcluster, "设备句柄"=w3557:i32)  [unwired: 8 in]
          n1901 = Wait (ms)(milliseconds to wait=u32 10 ("等待时间（毫秒）")) -> ()  [unwired: 1 out]
          n1902 = local write "错误输出 6"(w3555) -> ()
        }
        frame #4 {
          n1903 = call "关闭设备.vi"("设备句柄"=w3559) -> ()  [unwired: 10 in]
        }
        frame #5 {
          "close2" <- TRUE ("close2")
        }
      }
    }
  }
  n1904 = local read "平均速度数组"() -> (w15:dbl[])
  n1905 = local read "D1平均速度"() -> (w16:dbl)
  n1906 = Build Array (concatenate)(w15, w16) -> (→"平均速度数组":dbl[])
  n1907 = disable-structure shown="启用" {
    disable-tunnel: w26 -> [w3562 _]
    disable-tunnel: 0 -> [w3561 _]
    frame Disabled {
      n1908 = while "数据更新线程" {
        tunnel: w3562 -> [w3576]
        shift-right: [w3567] -> _
        shift-left: _ -> [w3572]
        shift-right: [w3568] -> _
        shift-left: w3561 -> [w3571]
        stop <- w3574 stop-if-true
        n1909 = Dequeue Element(queue=w3576, timeout in ms (-1)=5 ("超时毫秒(-1)")) -> (element=w3573:T13, timed out?=w3566:bool, error out=w3574:errorcluster)  [unwired: 1 in, 1 out]
        n1910 = case shown="假" w3566 {
          tunnel: w3573 -> [w3587 _]
          tunnel: w3572 -> [w3590 w3598]
          tunnel: [w3583 w3598] -> w3570
          tunnel: w3571 -> [w3586 w3597]
          tunnel: [w3584 w3597] -> w3569
          frame False {
            n1911 = Insert Into Array(array=w3590, new element=w3587) -> (w3588:T13)  [unwired: 1 in]
            n1912 = Array Size(array=w3588) -> (size(s)=w3589:i32)
            n1913 = case "最多保存500帧" shown="501.." w3589 {
              selector: w3589 -> [_ w3595]
              tunnel: w3588 -> [w3591 w3596]
              tunnel: [w3591 w3593] -> w3583
              tunnel: [_ w3592] -> w3585
              frame 0, Default {
              }
              frame 501.. {
                n1914 = Subtract(x=w3595, y=500) -> (x-y=w3592:i32)
                n1915 = Array Subset(array=w3596, index=w3592) -> (w3593:T13)  [unwired: 1 in]
              }
            }
            n1916 = Add(x=w3586, y=w3585) -> (x+y=w3584:i32)
          }
          frame True {
          }
        }
        n1917 = Not(x=w3566) -> (.not. x?=w3565:bool)
        n1918 = case shown="真" "Clear" {
          tunnel: w3569 -> [w3581 _]
          tunnel: w3570 -> [w3582 _]
          tunnel: [w3582 _] -> w3567
          tunnel: [w3581 _] -> w3568
          frame False {
          }
          frame True {
          }
        }
        n1919 = Or(x="Clear", y=w3565) -> (x .or. y?=w3564:bool)
        n1920 = case shown="真" w3564 {
          tunnel: w3568 -> [_ w3578]
          tunnel: w3567 -> [_ w3577]
          frame False {
          }
          frame True {
            n1921 = control-ref of="本VI"() -> (w3579:refnum<vi>)
            n1922 = control-ref of="list"() -> (w3580:refnum<vi>)
            n1923 = call "Demo_UpdateList.vi"("Offset"=w3578, "Buffer"=w3577, "list"=w3580, "MainVi"=w3579) -> ()  [unwired: 8 out]
          }
        }
      }
    }
    frame Enabled {
    }
  }
  n1924 = while "接收线程" {
    tunnel: w26 -> [w3605]
    shift-right: [w3603] -> _
    shift-left: u32 0 ("RecvCnt") -> [w3604]
    shift-right: [w3601] -> _
    shift-left: "" ("档位") -> [w3602]
    stop <- w3600 stop-if-true
    n1925 = local read "Open"() -> (w3606:bool)
    n1926 = case shown="真" w3606 {
      tunnel: w3605 -> [_ w3616]
      tunnel: w3604 -> [w3608 w3615]
      tunnel: [w3608 w3614] -> w3603
      tunnel: w3602 -> [w3607 w3611]
      tunnel: [w3607 w3610] -> w3601
      frame False {
        # "CAN未打开，延时50ms"
        n1927 = Wait (ms)(milliseconds to wait=u32 50 ("等待时间（毫秒）")) -> ()  [unwired: 1 out]
      }
      frame True {
        n1928 = local read "DevType"() -> (w3619:T3)
        n1929 = local read "Channel"() -> (w3613:T4)
        n1930 = call "VCI_Receive.vi"("CANIndex"=w3613, "DevIndex"=u32 0, "DevType"=w3619) -> ("Recieve"=w3612:T12[])  [unwired: 3 in, 5 out]
        n1931 = Empty Array?(array=w3612) -> (empty?=w3617:bool)
        n1932 = case shown="假" w3617 {
          tunnel: w3616 -> [w3632 _]
          tunnel: w3612 -> [w3624 _]
          tunnel: [w3629 _] -> _
          tunnel: w3615 -> [w3627 w3651]
          tunnel: [w3626 w3651] -> w3614
          tunnel: w3613 -> [w3625 _]
          tunnel: w3611 -> [w3623 w3650]
          tunnel: [w3622 w3650] -> w3610
          frame False {
            n1933 = Array Size(array=w3624) -> (size(s)=w3628:i32)
            n1934 = call "Demo_MakeDispBuff.vi"("Channel"=w3625, "Type"=enum16{"接收", "发送"}."接收", "OBJs"=w3624) -> ("Buffer"=w3630:T13)
            n1935 = Add(x=w3628, y=w3627) -> (x+y=w3626:u32)
            "RecvCnt" <- w3626
            n1936 = for {
              tunnel: w3624 -> [w3640] mode=indexing
              tunnel: w3623 -> [w3637]
              tunnel: [w3636] -> w3622
              n1937 = Unbundle By Name(w3640) -> ("ID"=w3639:u32, "Data"=w3638:u8[])
              n1938 = case shown="18A" w3639 {
                tunnel: w3638 -> [_ w3646]
                tunnel: w3637 -> [w3641 _]
                tunnel: [w3641 _] -> w3636
                frame 0, Default {
                }
                frame 394 {
                  n1939 = Index Array(array=w3646) -> (element #3=w3645:u8, element #4=w3644:u8)  [unwired: 6 in, 4 out]
                  n1940 = Number To Boolean Array(number=w3644) -> (Boolean array=→"布尔数组 2":bool[])
                  n1941 = Number To Boolean Array(number=w3645) -> (Boolean array=→"布尔数组":bool[])
                }
              }
            }
            n1942 = disable-structure shown="禁用" {
              disable-tunnel: w3632 -> [w3635 _]
              disable-tunnel: w3630 -> [w3634 _]
              disable-tunnel: [w3633 _] -> w3629
              frame Disabled {
                n1943 = Enqueue Element(queue=w3635, element=w3634) -> (error out=w3633:errorcluster)  [unwired: 1 in, 3 out]
              }
              frame Enabled {
              }
            }
            n1944 = local write "comcnt"(u16 0 ("comcnt")) -> ()
            "遥控器通讯" <- FALSE ("遥控器通讯")
          }
          frame True {
            n1945 = local write "遥控器通讯"(TRUE ("遥控器通讯")) -> ()
            n1946 = property on="comcnt" class="DigNum (严格)"() -> ("Value"=w3647:u16)  [unwired: 2 in, 2 out]
            n1947 = Increment(x=w3647) -> (x+1=→"comcnt":u16)
          }
        }
      }
    }
    n1948 = local read "停止"() -> (w3600:bool)
    n1949 = Wait (ms)(milliseconds to wait=u32 50 ("等待时间（毫秒）")) -> ()  [unwired: 1 out]
  }
  n1950 = Release Queue(queue=w11) -> ()  [unwired: 2 in, 3 out]
  n1951 = disable-structure shown="禁用" {
    disable-tunnel: w4 -> [w3653 _]
    frame Disabled {
      n1952 = control-ref of="本应用程序"() -> (w3655:refnum<vi>)
      n1953 = invoke class="VI" method="FP.Close"(error in=w3653) -> (error out=w3652:errorcluster)  [unwired: 2 in, 2 out]
      n1954 = property class="App"(reference=w3655) -> ("App.Kind"=w3654:T19)  [unwired: 1 in, 2 out]
      n1955 = case shown="\"Development System\"" w3654 {
        tunnel: w3652 -> [_ _]
        frame "invalid app kind", Default {
          n1956 = Quit LabVIEW() -> ()  [unwired: 1 out]
        }
        frame "Development System" {
        }
      }
    }
    frame Enabled {
    }
  }
  n1957 = while {
    stop <- w3663 stop-if-true
    n1958 = local read "对话框"() -> (w3656:bool)
    n1959 = local read "到期了"() -> (w3660:bool)
    n1960 = call "初始化.vi"() -> ("first row"=w3664:dbl[], "最终选择的真实日期"=w3665:dbl[], "密码"=w3666:string[][])  [unwired: 3 in]
    n1961 = case shown="真" w3656 {
      frame False {
      }
      frame True {
        n1962 = flat-sequence {
          frame #0 {
            n1963 = One Button Dialog(message="试用期已到，电机将无法加载，请输入密码" ("消息")) -> ()  [unwired: 1 in, 1 out]
          }
          frame #1 {
            n1964 = local write "对话框"(FALSE ("对话框")) -> ()
          }
        }
      }
    }
    n1965 = case shown="真" w3660 {
      frame False {
        n1966 = property on="密码输入" class="Str"("Visible"=FALSE ("可见")) -> ()  [unwired: 2 in, 2 out]
      }
      frame True {
        w3671 = i16 0 ("驱动电机转速下给定")
        n1967 = property on="密码输入" class="Str"("Visible"=TRUE ("可见")) -> ()  [unwired: 2 in, 2 out]
        n1968 = local write "加载电机左下转矩给定"(w3671) -> ()
        n1969 = local write "加载电机右下转矩给定"(w3671) -> ()
        n1970 = local write "加载电机右上转矩给定"(w3671) -> ()
        n1971 = local write "驱动电机上转速给定"(w3671) -> ()
        n1972 = local write "驱动电机转速下给定"(w3671) -> ()
        n1973 = local write "加载电机左上转矩给定"(w3671) -> ()
      }
    }
    n1974 = Wait (ms)(milliseconds to wait=u32 500 ("等待时间（毫秒）")) -> ()  [unwired: 1 out]
    n1975 = call "到期.vi"("最终选择的真实的日期"=w3665, "加期限后的日期"=w3664, "密码和期限"=w3666, "密码输入"="密码输入") -> ("到期了"=w3659:bool)  [unwired: 1 out]
    "到期了" <- w3659
    n1976 = call <vilib>:"Boolean Crossing PtByPt.vi"("direction"=enum16{"either", "false-true", "true-false"}."false-true", "input"=w3659) -> ("crossing"=w3657:bool)  [unwired: 1 in]
    n1977 = case shown="真" w3657 {
      frame False {
      }
      frame True {
        "对话框" <- TRUE ("对话框")
      }
    }
    n1978 = local read "停止"() -> (w3663:bool)
  }
  n1979 = while {
    stop <- FALSE stop-if-true
    n1980 = local read "close2"() -> (w3675:bool)
    n1981 = local read "close"() -> (w3676:bool)
    n1982 = And(x=w3676, y=w3675) -> (x .and. y?=w3674:bool)
    n1983 = case shown="真" w3674 {
      frame False {
      }
      frame True {
        n1984 = flat-sequence {
          frame #0 {
            w3686 = FALSE ("close")
            n1985 = local read "Config"() -> (w3685:T9)
            n1986 = local write "close"(w3686) -> ()
            n1987 = local write "close2"(w3686) -> ()
            n1988 = Unbundle By Name(w3685) -> ("DevType"=w3684:T3, "DevIndex"=w3683:u32)
            n1989 = call "VCI_CloseDevice.vi"("DevIndex"=w3683, "DevType"=w3684) -> ()  [unwired: 1 in, 9 out]
            n1990 = Wait (ms)(milliseconds to wait=u32 50 ("等待时间（毫秒）")) -> ()  [unwired: 1 out]
          }
          frame #1 {
            n1991 = Stop(stop? (T)=TRUE ("停止？(T)")) -> ()
          }
        }
      }
    }
    n1992 = local read "对话框传递"() -> (w3673:bool)
    n1993 = Wait (ms)(milliseconds to wait=u32 5 ("等待时间（毫秒）")) -> ()  [unwired: 1 out]
    n1994 = case shown="真" w3673 {
      frame False {
      }
      frame True {
        n1995 = One Button Dialog(message="温度超过70℃\n请选择查看数据菜单确认" ("消息")) -> (true=w3680:bool)  [unwired: 1 in]
        n1996 = Not(x=w3680) -> (.not. x?=w3679:bool)
        n1997 = local write "对话框传递"(w3679) -> ()
      }
    }
  }
  n1998 = call-dynamic "Close.vi"("error in (no error)"=w25, "Modbus master in"=w24) -> ("error out"=w9:errorcluster)  [unwired: 9 in]
  n1999 = call <vilib>:"Clear Errors.vi"("error in (no error)"=w9) -> ()  [unwired: 5 in, 2 out]
